vi "Surviv_io.vi"() -> ()   [LabVIEW 2021]
uses:
  <vilib>/Utility/miscctls.llb/LVPositionTypeDef.ctl
  b365312c-386e-413b-b974-73f95af02f70.vi
  <vilib>/Utility/miscctls.llb/LVComboBoxStrsAndValuesArrayTypeDef.ctl
  <vilib>/Utility/inputDevices.llb/closeMouse.vi
  <vilib>/Utility/inputDevices.llb/closeKeyboard.vi
  <vilib>/Utility/inputDevices.llb/mouseAcquire.vi
  <vilib>/Utility/inputDevices.llb/keyboardAcquire.vi
  <vilib>/Utility/file.llb/Read Delimited Spreadsheet (DBL).vi
  <vilib>/Utility/file.llb/Write Delimited Spreadsheet (DBL).vi
  <vilib>/sound2/lvsound2.llb/Sound Output Set Volume (Single).vi
panel:
  out "Data length":i32
  out "NetPlayer Commend":T1(array[cluster])
  out "My NetPlayer number":i32
  out "Connecting....":bool caption="Connecting..."
  out "NetPlayer":cluster{"Name":string, "IP Address":u32}[](array[cluster])
  in  "創建遊戲":bool
  in  "加入遊戲":bool
  out "Network Game":bool
  in  "選擇網路介面:":string(combo)="192.168.56.1"
  out "Background music":dbl
  out "Final Winner":string
  out "Enemy on 8 directions":T2
  out "Farther Bullets on 8 directions":T2
  out "Closer Bullets on 8 directions":T2
  out "Object on 8 directions":T2
  out "Closest valid target":T3
  out "Current Player HP":dbl
  out "Player HP Healing (And visibility)":i32[](array[numeric])
  out "Alive number":i32
  out "MP HP":dbl(slide) scale=0.0..290.0
  out "Input detect frequency (Hz)":dbl
  out "Sent command":T4(array[cluster])
  out "MainPlayer":T5
  out "Movement":dbl
  out "Theta":dbl
  out "Object number":i32
  out "Player Bullets Reload":i32[](array[numeric])
  out "Player Bullets":i32[](array[numeric])
  out "Frame Number":i32
  out "Player info":T6(array[cluster])
  out "Physic Engine frequency (Hz)":dbl
  out "Color 2":u32(colorbox)
  out "Color":u32(colorbox)
  out "MO ID":i32
  out "Moving Entity Position":T7(array[cluster])
  in  "進入遊戲":bool
  out "Map Entity Object Position":T8(array[cluster])
  in  "地圖:":string(combo) caption="Combo Box"
  in  "電腦代打模式:\n(Based on Machine Learning)\n(Behavior cloning)\n(Warning: High computing workload)":bool
  in  "初級電腦玩家人數:":i32 min=0 max=0 step=1
  in  "普通電腦玩家人數:":i32=1 min=0 max=19 step=1
  in  "Host IP: (Local Network)":string
  in  "玩家ID: (創建遊戲)":string
  in  "玩家ID: (加入遊戲)":string
  in  "Close (Main UI)":bool
  out "State":i32
  in  "Customized Game Button":bool
  in  "Join/Create Room Button":bool
  in  "Game Instruction Button":bool
  in  "Game Start Button":bool
  out "FPS":dbl
  in  "STOP (會卡住)":bool
  out "已加入的玩家:":string[](array[string])
  out "PlayingScene":picture
  # "若要遊玩網路遊戲，請至遊戲資料夾，目錄\\Game\\cmd\\Firewall.bat，點選\"以管理員身分執行\"，以打開防火牆設定，連線雙方均須打開請確保兩位玩家 在同一 Local Network 內 (如: 兩筆電連到同一個手機熱點)，並且在遊戲選單選擇對應的網卡介面，方可連上遊玩!"
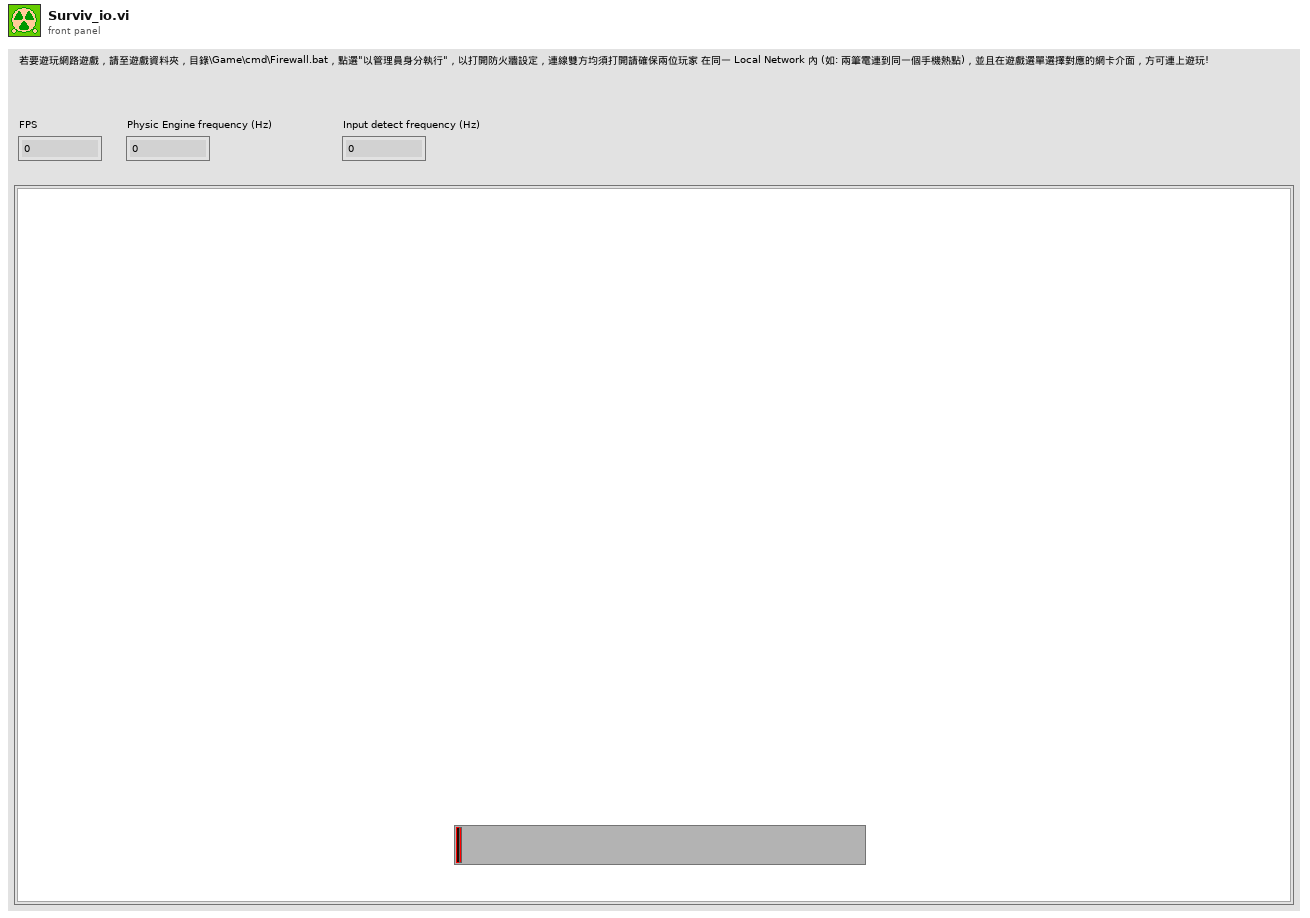
[diagram p1: front panel]
types:
  T1 = cluster{"Vector scalar":sgl, "Vector theta":sgl, "Mouse theta":sgl, "Mouse Shoot":sgl, "Reload R":sgl}[]
  T2 = cluster{"D1":dbl, "D2":dbl, "D3":dbl, "D4":dbl, "D5":dbl, "D6":dbl, "D7":dbl, "D8":dbl}
  T3 = cluster{"Theta (toward that target)":dbl, "Distance (toward that target)":dbl, "Reachable":bool}
  T4 = cluster{"X":dbl, "Y":dbl, "Object type":dbl, "Move info":dbl, "Vector scalar":dbl, "Theta":dbl}[]
  T5 = cluster{"X":dbl, "Y":dbl, "Object type":dbl, "Radius":dbl, "Width":dbl, "Height":dbl, "Theta":dbl, "HP":dbl, "R":dbl, "G":dbl, "B":dbl}
  T6 = cluster{"Kills":dbl, "Name":string, "Rank":dbl, "Who Kill Me":dbl, "After Kill":dbl}[]
  T7 = cluster{"X":dbl, "Y":dbl, "Object type":dbl, "Move info":dbl, "Vector scalar":dbl, "Vector theta":dbl}[]
  T8 = cluster{"X":dbl, "Y":dbl, "Object type":dbl, "Radius":dbl, "Width":dbl, "Height":dbl, "Theta":dbl, "HP":dbl, "R":dbl, "G":dbl, "B":dbl}[]
  T9 = typedef "LVComboBoxStrsAndValuesArrayTypeDef.ctl" = cluster{"String":string, "Value":string}[]
  T10 = enum8{"Enabled", "Disabled", "Disabled and Grayed Out"}
  T11 = cluster{"left":i16, "top":i16, "right":i16, "bottom":i16}
  T12 = typedef "LVPositionTypeDef.ctl" = cluster{"Left":i32, "Top":i32}
  T13 = enum16{"User-specified Font", "Application Font", "System Font", "Dialog Font"}
  T14 = cluster{"Font Name:":string, "Size":i16, "Strikeout?":bool, "Italic?":bool, "Underline?":bool, "Outline?":bool, "Shadow?":bool, "Bold?":bool}
  T15 = cluster{"horizontal":enum16{"left", "center", "right"}, "vertical":enum16{"top", "center", "bottom"}}
  T16 = enum16{"None", "Stacked", "Clockwise", "Counterclockwise"}
  T17 = cluster{"初級電腦玩家人數: ":i32, "普通電腦玩家人數: ":i32, "地圖:":string, "已加入的玩家:":string[]}
  T18 = typedef "Sound Output Task ID.ctl" = u32
  T19 = cluster{"Vector scalar":sgl, "Vector theta":sgl, "Mouse theta":sgl, "Mouse Shoot":sgl, "Reload R":sgl, "Reload R 2":sgl}
  T20 = cluster{dbl, "玩家ID: (加入遊戲)":string, dbl, dbl, dbl}
  T21 = cluster{"[0]":dbl, "[1]":dbl, "[2]":dbl, "[3]":dbl, "[4]":dbl, "[5]":dbl, "[6]":dbl, "[7]":dbl, "[8]":dbl, "[9]":dbl, "[10]":dbl}
  T22 = cluster{"[0]":dbl, "[1]":dbl, "[2]":dbl, "[3]":dbl, "[4]":dbl, "[5]":dbl, "[6]":dbl, "[7]":dbl, "[8]":dbl, "[9]":dbl, "[10]":dbl}[]
  T23 = cluster{"Kills":dbl, "玩家ID: (加入遊戲)":string, "Rank":dbl, "Who Kill Me":dbl, "After Kill":dbl}[]
  T24 = cluster{"X":dbl, "Y":dbl, "Object type":dbl, "Move info":dbl, "Vector scalar":dbl, "Vector theta":dbl}
  T25 = cluster{dbl, dbl, "Object type":dbl, "Move info":dbl, "Vector scalar":dbl, "Vector theta":dbl}
  T26 = cluster{"Kills":dbl, "Name":string, "Rank":dbl, "Who Kill Me":dbl, "After Kill":dbl}
  T27 = cluster{dbl, "Name":string, "Rank":dbl, "Who Kill Me":dbl, "After Kill":dbl}
  T28 = cluster{"Kills":dbl, "Name":string, "Alive number":i32, dbl, "y":dbl}
  T29 = cluster{"X":dbl, "Y":dbl, "Object type":dbl, "Radius":dbl, "Width":dbl, "Height":dbl, "Theta":dbl, dbl, "R":dbl, "G":dbl, "B":dbl}
  T30 = cluster{"New Vector Scalar":dbl, "New Vector Theta":dbl}
  T31 = cluster{dbl, dbl, "Object type":dbl, "Radius":dbl, "Width":dbl, "Height":dbl, "Move info":dbl, "HP":dbl, "R":dbl, "G":dbl, "B":dbl}
  T32 = cluster{"X":dbl, "Y":dbl, "Object type":dbl, "Radius":dbl, "y":dbl, "Height":dbl, "Theta":dbl, "HP":dbl, "R":dbl, "G":dbl, "B":dbl}
  T33 = cluster{"X":dbl, "Y":dbl, "Object type":dbl, "Radius":dbl, "y":dbl, "Height":dbl, "Theta":dbl, dbl, "R":dbl, "G":dbl, "B":dbl}
  T34 = cluster{"X":dbl, "Y":dbl, dbl, dbl, dbl, dbl, dbl, dbl, dbl, dbl, dbl}
  T35 = cluster{"X":dbl, "Y":dbl, "Object type":dbl, "Move info":dbl, "Vector scalar":dbl, "Theta":dbl}
  T36 = typedef "LVPointTypeDef.ctl" = cluster{"Horizontal":i16, "Vertical":i16}
  T37 = enum16{"0", "1", "2", "3", "4", "5", "6", "7", "8", "9", "A", "B", "C", "D", "E", "F", "G", "H", "I", "J", "K", "L", "M", "N", "O", "P", "Q", "R", "S", "T", "U", "V", "W", "X", "Y", "Z", "F1", "F2", "F3", "F4", "F5", "F6", "F7", "F8", "F9", "F10", "F11", "F12", "F13", "F14", "F15", "ADD", "BACK", "BACKSLASH", "CAPITAL", "COMMA", "DECIMAL", "DELETE", "DIVIDE", "DOWN", "END", "EQUALS", "ESCAPE", "GRAVE (`)", "HOME", "INSERT", "LBRACKET", "LCONTROL", "LEFT", "L ALT", "LSHIFT", "LWIN", "MINUS", "MULTIPLY", "NEXT", "NUMLOCK", "NUMPAD_0", "NUMPAD_1", "NUMPAD_2", "NUMPAD_3", "NUMPAD_4", "NUMPAD_5", "NUMPAD_6", "NUMPAD_7", "NUMPAD_8", "NUMPAD_9", "PAUSE", "PERIOD", "PRIOR (PG UP)", "RBRACKET", "RCONTROL", "RETURN", "RIGHT", "R ALT", "RSHIFT", "RWIN", "SCROLL", "SEMICOLON", "SLASH", "SPACE", "SUBTRACT", "TAB", "UP", "ENTER (num pad)", "' (quote)"}[]
  T38 = cluster{"Horizontal":i32, "Vertical":i32, "Scrolling":i32}
  T39 = cluster{"button 1":bool, "button 2":bool, "button 3":bool, "button 4":bool}
  T40 = typedef "LVRectTypeDef.ctl" = cluster{"Left":i16, "Top":i16, "Right":i16, "Bottom":i16}
  T41 = cluster{dbl, dbl, i32, "Mouse theta":sgl, "Vector scalar":sgl, "Vector theta":sgl}
  T42 = cluster{dbl, dbl, i32, dbl, dbl, "Mouse theta":sgl}
  T43 = cluster{"X":sgl, "Y":sgl, "Object type":sgl, "Radius":sgl, "Width":sgl, "Height":sgl, "Theta":sgl, "HP":sgl, "R":sgl, "G":sgl, "B":sgl}[]
  T44 = cluster{cluster{"X":sgl, "Y":sgl, "Object type":sgl, "Radius":sgl, "Width":sgl, "Height":sgl, "Theta":sgl, "HP":sgl, "R":sgl, "G":sgl, "B":sgl}[], "Final Winner":string, "Player info":cluster{"Kills":dbl, "Name":string, "Rank":dbl, "Who Kill Me":dbl, "After Kill":dbl}[], "Alive number":i32, i32, i32, i32}
  T45 = cluster{"Vector scalar":sgl, "Vector theta":sgl, "Mouse theta":sgl, "Mouse Shoot":sgl, "Reload R":sgl}
  T46 = cluster{dbl, "Theta":dbl, dbl, "f":dbl, "f":dbl, "My NetPlayer number":i32}
  T47 = cluster{sgl, "Theta":sgl, sgl, "f":sgl, "f":sgl, "My NetPlayer number":sgl}
  T48 = cluster{cluster{"X":sgl, "Y":sgl, "Object type":sgl, "Radius":sgl, "Width":sgl, "Height":sgl, "Theta":sgl, "HP":sgl, "R":sgl, "G":sgl, "B":sgl}[], "Final Winner":string, "Player info":cluster{"Kills":dbl, "Name":string, "Rank":dbl, "Who Kill Me":dbl, "After Kill":dbl}[], "Alive number":i32, "element":i32, "element":i32, "element":i32}
  T49 = cluster{"X":sgl, "Y":sgl, "Object type":sgl, "Radius":sgl, "Width":sgl, "Height":sgl, "Theta":sgl, "HP":sgl, "R":sgl, "G":sgl, "B":sgl}
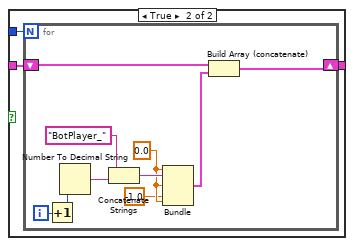
[diagram p4: hidden frame]
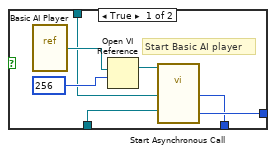
[diagram p6: hidden frame]
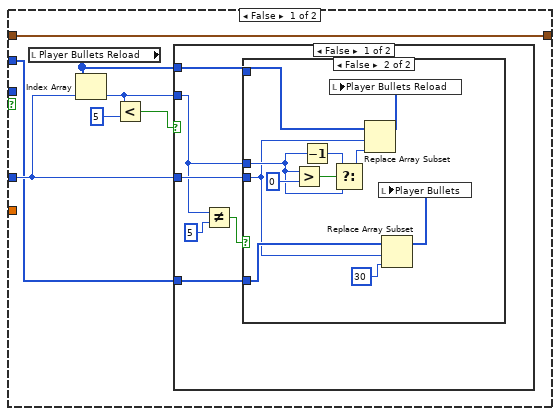
[diagram p11: hidden frame]
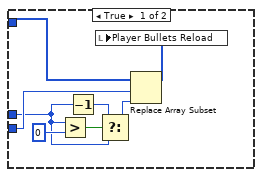
[diagram p12: hidden frame]
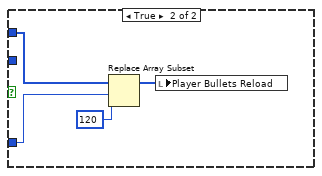
[diagram p13: hidden frame]
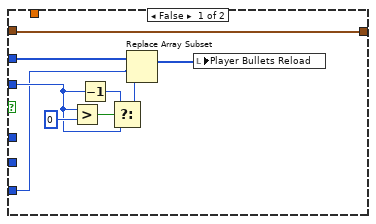
[diagram p14: hidden frame]
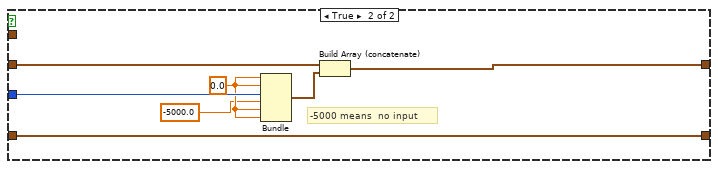
[diagram p15: hidden frame]
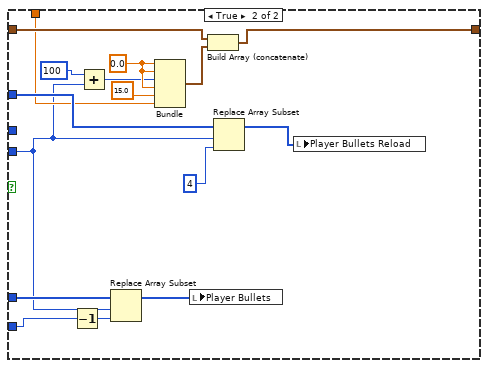
[diagram p18: hidden frame]
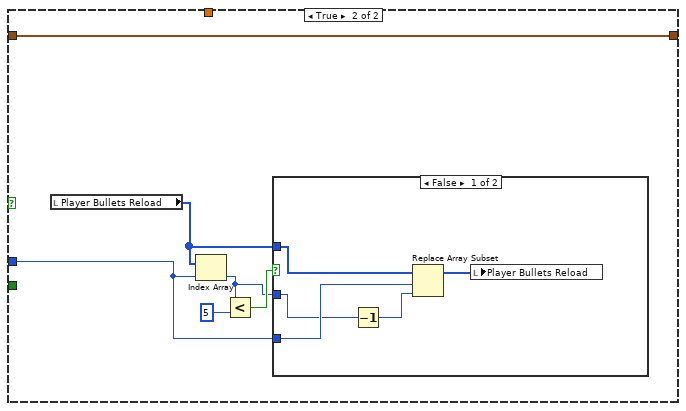
[diagram p19: hidden frame]
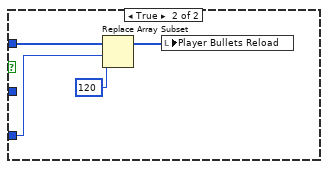
[diagram p20: hidden frame]
diagram:
  # "Stop still stuck as game started.\nUnsolved, but it doesn't matter.\nThis problem is from high workloads\nof Front Panel"
  # "Test color"
  n1 = flat-sequence {
    tunnel: [w13] -> w2
    tunnel: [w620] -> w1
    frame #0 {
      w47 = ""
      w13 = 1.0 ("Background music")
      # "Main UI and the whole game initialization."
      # "Initialization"
      n2 = String To IP() -> (0:w22:u32[])  [unwired: 1 in]
      n3 = for {
        tunnel: w22 -> [w65] mode=indexing
        shift-right: [w67] -> w21
        shift-left: T9 [] ("Strings And Values []") -> [w68]
        tunnel: [w63] -> w20
        n4 = IP To String(1:TRUE ("dot notation? (F)"), 2:w65) -> (0:w63:string)
        n5 = Bundle("name"=w63, "name"=w63) -> (w64:cluster{"name":string, "name":string})  [unwired: 1 in]
        n6 = Build Array (concatenate)(w68, w64) -> (w67:T9)
      }
      n7 = local write "NetPlayer Commend"(T1 [] ("NetPlayer Commend")) -> ()
      n8 = property on="電腦代打模式:\n(Based on Machine Learning)\n(Behavior cloning)\n(Warning: High computing workload)" class="Bool (strict)"("Visible"=FALSE) -> ()  [unwired: 2 in, 2 out]
      n9 = property on="普通電腦玩家人數:" class="DigNum (strict)"("Visible"=FALSE) -> ()  [unwired: 2 in, 2 out]
      n10 = property on="初級電腦玩家人數:" class="DigNum (strict)"("Visible"=FALSE) -> ()  [unwired: 2 in, 2 out]
      n11 = property on="地圖:" class="CmbBox"("Visible"=FALSE) -> ()  [unwired: 2 in, 2 out]
      n12 = local write "STOP (會卡住)"(FALSE ("Visible")) -> ()
      n13 = property on="選擇網路介面:" class="CmbBox"("Strings And Values[]"=w21) -> ()  [unwired: 2 in, 2 out]
      n14 = local write "選擇網路介面:"(w20) -> ()
      n15 = local write "Network Game"(FALSE ("Network Game")) -> ()
      n16 = local write "Connecting...."(FALSE ("Connecting....")) -> ()
      n17 = property on="已加入的玩家:" class="Arr (strict)"("Visible"=FALSE) -> ()  [unwired: 2 in, 2 out]
      n18 = property on="選擇網路介面:" class="CmbBox"("Visible"=FALSE) -> ()  [unwired: 2 in, 2 out]
      n19 = property on="加入遊戲" class="Bool"("Visible"=FALSE) -> ()  [unwired: 2 in, 2 out]
      n20 = local write "玩家ID: (加入遊戲)"(w47) -> ()
      n21 = property on="創建遊戲" class="Bool"("Visible"=FALSE) -> ()  [unwired: 2 in, 2 out]
      n22 = local write "玩家ID: (創建遊戲)"(w47) -> ()
      n23 = property on="Connecting...." class="Bool (strict)"("Visible"=FALSE) -> ()  [unwired: 2 in, 2 out]
      n24 = property on="Game Start Button" class="Bool"("Visible"=TRUE) -> ()  [unwired: 2 in, 2 out]
      n25 = property on="Join/Create Room Button" class="Bool"("Visible"=TRUE) -> ()  [unwired: 2 in, 2 out]
      n26 = property on="Customized Game Button" class="Bool"("Visible"=TRUE) -> ()  [unwired: 2 in, 2 out]
      n27 = property on="Game Instruction Button" class="Bool"("Visible"=TRUE) -> ()  [unwired: 2 in, 2 out]
      n28 = property on="MP HP" class="Slide (strict)"("Scale.Visible"=FALSE) -> ()  [unwired: 2 in, 2 out]
      n29 = property on="MP HP" class="Slide (strict)"("Visible"=FALSE) -> ()  [unwired: 2 in, 2 out]
      n30 = property on="進入遊戲" class="Bool"("Visible"=FALSE) -> ()  [unwired: 2 in, 2 out]
      n31 = property on="玩家ID: (創建遊戲)" class="Str"("Visible"=FALSE) -> ()  [unwired: 2 in, 2 out]
      n32 = property on="Host IP: (Local Network)" class="Str"("Visible"=FALSE) -> ()  [unwired: 2 in, 2 out]
      n33 = property on="玩家ID: (加入遊戲)" class="Str"("Visible"=FALSE) -> ()  [unwired: 2 in, 2 out]
      n34 = property on="Close (Main UI)" class="Bool (strict)"("Visible"=FALSE) -> ()  [unwired: 2 in, 2 out]
      n35 = local write "MP HP"(300.0 ("MP HP")) -> ()
      n36 = local write "初級電腦玩家人數:"(0 ("普通電腦玩家人數:")) -> ()
      n37 = local write "普通電腦玩家人數:"(10 ("普通電腦玩家人數:")) -> ()
      n38 = local write "地圖:"("Map 1" ("地圖:")) -> ()
      n39 = Current VI's Path() -> (path=w62:path)
      n40 = Strip Path(path=w62) -> (stripped path=w61:path)  [unwired: 1 out]
      n41 = Path To String(path=w61) -> (string=w60:string)
      n42 = property on="初級電腦玩家人數:" class="DigNum (strict)"("DisabledEnum"=T10."Enabled" ("Disabled")) -> ()  [unwired: 2 in, 2 out]
      n43 = property on="普通電腦玩家人數:" class="DigNum (strict)"("DisabledEnum"=T10."Enabled" ("Disabled")) -> ()  [unwired: 2 in, 2 out]
      n44 = property on="地圖:" class="CmbBox"("DisabledEnum"=T10."Enabled" ("Disabled")) -> ()  [unwired: 2 in, 2 out]
      n45 = property on="普通電腦玩家人數:" class="DigNum (strict)"("Maximum"=19 ("x")) -> ()  [unwired: 2 in, 2 out]
      n46 = Concatenate Strings("Start-Process cmd -ArgumentList \"/c `\"`\"" ("command line"), w60, "\\cmd\\Firewall.bat`\"`\"\" -Verb runAs" ("string")) -> ()  [unwired: 1 out]
      n47 = local write "Alive number"(100 ("Alive number")) -> ()
      n48 = property on="Map Entity Object Position" class="Arr (strict)"("Visible"=FALSE) -> ()  [unwired: 2 in, 2 out]
      n49 = local write "PlayingScene"(picture data[5B] ("picture")) -> ()
      n50 = property on="State" class="DigNum (strict)"("Visible"=FALSE) -> ()  [unwired: 2 in, 2 out]
      n51 = local write "State"(0 ("State")) -> ()
      n52 = Wait (ms)(milliseconds to wait=u32 5) -> ()  [unwired: 1 out]
      "MO ID" <- 0 ("MO ID")
      "Background music" <- w13
      "已加入的玩家:" <- string[] [] ("已加入的玩家:")
      "NetPlayer" <- cluster{"Name":string, "IP Address":u32}[] [] ("NetPlayer")
    }
    frame #1 {
      n53 = while {
        shift-right: [w70] -> _
        shift-left: _ -> [w69]
        stop <- w74 stop-if-true
        # "The Main Graphic User Interface"
        n54 = local read "State"() -> (w76:i32)
        n55 = call <vilib>:"Draw Rectangle.vi"("picture"=picture data[5B], "rect"=T11 {"left"=0, "top"=0, "right"=1280, "bottom"=720}, "fill?(F)"=TRUE, "color(black)"=u32 11861920) -> ("new picture"=w75:picture)  [unwired: 5 in]
        n56 = call <vilib>:"High Resolution Relative Seconds.vi"() -> ("relative seconds"=w82:dbl)
        n57 = feedback-in #1(w82) -> ()
        n58 = feedback #1(u32 0 ("millisecond timer value")) -> (w83:dbl)
        n59 = case shown="5" w76 {
          tunnel: w75 -> [w154 w180 w217 w354 w445 w496 w549]
          tunnel: [w153 w181 w218 w355 w446 w497 w550] -> w72
          tunnel: [_ _ _ w334 w427 w483 w540] -> w73
          tunnel: [_ _ w200 w335 w432 _ _] -> w70
          tunnel: w69 -> [_ _ _ w341 w433 _ _]
          frame 0, Default {
            n60 = call <vilib>:"Draw Text at Point.vi"("text orientation"=T16."None", "[user-specified font]"=T14 {"Font Name:"="Arial", "Size"=96, "Strikeout?"=FALSE, "Italic?"=FALSE, "Underline?"=FALSE, "Outline?"=FALSE, "Shadow?"=FALSE, "Bold?"=FALSE}, "text color(black)"=u32 0, "desired font(Application)"=T13."User-specified Font", "text"="Surviv.io", "alignment(left, top)"=T15 {"horizontal"=enum."center", "vertical"=enum."top"}, "origin"=cluster{"x":i16, "y":i16} {"x"=640, "y"=80}, "picture"=w154) -> ("new picture"=w158:picture)  [unwired: 2 in, 1 out]
            n61 = call <vilib>:"Draw Text at Point.vi"("text orientation"=T16."None", "[user-specified font]"=T14 {"Font Name:"="Arial", "Size"=36, "Strikeout?"=FALSE, "Italic?"=FALSE, "Underline?"=FALSE, "Outline?"=FALSE, "Shadow?"=FALSE, "Bold?"=FALSE}, "text color(black)"=u32 16716306, "desired font(Application)"=T13."User-specified Font", "text"="Unofficial Version", "alignment(left, top)"=T15 {"horizontal"=enum."center", "vertical"=enum."top"}, "origin"=cluster{"x":i16, "y":i16} {"x"=800, "y"=180}, "picture"=w158) -> ("new picture"=w157:picture)  [unwired: 2 in, 1 out]
            n62 = call <vilib>:"Draw Text at Point.vi"("text"="All rights reserved by 113550153, 113550099", "origin"=cluster{"x":i16, "y":i16} {"x"=1015, "y"=695}, "picture"=w157) -> ("new picture"=w153:picture)  [unwired: 7 in, 1 out]
          }
          frame 2 {
            n63 = call <vilib>:"Draw Rectangle.vi"("picture"=w180, "rect"=T11 {"left"=180, "top"=30, "right"=1100, "bottom"=690}, "fill?(F)"=TRUE, "color(black)"=u32 13816530) -> ("new picture"=w174:picture)  [unwired: 5 in]
            n64 = call <vilib>:"Draw Rectangle.vi"("picture"=w174, "rect"=T11 {"left"=180, "top"=30, "right"=1100, "bottom"=690}, "color(black)"=u32 0) -> ("new picture"=w173:picture)  [unwired: 6 in]
            n65 = call <vilib>:"Draw Text at Point.vi"("text orientation"=T16."None", "[user-specified font]"=T14 {"Font Name:"="Arial", "Size"=48, "Strikeout?"=FALSE, "Italic?"=FALSE, "Underline?"=FALSE, "Outline?"=FALSE, "Shadow?"=FALSE, "Bold?"=FALSE}, "text color(black)"=u32 0, "desired font(Application)"=T13."User-specified Font", "text"="遊戲說明", "alignment(left, top)"=T15 {"horizontal"=enum."center", "vertical"=enum."top"}, "origin"=cluster{"x":i16, "y":i16} {"x"=640, "y"=80}, "picture"=w173) -> ("new picture"=w185:picture)  [unwired: 2 in, 1 out]
            n66 = call <vilib>:"Draw Text at Point.vi"("text orientation"=T16."None", "[user-specified font]"=T14 {"Font Name:"="Arial", "Size"=36, "Strikeout?"=FALSE, "Italic?"=FALSE, "Underline?"=FALSE, "Outline?"=FALSE, "Shadow?"=FALSE, "Bold?"=FALSE}, "text color(black)"=u32 0, "desired font(Application)"=T13."User-specified Font", "text"="WASD                      |                 操作角色移動方向\n\n滑鼠                         |                 控制角色瞄準方向\n\n滑鼠右鍵點擊         |                 射擊\n\nR                               |                 換彈\n\n祝您體驗愉快!", "alignment(left, top)"=T15 {"horizontal"=enum."left", "vertical"=enum."top"}, "origin"=cluster{"x":i16, "y":i16} {"x"=240, "y"=210}, "picture"=w185) -> ("new picture"=w184:picture)  [unwired: 2 in, 1 out]
            n67 = call <vilib>:"Draw Text at Point.vi"("text"="All rights reserved by 113550153, 113550099", "origin"=cluster{"x":i16, "y":i16} {"x"=1015, "y"=695}, "picture"=w184) -> ("new picture"=w181:picture)  [unwired: 7 in, 1 out]
          }
          frame 3 {
            n68 = call <vilib>:"Draw Rectangle.vi"("picture"=w217, "rect"=T11 {"left"=180, "top"=30, "right"=1100, "bottom"=690}, "fill?(F)"=TRUE, "color(black)"=u32 13816530) -> ("new picture"=w211:picture)  [unwired: 5 in]
            n69 = call <vilib>:"Draw Rectangle.vi"("picture"=w211, "rect"=T11 {"left"=180, "top"=30, "right"=1100, "bottom"=690}, "color(black)"=u32 0) -> ("new picture"=w207:picture)  [unwired: 6 in]
            n70 = call <vilib>:"Draw Rectangle.vi"("picture"=w207, "rect"=T11 {"left"=180, "top"=30, "right"=640, "bottom"=580}, "color(black)"=u32 0) -> ("new picture"=w202:picture)  [unwired: 6 in]
            n71 = call <vilib>:"Draw Rectangle.vi"("picture"=w202, "rect"=T11 {"left"=180, "top"=30, "right"=1100, "bottom"=580}, "color(black)"=u32 0) -> ("new picture"=w203:picture)  [unwired: 6 in]
            n72 = call <vilib>:"Draw Text at Point.vi"("text orientation"=T16."None", "[user-specified font]"=T14 {"Font Name:"="Arial", "Size"=48, "Strikeout?"=FALSE, "Italic?"=FALSE, "Underline?"=FALSE, "Outline?"=FALSE, "Shadow?"=FALSE, "Bold?"=FALSE}, "text color(black)"=u32 0, "desired font(Application)"=T13."User-specified Font", "text"="加入遊戲", "alignment(left, top)"=T15 {"horizontal"=enum."center", "vertical"=enum."top"}, "origin"=cluster{"x":i16, "y":i16} {"x"=400, "y"=120}, "picture"=w203) -> ("new picture"=w221:picture)  [unwired: 2 in, 1 out]
            n73 = call <vilib>:"Draw Text at Point.vi"("text orientation"=T16."None", "[user-specified font]"=T14 {"Font Name:"="Arial", "Size"=48, "Strikeout?"=FALSE, "Italic?"=FALSE, "Underline?"=FALSE, "Outline?"=FALSE, "Shadow?"=FALSE, "Bold?"=FALSE}, "text color(black)"=u32 0, "desired font(Application)"=T13."User-specified Font", "text"="創建遊戲", "alignment(left, top)"=T15 {"horizontal"=enum."center", "vertical"=enum."top"}, "origin"=cluster{"x":i16, "y":i16} {"x"=880, "y"=120}, "picture"=w221) -> ("new picture"=w220:picture)  [unwired: 2 in, 1 out]
            n74 = event shown="[1] \"創建遊戲\": Value Change" {
              selector: _ -> [_ _ _]
              dyn-events: _ -> [_ _ _]
              timeout: 1 -> [_ _ _]
              tunnel: [_ w236 w283] -> w200
              event Timeout {
                n75 = event-data() -> ()  [unwired: 1 in, 3 out]
              }
              event "創建遊戲": Value Change {
                n76 = event-data() -> ()  [unwired: 1 in, 1 out]
                n77 = local write "電腦代打模式:\n(Based on Machine Learning)\n(Behavior cloning)\n(Warning: High computing workload)"(FALSE ("電腦代打模式:\n(Based on Machine Learning)\n(Behavior cloning)\n(Warning: High computing workload)")) -> ()
                n78 = property on="創建遊戲" class="Bool"("Visible"=FALSE) -> ()  [unwired: 2 in, 2 out]
                n79 = property on="加入遊戲" class="Bool"("Visible"=FALSE) -> ()  [unwired: 2 in, 2 out]
                n80 = property on="Close (Main UI)" class="Bool (strict)"("Visible"=FALSE) -> ()  [unwired: 2 in, 2 out]
                n81 = property on="進入遊戲" class="Bool"("Visible"=TRUE) -> ()  [unwired: 2 in, 2 out]
                n82 = property on="已加入的玩家:" class="Arr (strict)"("Visible"=TRUE) -> ()  [unwired: 2 in, 2 out]
                n83 = property on="Host IP: (Local Network)" class="Str"("Visible"=FALSE) -> ()  [unwired: 2 in, 2 out]
                n84 = property on="初級電腦玩家人數:" class="DigNum (strict)"("Position"=T12 {"Left"=36, "Top"=-154}) -> ()  [unwired: 2 in, 2 out]
                n85 = property on="普通電腦玩家人數:" class="DigNum (strict)"("Position"=T12 {"Left"=36, "Top"=-60}) -> ()  [unwired: 2 in, 2 out]
                n86 = property on="地圖:" class="CmbBox"("Position"=T12 {"Left"=54, "Top"=48}) -> ()  [unwired: 2 in, 2 out]
                n87 = property on="玩家ID: (加入遊戲)" class="Str"("Visible"=FALSE) -> ()  [unwired: 2 in, 2 out]
                n88 = property on="玩家ID: (創建遊戲)" class="Str"("Visible"=FALSE) -> ()  [unwired: 2 in, 2 out]
                n89 = property on="選擇網路介面:" class="CmbBox"("Visible"=FALSE) -> ()  [unwired: 2 in, 2 out]
                n90 = local read "已加入的玩家:"() -> (w253:string[])
                n91 = local write "玩家ID: (加入遊戲)"("玩家ID: (創建遊戲)") -> ()
                n92 = property on="初級電腦玩家人數:" class="DigNum (strict)"("Visible"=TRUE) -> ()  [unwired: 2 in, 2 out]
                n93 = property on="普通電腦玩家人數:" class="DigNum (strict)"("Visible"=TRUE) -> ()  [unwired: 2 in, 2 out]
                n94 = property on="地圖:" class="CmbBox"("Visible"=TRUE) -> ()  [unwired: 2 in, 2 out]
                n95 = Equal?(x="玩家ID: (創建遊戲)", y="") -> (x = y?=w255:bool)
                n96 = local read "選擇網路介面:"() -> (w239:string)
                n97 = case shown="True" w255 {
                  tunnel: "玩家ID: (創建遊戲)" -> [w264 _]
                  tunnel: [w264 w265] -> w250
                  frame False {
                  }
                  frame True {
                    n98 = Random Number (0-1)() -> (number: 0 to 1=w271:dbl)
                    n99 = Multiply(x=w271, y=9999.0) -> (x*y=w268:dbl)
                    n100 = To Long Integer(number=w268) -> (32bit integer=w266:i32)
                    n101 = Number To Decimal String(number=w266) -> (decimal integer string=w267:string)  [unwired: 1 in]
                    n102 = Concatenate Strings("無名氏_", w267) -> (w265:string)
                  }
                }
                n103 = Insert Into Array(array=w253, index=0, new element=w250) -> (w252:string[])
                n104 = local write "State"(5 ("State")) -> ()
                n105 = local write "已加入的玩家:"(w252) -> ()
                n106 = property on="進入遊戲" class="Bool"("Position"=T12 {"Left"=108, "Top"=192}) -> ()  [unwired: 2 in, 2 out]
                n107 = String To IP(1:w239) -> (0:w238:u32)
                n108 = UDP Open(7:w238, 11:u16 52023 ("port")) -> (port=w236:refnum<k16>)  [unwired: 3 in, 2 out]
              }
              event "加入遊戲": Value Change {
                n109 = event-data() -> ()  [unwired: 1 in, 1 out]
                n110 = local read "玩家ID: (加入遊戲)"() -> (w292:string)
                n111 = local read "Host IP: (Local Network)"() -> (w295:string)
                n112 = Equal?(x=w292, y="") -> (x = y?=w293:bool)
                n113 = property on="Connecting...." class="Bool (strict)"("Caption.Text"="Connecting...") -> ()  [unwired: 2 in, 2 out]
                n114 = case shown="True" w293 {
                  tunnel: w292 -> [w326 _]
                  tunnel: [w326 w327] -> w290
                  frame False {
                  }
                  frame True {
                    n115 = Random Number (0-1)() -> (number: 0 to 1=w333:dbl)
                    n116 = Multiply(x=w333, y=9999.0) -> (x*y=w330:dbl)
                    n117 = To Long Integer(number=w330) -> (32bit integer=w328:i32)
                    n118 = Number To Decimal String(number=w328) -> (decimal integer string=w329:string)  [unwired: 1 in]
                    n119 = Concatenate Strings("無名氏_", w329) -> (w327:string)
                  }
                }
                n120 = local write "Connecting...."(FALSE ("Connecting....")) -> ()
                n121 = String To IP(1:w295) -> (0:w278:u32)
                n122 = property on="Connecting...." class="Bool (strict)"("Visible"=TRUE) -> ()  [unwired: 2 in, 2 out]
                n123 = local read "選擇網路介面:"() -> (w298:string)
                n124 = String To IP(1:w298) -> (0:w279:u32)
                n125 = Equal?(x=w279, y=w278) -> (x = y?=w280:bool)
                n126 = Select(t=u32 0, s=w280, f=w278) -> (s? t:f=w277:u32)
                n127 = UDP Open(7:w279, 11:u16 52023 ("port")) -> (port=w296:refnum<k16>)  [unwired: 3 in, 2 out]
                n128 = UDP Write(address=w277, port or service name=u16 52023, connection ID=w296, data in=w290) -> (error out=w281:errorcluster, 3:w289:refnum<k16>)  [unwired: 2 in]
                n129 = UDP Read(connection ID=w289, timeout ms (25000)=5000, 8:w281) -> (data out=w275:string, error out=w288:errorcluster, 3:w284:refnum<k16>)  [unwired: 1 in, 2 out]
                n130 = case shown="No Error" w288 {
                  tunnel: w284 -> [w301 w321]
                  tunnel: [w301 _] -> w283
                  frame No Error {
                    n131 = local write "電腦代打模式:\n(Based on Machine Learning)\n(Behavior cloning)\n(Warning: High computing workload)"(FALSE ("電腦代打模式:\n(Based on Machine Learning)\n(Behavior cloning)\n(Warning: High computing workload)")) -> ()
                    n132 = property on="Connecting...." class="Bool (strict)"("Visible"=FALSE) -> ()  [unwired: 2 in, 2 out]
                    n133 = local write "State"(6 ("State")) -> ()
                    n134 = property on="玩家ID: (加入遊戲)" class="Str"("Visible"=FALSE) -> ()  [unwired: 2 in, 2 out]
                    n135 = property on="選擇網路介面:" class="CmbBox"("Visible"=FALSE) -> ()  [unwired: 2 in, 2 out]
                    n136 = property on="初級電腦玩家人數:" class="DigNum (strict)"("Visible"=TRUE) -> ()  [unwired: 2 in, 2 out]
                    n137 = property on="普通電腦玩家人數:" class="DigNum (strict)"("Visible"=TRUE) -> ()  [unwired: 2 in, 2 out]
                    n138 = property on="加入遊戲" class="Bool"("Visible"=FALSE) -> ()  [unwired: 2 in, 2 out]
                    n139 = property on="進入遊戲" class="Bool"("Position"=T12 {"Left"=108, "Top"=192}) -> ()  [unwired: 2 in, 2 out]
                    n140 = property on="初級電腦玩家人數:" class="DigNum (strict)"("Position"=T12 {"Left"=36, "Top"=-154}) -> ()  [unwired: 2 in, 2 out]
                    n141 = property on="普通電腦玩家人數:" class="DigNum (strict)"("Position"=T12 {"Left"=36, "Top"=-60}) -> ()  [unwired: 2 in, 2 out]
                    n142 = property on="地圖:" class="CmbBox"("Position"=T12 {"Left"=54, "Top"=48}) -> ()  [unwired: 2 in, 2 out]
                    n143 = property on="已加入的玩家:" class="Arr (strict)"("Visible"=TRUE) -> ()  [unwired: 2 in, 2 out]
                    n144 = property on="創建遊戲" class="Bool"("Visible"=FALSE) -> ()  [unwired: 2 in, 2 out]
                    n145 = property on="地圖:" class="CmbBox"("Visible"=TRUE) -> ()  [unwired: 2 in, 2 out]
                    n146 = property on="Close (Main UI)" class="Bool (strict)"("Visible"=FALSE) -> ()  [unwired: 2 in, 2 out]
                    n147 = property on="Host IP: (Local Network)" class="Str"("Visible"=FALSE) -> ()  [unwired: 2 in, 2 out]
                    n148 = property on="初級電腦玩家人數:" class="DigNum (strict)"("DisabledEnum"=T10."Disabled" ("Disabled")) -> ()  [unwired: 2 in, 2 out]
                    n149 = property on="普通電腦玩家人數:" class="DigNum (strict)"("DisabledEnum"=T10."Disabled" ("Disabled")) -> ()  [unwired: 2 in, 2 out]
                    n150 = property on="地圖:" class="CmbBox"("DisabledEnum"=T10."Disabled" ("Disabled")) -> ()  [unwired: 2 in, 2 out]
                    n151 = property on="玩家ID: (創建遊戲)" class="Str"("Visible"=FALSE) -> ()  [unwired: 2 in, 2 out]
                  }
                  frame Error {
                    n152 = flat-sequence {
                      frame #0 {
                        n153 = local write "Connecting...."(TRUE ("Connecting....")) -> ()
                        n154 = Wait (ms)(milliseconds to wait=u32 500) -> ()  [unwired: 1 out]
                        n155 = property on="Connecting...." class="Bool (strict)"("Caption.Text"="Connect Failed !") -> ()  [unwired: 2 in, 2 out]
                      }
                      frame #1 {
                        n156 = property on="Connecting...." class="Bool (strict)"("Visible"=FALSE) -> ()  [unwired: 2 in, 2 out]
                      }
                    }
                    n157 = UDP Close(connection ID=w321) -> ()  [unwired: 1 in, 2 out]
                  }
                }
                n158 = Unflatten From String(type=0, binary string=w275) -> (value=w274:i32, error out=w272:errorcluster)  [unwired: 3 in, 1 out]
                n159 = Unbundle(w272) -> ()  [unwired: 3 out]
                n160 = local write "My NetPlayer number"(w274) -> ()
              }
            }
            n161 = call <vilib>:"Draw Text at Point.vi"("text"="All rights reserved by 113550153, 113550099", "origin"=cluster{"x":i16, "y":i16} {"x"=1015, "y"=695}, "picture"=w220) -> ("new picture"=w218:picture)  [unwired: 7 in, 1 out]
          }
          frame 5 {
            n162 = local read "NetPlayer"() -> (w340:cluster{"Name":string, "IP Address":u32}[])
            n163 = call <vilib>:"Draw Rectangle.vi"("picture"=w354, "rect"=T11 {"left"=180, "top"=30, "right"=1100, "bottom"=690}, "fill?(F)"=TRUE, "color(black)"=u32 13816530) -> ("new picture"=w348:picture)  [unwired: 5 in]
            n164 = Array Size(array=w340) -> (size(s)=w339:i32)
            n165 = Less?(x=w339, y=9) -> (x < y?=w337:bool)
            n166 = case shown="True" w337 {
              tunnel: w341 -> [w375 w381]
              tunnel: [w375 w376] -> w335
              frame False {
              }
              frame True {
                n167 = UDP Read(connection ID=w381, timeout ms (25000)=16) -> (data out=w378:string, error out=w379:errorcluster, 3:w376:refnum<k16>, 6:w377:u32)  [unwired: 2 in, 1 out]
                n168 = case shown="No Error" w379 {
                  tunnel: w378 -> [w386 _]
                  tunnel: w377 -> [w388 _]
                  tunnel: w376 -> [w392 _]
                  frame No Error {
                    n169 = local read "已加入的玩家:"() -> (w382:string[])
                    n170 = Array Size(array=w382) -> (size(s)=w384:i32)
                    n171 = local read "NetPlayer"() -> (w390:cluster{"Name":string, "IP Address":u32}[])
                    n172 = Bundle("data out"=w386, "address"=w388) -> (w387:cluster{"data out":string, "address":u32})  [unwired: 1 in]
                    n173 = Flatten To String(anything=w384) -> (data string=w385:string)  [unwired: 3 in, 2 out]
                    n174 = Build Array (concatenate)(w382, w386) -> (w383:string[])
                    n175 = Build Array (concatenate)(w390, w387) -> (w389:cluster{"data out":string, "address":u32}[])
                    n176 = UDP Write(address=w388, port or service name=u16 52023, connection ID=w392, data in=w385) -> ()  [unwired: 2 in, 2 out]
                    n177 = local write "已加入的玩家:"(w383) -> ()
                    n178 = local write "NetPlayer"(w389) -> ()
                  }
                  frame Error {
                  }
                }
              }
            }
            n179 = call <vilib>:"Draw Rectangle.vi"("picture"=w348, "rect"=T11 {"left"=180, "top"=30, "right"=1100, "bottom"=690}, "color(black)"=u32 0) -> ("new picture"=w344:picture)  [unwired: 6 in]
            n180 = call <vilib>:"Draw Rectangle.vi"("picture"=w344, "rect"=T11 {"left"=180, "top"=30, "right"=1100, "bottom"=120}, "color(black)"=u32 0) -> ("new picture"=w345:picture)  [unwired: 6 in]
            n181 = event shown="[1] \"進入遊戲\": Value Change" {
              selector: _ -> [_ _]
              dyn-events: _ -> [_ _]
              timeout: 1 -> [_ _]
              tunnel: w335 -> [_ w402]
              tunnel: [_ TRUE ("Visible")] -> w334
              event Timeout {
                n182 = event-data() -> ()  [unwired: 1 in, 3 out]
                n183 = local read "普通電腦玩家人數:"() -> (w395:i32)
                n184 = Subtract(x=10, y=w395) -> (x-y=w396:i32)
                n185 = property on="普通電腦玩家人數:" class="DigNum (strict)"("Maximum"=10 ("x")) -> ()  [unwired: 2 in, 2 out]
                n186 = property on="初級電腦玩家人數:" class="DigNum (strict)"("Maximum"=w396) -> ()  [unwired: 2 in, 2 out]
              }
              event "進入遊戲": Value Change {
                n187 = event-data() -> ()  [unwired: 1 in, 1 out]
                n188 = local read "NetPlayer"() -> (w400:cluster{"Name":string, "IP Address":u32}[])
                n189 = Array Size(array=w400) -> (size(s)=w399:i32)
                n190 = property on="已加入的玩家:" class="Arr (strict)"("Visible"=FALSE) -> ()  [unwired: 2 in, 2 out]
                n191 = property on="普通電腦玩家人數:" class="DigNum (strict)"("Visible"=FALSE) -> ()  [unwired: 2 in, 2 out]
                n192 = Not Equal To 0?(x=w399) -> (x != 0?=w398:bool)
                n193 = property on="進入遊戲" class="Bool"("Visible"=FALSE) -> ()  [unwired: 2 in, 2 out]
                n194 = case shown="True" w398 {
                  tunnel: w400 -> [_ w411]
                  tunnel: w402 -> [w408 w410]
                  frame False {
                    n195 = UDP Close(connection ID=w408) -> ()  [unwired: 1 in, 2 out]
                  }
                  frame True {
                    n196 = for {
                      tunnel: w411 -> [w414] mode=indexing
                      tunnel: w410 -> [w413]
                      tunnel: [w412] -> w409
                      n197 = for {
                        N: 5 -> [_]
                        tunnel: w414 -> [w425]
                        tunnel: w413 -> [w426]
                        tunnel: [w421] -> w412
                        w416 = -1
                        n198 = Bundle(w416, w416, "", "已加入的玩家:"=string[] []) -> (w418:cluster{i32, i32, string, "已加入的玩家:":string[]})  [unwired: 1 in]
                        n199 = Unbundle(w425) -> ("IP Address"=w424:u32)  [unwired: 1 out]
                        n200 = Flatten To String(anything=w418) -> (data string=w422:string)  [unwired: 3 in, 2 out]
                        n201 = Wait (ms)(milliseconds to wait=u32 2) -> ()  [unwired: 1 out]
                        n202 = UDP Write(address=w424, port or service name=u16 52023, connection ID=w426, data in=w422) -> (3:w421:refnum<k16>)  [unwired: 2 in, 1 out]
                      }
                    }
                    n203 = UDP Close(connection ID=w409) -> ()  [unwired: 1 in, 2 out]
                  }
                }
                n204 = local write "Network Game"(FALSE ("Network Game")) -> ()
                n205 = property on="地圖:" class="CmbBox"("Visible"=FALSE) -> ()  [unwired: 2 in, 2 out]
                n206 = property on="初級電腦玩家人數:" class="DigNum (strict)"("Visible"=FALSE) -> ()  [unwired: 2 in, 2 out]
              }
            }
            n207 = call <vilib>:"Draw Text at Point.vi"("text orientation"=T16."None", "[user-specified font]"=T14 {"Font Name:"="Arial", "Size"=48, "Strikeout?"=FALSE, "Italic?"=FALSE, "Underline?"=FALSE, "Outline?"=FALSE, "Shadow?"=FALSE, "Bold?"=FALSE}, "text color(black)"=u32 0, "desired font(Application)"=T13."User-specified Font", "text"="等待遊戲開始...", "alignment(left, top)"=T15 {"horizontal"=enum."center", "vertical"=enum."top"}, "origin"=cluster{"x":i16, "y":i16} {"x"=640, "y"=50}, "picture"=w345) -> ("new picture"=w342:picture)  [unwired: 2 in, 1 out]
            n208 = call <vilib>:"Draw Text at Point.vi"("text"="All rights reserved by 113550153, 113550099", "origin"=cluster{"x":i16, "y":i16} {"x"=1015, "y"=695}, "picture"=w342) -> ("new picture"=w355:picture)  [unwired: 7 in, 1 out]
            n209 = local read "NetPlayer"() -> (w336:cluster{"Name":string, "IP Address":u32}[])
            n210 = for {
              tunnel: w336 -> [w374] mode=indexing
              tunnel: w335 -> [w372]
              n211 = local read "初級電腦玩家人數:"() -> (w368:i32)
              n212 = local read "普通電腦玩家人數:"() -> (w367:i32)
              n213 = local read "已加入的玩家:"() -> (w369:string[])
              n214 = Unbundle(w374) -> ("IP Address"=w371:u32)  [unwired: 1 out]
              n215 = local read "地圖:"() -> (w366:string)
              n216 = Bundle("初級電腦玩家人數:"=w368, "普通電腦玩家人數:"=w367, "地圖:"=w366, "已加入的玩家:"=w369) -> (w365:T17)  [unwired: 1 in]
              n217 = Flatten To String(anything=w365) -> (data string=w373:string)  [unwired: 3 in, 2 out]
              n218 = UDP Write(address=w371, port or service name=u16 52023, connection ID=w372, data in=w373) -> ()  [unwired: 2 in, 2 out]
            }
          }
          frame 6 {
            n219 = call <vilib>:"Draw Rectangle.vi"("picture"=w445, "rect"=T11 {"left"=180, "top"=30, "right"=1100, "bottom"=690}, "fill?(F)"=TRUE, "color(black)"=u32 13816530) -> ("new picture"=w439:picture)  [unwired: 5 in]
            n220 = UDP Read(connection ID=w433, timeout ms (25000)=16) -> (data out=w429:string, error out=w430:errorcluster, 3:w432:refnum<k16>, 6:w428:u32)  [unwired: 2 in, 1 out]
            n221 = call <vilib>:"Draw Rectangle.vi"("picture"=w439, "rect"=T11 {"left"=180, "top"=30, "right"=1100, "bottom"=690}, "color(black)"=u32 0) -> ("new picture"=w435:picture)  [unwired: 6 in]
            n222 = case shown="No Error" w430 {
              tunnel: w429 -> [w470 _]
              tunnel: w428 -> [_ _]
              tunnel: w432 -> [w461 _]
              tunnel: [w464 _] -> w427
              frame No Error {
                w467 = 0
                n223 = Bundle(w467, w467, "", "已加入的玩家:"=string[] []) -> (w466:cluster{i32, i32, string, "已加入的玩家:":string[]})  [unwired: 1 in]
                n224 = Unflatten From String(type=w466, binary string=w470) -> (value=w465:cluster{i32, i32, string, "已加入的玩家:":string[]}, error out=w460:errorcluster)  [unwired: 3 in, 1 out]
                n225 = Unbundle(w460) -> ()  [unwired: 3 out]
                n226 = Unbundle(w465) -> (w458:i32, w459:i32, w457:string, "已加入的玩家:"=w456:string[])
                n227 = Equal?(x=w458, y=-1) -> (x = y?=w463:bool)
                n228 = case shown="True" w463 {
                  tunnel: [_ TRUE ("Visible")] -> w464
                  tunnel: w461 -> [_ w475]
                  tunnel: w459 -> [w474 _]
                  tunnel: w458 -> [w473 _]
                  tunnel: w457 -> [w472 _]
                  tunnel: w456 -> [w471 _]
                  frame False {
                    n229 = local write "已加入的玩家:"(w471) -> ()
                    n230 = local write "地圖:"(w472) -> ()
                    n231 = local write "初級電腦玩家人數:"(w473) -> ()
                    n232 = local write "普通電腦玩家人數:"(w474) -> ()
                  }
                  frame True {
                    n233 = property on="普通電腦玩家人數:" class="DigNum (strict)"("Visible"=FALSE) -> ()  [unwired: 2 in, 2 out]
                    n234 = property on="已加入的玩家:" class="Arr (strict)"("Visible"=FALSE) -> ()  [unwired: 2 in, 2 out]
                    n235 = property on="地圖:" class="CmbBox"("Visible"=FALSE) -> ()  [unwired: 2 in, 2 out]
                    n236 = UDP Close(connection ID=w475) -> ()  [unwired: 1 in, 2 out]
                    n237 = local write "Network Game"(TRUE ("Network Game")) -> ()
                    n238 = local write "Network Game"(TRUE ("Network Game")) -> ()
                    n239 = property on="初級電腦玩家人數:" class="DigNum (strict)"("Visible"=FALSE) -> ()  [unwired: 2 in, 2 out]
                  }
                }
              }
              frame Error {
              }
            }
            n240 = call <vilib>:"Draw Rectangle.vi"("picture"=w435, "rect"=T11 {"left"=180, "top"=30, "right"=1100, "bottom"=120}, "color(black)"=u32 0) -> ("new picture"=w436:picture)  [unwired: 6 in]
            n241 = call <vilib>:"Draw Text at Point.vi"("text orientation"=T16."None", "[user-specified font]"=T14 {"Font Name:"="Arial", "Size"=48, "Strikeout?"=FALSE, "Italic?"=FALSE, "Underline?"=FALSE, "Outline?"=FALSE, "Shadow?"=FALSE, "Bold?"=FALSE}, "text color(black)"=u32 0, "desired font(Application)"=T13."User-specified Font", "text"="等待遊戲開始...", "alignment(left, top)"=T15 {"horizontal"=enum."center", "vertical"=enum."top"}, "origin"=cluster{"x":i16, "y":i16} {"x"=640, "y"=50}, "picture"=w436) -> ("new picture"=w434:picture)  [unwired: 2 in, 1 out]
            n242 = call <vilib>:"Draw Text at Point.vi"("text"="All rights reserved by 113550153, 113550099", "origin"=cluster{"x":i16, "y":i16} {"x"=1015, "y"=695}, "picture"=w434) -> ("new picture"=w446:picture)  [unwired: 7 in, 1 out]
          }
          frame 4 {
            n243 = call <vilib>:"Draw Rectangle.vi"("picture"=w496, "rect"=T11 {"left"=180, "top"=30, "right"=1100, "bottom"=690}, "fill?(F)"=TRUE, "color(black)"=u32 13816530) -> ("new picture"=w490:picture)  [unwired: 5 in]
            n244 = call <vilib>:"Draw Rectangle.vi"("picture"=w490, "rect"=T11 {"left"=180, "top"=30, "right"=1100, "bottom"=690}, "color(black)"=u32 0) -> ("new picture"=w485:picture)  [unwired: 6 in]
            n245 = call <vilib>:"Draw Rectangle.vi"("picture"=w485, "rect"=T11 {"left"=180, "top"=30, "right"=640, "bottom"=690}, "color(black)"=u32 0) -> ("new picture"=w486:picture)  [unwired: 6 in]
            n246 = event shown="[1] \"進入遊戲\": Value Change" {
              selector: _ -> [_ _]
              dyn-events: _ -> [_ _]
              timeout: 1 -> [_ _]
              tunnel: [_ TRUE ("Visible")] -> w483
              event Timeout {
                n247 = event-data() -> ()  [unwired: 1 in, 3 out]
                n248 = local read "普通電腦玩家人數:"() -> (w516:i32)
                n249 = Subtract(x=19, y=w516) -> (x-y=w517:i32)
                n250 = property on="初級電腦玩家人數:" class="DigNum (strict)"("Maximum"=w517) -> ()  [unwired: 2 in, 2 out]
              }
              event "進入遊戲": Value Change {
                n251 = event-data() -> ()  [unwired: 1 in, 1 out]
                n252 = property on="Close (Main UI)" class="Bool (strict)"("Visible"=FALSE) -> ()  [unwired: 2 in, 2 out]
                n253 = property on="進入遊戲" class="Bool"("Visible"=FALSE) -> ()  [unwired: 2 in, 2 out]
                n254 = property on="玩家ID: (加入遊戲)" class="Str"("Visible"=FALSE) -> ()  [unwired: 2 in, 2 out]
                n255 = property on="地圖:" class="CmbBox"("Visible"=FALSE) -> ()  [unwired: 2 in, 2 out]
                n256 = property on="初級電腦玩家人數:" class="DigNum (strict)"("Visible"=FALSE) -> ()  [unwired: 2 in, 2 out]
                n257 = property on="普通電腦玩家人數:" class="DigNum (strict)"("Visible"=FALSE) -> ()  [unwired: 2 in, 2 out]
                n258 = property on="電腦代打模式:\n(Based on Machine Learning)\n(Behavior cloning)\n(Warning: High computing workload)" class="Bool (strict)"("Visible"=FALSE) -> ()  [unwired: 2 in, 2 out]
                n259 = local write "Network Game"(FALSE ("Network Game")) -> ()
                n260 = local read "玩家ID: (加入遊戲)"() -> (w519:string)
                n261 = Equal?(x=w519, y="") -> (x = y?=w521:bool)
                n262 = case shown="True" w521 {
                  tunnel: w519 -> [w531 _]
                  tunnel: [w531 w532] -> w520
                  frame False {
                  }
                  frame True {
                    n263 = Random Number (0-1)() -> (number: 0 to 1=w538:dbl)
                    n264 = Multiply(x=w538, y=9999.0) -> (x*y=w535:dbl)
                    n265 = To Long Integer(number=w535) -> (32bit integer=w533:i32)
                    n266 = Number To Decimal String(number=w533) -> (decimal integer string=w534:string)  [unwired: 1 in]
                    n267 = Concatenate Strings("無名氏_", w534) -> (w532:string)
                  }
                }
                n268 = local write "玩家ID: (加入遊戲)"(w520) -> ()
              }
            }
            n269 = call <vilib>:"Draw Text at Point.vi"("text orientation"=T16."None", "[user-specified font]"=T14 {"Font Name:"="Arial", "Size"=48, "Strikeout?"=FALSE, "Italic?"=FALSE, "Underline?"=FALSE, "Outline?"=FALSE, "Shadow?"=FALSE, "Bold?"=FALSE}, "text color(black)"=u32 0, "desired font(Application)"=T13."User-specified Font", "text"="遊戲玩家", "alignment(left, top)"=T15 {"horizontal"=enum."center", "vertical"=enum."top"}, "origin"=cluster{"x":i16, "y":i16} {"x"=400, "y"=150}, "picture"=w486) -> ("new picture"=w501:picture)  [unwired: 2 in, 1 out]
            n270 = call <vilib>:"Draw Text at Point.vi"("text orientation"=T16."None", "[user-specified font]"=T14 {"Font Name:"="Arial", "Size"=48, "Strikeout?"=FALSE, "Italic?"=FALSE, "Underline?"=FALSE, "Outline?"=FALSE, "Shadow?"=FALSE, "Bold?"=FALSE}, "text color(black)"=u32 0, "desired font(Application)"=T13."User-specified Font", "text"="地圖選項", "alignment(left, top)"=T15 {"horizontal"=enum."center", "vertical"=enum."top"}, "origin"=cluster{"x":i16, "y":i16} {"x"=880, "y"=150}, "picture"=w501) -> ("new picture"=w500:picture)  [unwired: 2 in, 1 out]
            n271 = call <vilib>:"Draw Text at Point.vi"("text"="All rights reserved by 113550153, 113550099", "origin"=cluster{"x":i16, "y":i16} {"x"=1015, "y"=695}, "picture"=w500) -> ("new picture"=w497:picture)  [unwired: 7 in, 1 out]
          }
          frame 1 {
            n272 = call <vilib>:"Draw Rectangle.vi"("picture"=w549, "rect"=T11 {"left"=180, "top"=30, "right"=1100, "bottom"=690}, "fill?(F)"=TRUE, "color(black)"=u32 13816530) -> ("new picture"=w543:picture)  [unwired: 5 in]
            n273 = call <vilib>:"Draw Rectangle.vi"("picture"=w543, "rect"=T11 {"left"=180, "top"=30, "right"=1100, "bottom"=690}, "color(black)"=u32 0) -> ("new picture"=w542:picture)  [unwired: 6 in]
            n274 = event shown="[1] \"進入遊戲\": Value Change" {
              selector: _ -> [_ _]
              dyn-events: _ -> [_ _]
              timeout: 1 -> [_ _]
              tunnel: [_ TRUE] -> w540
              event Timeout {
                n275 = event-data() -> ()  [unwired: 1 in, 3 out]
              }
              event "進入遊戲": Value Change {
                n276 = event-data() -> ()  [unwired: 1 in, 3 out]
                n277 = local write "電腦代打模式:\n(Based on Machine Learning)\n(Behavior cloning)\n(Warning: High computing workload)"(FALSE) -> ()
                n278 = Random Number (0-1)() -> (number: 0 to 1=w584:dbl)
                n279 = Multiply(x=w584, y=3.0) -> (x*y=w577:dbl)
                n280 = Greater Or Equal?(x=w577, y=1.0) -> (x >= y?=w576:bool)
                n281 = Greater Or Equal?(x=w577, y=2.0) -> (x >= y?=w581:bool)
                n282 = Select(t="Map 2" ("地圖:"), s=w576, f="Map 1" ("地圖:")) -> (s? t:f=w575:string)
                n283 = Select(t="Map 3" ("地圖:"), s=w581, f=w575) -> (s? t:f=w579:string)
                n284 = Random Number (0-1)() -> (number: 0 to 1=w588:dbl)
                n285 = Multiply(x=w588, y=9.0) -> (x*y=w568:dbl)
                n286 = Add(x=w568, y=10.0) -> (x+y=w569:dbl)
                n287 = property on="玩家ID: (加入遊戲)" class="Str"("Visible"=FALSE) -> ()  [unwired: 2 in, 2 out]
                n288 = property on="進入遊戲" class="Bool"("Visible"=FALSE) -> ()  [unwired: 2 in, 2 out]
                n289 = To Long Integer(number=w569) -> (32bit integer=w585:i32)
                n290 = local write "普通電腦玩家人數:"(w585) -> ()
                n291 = local write "初級電腦玩家人數:"(0 ("強力電腦玩家人數:")) -> ()
                n292 = local write "地圖:"(w579) -> ()
                n293 = property on="Close (Main UI)" class="Bool (strict)"("Visible"=FALSE) -> ()  [unwired: 2 in, 2 out]
                n294 = local write "Network Game"(FALSE ("Network Game")) -> ()
                n295 = local read "玩家ID: (加入遊戲)"() -> (w560:string)
                n296 = Equal?(x=w560, y="") -> (x = y?=w563:bool)
                n297 = case shown="True" w563 {
                  tunnel: w560 -> [w589 _]
                  tunnel: [w589 w590] -> w561
                  frame False {
                  }
                  frame True {
                    n298 = Random Number (0-1)() -> (number: 0 to 1=w596:dbl)
                    n299 = Multiply(x=w596, y=9999.0) -> (x*y=w593:dbl)
                    n300 = To Long Integer(number=w593) -> (32bit integer=w591:i32)
                    n301 = Number To Decimal String(number=w591) -> (decimal integer string=w592:string)  [unwired: 1 in]
                    n302 = Concatenate Strings("無名氏_", w592) -> (w590:string)
                  }
                }
                n303 = local write "玩家ID: (加入遊戲)"(w561) -> ()
              }
            }
            n304 = call <vilib>:"Draw Text at Point.vi"("text orientation"=T16."None", "[user-specified font]"=T14 {"Font Name:"="Arial", "Size"=48, "Strikeout?"=FALSE, "Italic?"=FALSE, "Underline?"=FALSE, "Outline?"=FALSE, "Shadow?"=FALSE, "Bold?"=FALSE}, "text color(black)"=u32 0, "desired font(Application)"=T13."User-specified Font", "text"="準備開始遊戲", "alignment(left, top)"=T15 {"horizontal"=enum."center", "vertical"=enum."top"}, "origin"=cluster{"x":i16, "y":i16} {"x"=640, "y"=150}, "picture"=w542) -> ("new picture"=w541:picture)  [unwired: 2 in, 1 out]
            n305 = call <vilib>:"Draw Text at Point.vi"("text"="All rights reserved by 113550153, 113550099", "origin"=cluster{"x":i16, "y":i16} {"x"=1015, "y"=695}, "picture"=w541) -> ("new picture"=w550:picture)  [unwired: 7 in, 1 out]
          }
        }
        n306 = Subtract(x=w82, y=w83) -> (x-y=w87:dbl)
        n307 = Divide(x=1.0, y=w87) -> (x/y=→"FPS":dbl)
        n308 = local read "STOP (會卡住)"() -> (w71:bool)
        n309 = Or(x=w73, y=w71) -> (x .or. y?=w74:bool)
        n310 = event shown="[4] \"Customized Game Button\": Value Change" {
          selector: _ -> [_ _ _ _ _ _]
          dyn-events: _ -> [_ _ _ _ _ _]
          timeout: 16 -> [_ _ _ _ _ _]
          event Timeout {
            n311 = event-data() -> ()  [unwired: 1 in, 3 out]
          }
          event "Game Start Button": Value Change {
            n312 = event-data() -> ()  [unwired: 1 in, 6 out]
            n313 = property on="Game Instruction Button" class="Bool"("Visible"=FALSE) -> ()  [unwired: 2 in, 2 out]
            n314 = property on="Game Start Button" class="Bool"("Visible"=FALSE) -> ()  [unwired: 2 in, 2 out]
            n315 = property on="Customized Game Button" class="Bool"("Visible"=FALSE) -> ()  [unwired: 2 in, 2 out]
            n316 = property on="Join/Create Room Button" class="Bool"("Visible"=FALSE) -> ()  [unwired: 2 in, 2 out]
            n317 = property on="Close (Main UI)" class="Bool (strict)"("Visible"=TRUE) -> ()  [unwired: 2 in, 2 out]
            n318 = property on="玩家ID: (加入遊戲)" class="Str"("Visible"=TRUE) -> ()  [unwired: 2 in, 2 out]
            n319 = property on="進入遊戲" class="Bool"("Visible"=TRUE) -> ()  [unwired: 2 in, 2 out]
            n320 = local write "State"(1 ("State")) -> ()
            n321 = property on="玩家ID: (加入遊戲)" class="Str"("Position"=T12 {"Left"=-162, "Top"=0}) -> ()  [unwired: 2 in, 2 out]
            n322 = property on="進入遊戲" class="Bool"("Left"=-100 ("Position:Left"), "Top"=120 ("Position:Top")) -> ()  [unwired: 2 in, 2 out]
          }
          event "Game Instruction Button": Value Change {
            n323 = event-data() -> ()  [unwired: 1 in, 6 out]
            n324 = property on="Game Instruction Button" class="Bool"("Visible"=FALSE) -> ()  [unwired: 2 in, 2 out]
            n325 = property on="Game Start Button" class="Bool"("Visible"=FALSE) -> ()  [unwired: 2 in, 2 out]
            n326 = property on="Customized Game Button" class="Bool"("Visible"=FALSE) -> ()  [unwired: 2 in, 2 out]
            n327 = property on="Join/Create Room Button" class="Bool"("Visible"=FALSE) -> ()  [unwired: 2 in, 2 out]
            n328 = local write "State"(2 ("State")) -> ()
            n329 = property on="Close (Main UI)" class="Bool (strict)"("Visible"=TRUE) -> ()  [unwired: 2 in, 2 out]
          }
          event "Join/Create Room Button": Value Change {
            n330 = event-data() -> ()  [unwired: 1 in, 6 out]
            n331 = property on="Game Instruction Button" class="Bool"("Visible"=FALSE) -> ()  [unwired: 2 in, 2 out]
            n332 = property on="Game Start Button" class="Bool"("Visible"=FALSE) -> ()  [unwired: 2 in, 2 out]
            n333 = property on="Customized Game Button" class="Bool"("Visible"=FALSE) -> ()  [unwired: 2 in, 2 out]
            n334 = property on="Join/Create Room Button" class="Bool"("Visible"=FALSE) -> ()  [unwired: 2 in, 2 out]
            n335 = property on="玩家ID: (加入遊戲)" class="Str"("Position"=T12 {"Left"=-384, "Top"=-136}) -> ()  [unwired: 2 in, 2 out]
            n336 = property on="Close (Main UI)" class="Bool (strict)"("Visible"=TRUE) -> ()  [unwired: 2 in, 2 out]
            n337 = property on="玩家ID: (創建遊戲)" class="Str"("Visible"=TRUE) -> ()  [unwired: 2 in, 2 out]
            n338 = property on="玩家ID: (加入遊戲)" class="Str"("Visible"=TRUE) -> ()  [unwired: 2 in, 2 out]
            n339 = property on="Host IP: (Local Network)" class="Str"("Visible"=TRUE) -> ()  [unwired: 2 in, 2 out]
            n340 = local write "State"(3 ("State")) -> ()
            n341 = property on="選擇網路介面:" class="CmbBox"("Visible"=TRUE) -> ()  [unwired: 2 in, 2 out]
            n342 = property on="加入遊戲" class="Bool"("Visible"=TRUE) -> ()  [unwired: 2 in, 2 out]
            n343 = property on="創建遊戲" class="Bool"("Visible"=TRUE) -> ()  [unwired: 2 in, 2 out]
          }
          event "Customized Game Button": Value Change {
            n344 = event-data() -> ()  [unwired: 1 in, 1 out]
            n345 = property on="初級電腦玩家人數:" class="DigNum (strict)"("Position"=T12 {"Left"=-400, "Top"=-90}) -> ()  [unwired: 2 in, 2 out]
            n346 = property on="普通電腦玩家人數:" class="DigNum (strict)"("Position"=T12 {"Left"=-400, "Top"=20}) -> ()  [unwired: 2 in, 2 out]
            n347 = property on="地圖:" class="CmbBox"("Position"=T12 {"Left"=90, "Top"=-72}) -> ()  [unwired: 2 in, 2 out]
            n348 = property on="玩家ID: (加入遊戲)" class="Str"("Position"=T12 {"Left"=72, "Top"=32}) -> ()  [unwired: 2 in, 2 out]
            n349 = property on="Game Instruction Button" class="Bool"("Visible"=FALSE) -> ()  [unwired: 2 in, 2 out]
            n350 = property on="Game Start Button" class="Bool"("Visible"=FALSE) -> ()  [unwired: 2 in, 2 out]
            n351 = property on="Customized Game Button" class="Bool"("Visible"=FALSE) -> ()  [unwired: 2 in, 2 out]
            n352 = property on="Join/Create Room Button" class="Bool"("Visible"=FALSE) -> ()  [unwired: 2 in, 2 out]
            n353 = property on="電腦代打模式:\n(Based on Machine Learning)\n(Behavior cloning)\n(Warning: High computing workload)" class="Bool (strict)"("Visible"=TRUE) -> ()  [unwired: 2 in, 2 out]
            n354 = local write "State"(4 ("State")) -> ()
            n355 = property on="Close (Main UI)" class="Bool (strict)"("Visible"=TRUE) -> ()  [unwired: 2 in, 2 out]
            n356 = property on="普通電腦玩家人數:" class="DigNum (strict)"("Visible"=TRUE) -> ()  [unwired: 2 in, 2 out]
            n357 = property on="初級電腦玩家人數:" class="DigNum (strict)"("Visible"=TRUE) -> ()  [unwired: 2 in, 2 out]
            n358 = property on="地圖:" class="CmbBox"("Visible"=TRUE) -> ()  [unwired: 2 in, 2 out]
            n359 = property on="玩家ID: (加入遊戲)" class="Str"("Visible"=TRUE) -> ()  [unwired: 2 in, 2 out]
            n360 = property on="進入遊戲" class="Bool"("Visible"=TRUE) -> ()  [unwired: 2 in, 2 out]
            n361 = property on="進入遊戲" class="Bool"("Left"=136 ("Position:Left"), "Top"=180 ("Position:Top")) -> ()  [unwired: 2 in, 2 out]
          }
          event "Close (Main UI)": Value Change {
            n362 = event-data() -> ()  [unwired: 1 in, 6 out]
            n363 = property on="普通電腦玩家人數:" class="DigNum (strict)"("Visible"=FALSE) -> ()  [unwired: 2 in, 2 out]
            n364 = property on="Game Instruction Button" class="Bool"("Visible"=TRUE) -> ()  [unwired: 2 in, 2 out]
            n365 = property on="初級電腦玩家人數:" class="DigNum (strict)"("Visible"=FALSE) -> ()  [unwired: 2 in, 2 out]
            n366 = property on="Game Start Button" class="Bool"("Visible"=TRUE) -> ()  [unwired: 2 in, 2 out]
            n367 = property on="Customized Game Button" class="Bool"("Visible"=TRUE) -> ()  [unwired: 2 in, 2 out]
            n368 = property on="Join/Create Room Button" class="Bool"("Visible"=TRUE) -> ()  [unwired: 2 in, 2 out]
            n369 = property on="電腦代打模式:\n(Based on Machine Learning)\n(Behavior cloning)\n(Warning: High computing workload)" class="Bool (strict)"("Visible"=FALSE) -> ()  [unwired: 2 in, 2 out]
            n370 = property on="創建遊戲" class="Bool"("Visible"=FALSE) -> ()  [unwired: 2 in, 2 out]
            n371 = property on="選擇網路介面:" class="CmbBox"("Visible"=FALSE) -> ()  [unwired: 2 in, 2 out]
            n372 = property on="進入遊戲" class="Bool"("Visible"=FALSE) -> ()  [unwired: 2 in, 2 out]
            n373 = local write "State"(0 ("State")) -> ()
            n374 = property on="Close (Main UI)" class="Bool (strict)"("Visible"=FALSE) -> ()  [unwired: 2 in, 2 out]
            n375 = property on="玩家ID: (加入遊戲)" class="Str"("Visible"=FALSE) -> ()  [unwired: 2 in, 2 out]
            n376 = property on="Host IP: (Local Network)" class="Str"("Visible"=FALSE) -> ()  [unwired: 2 in, 2 out]
            n377 = property on="玩家ID: (創建遊戲)" class="Str"("Visible"=FALSE) -> ()  [unwired: 2 in, 2 out]
            n378 = property on="加入遊戲" class="Bool"("Visible"=FALSE) -> ()  [unwired: 2 in, 2 out]
            n379 = property on="地圖:" class="CmbBox"("Visible"=FALSE) -> ()  [unwired: 2 in, 2 out]
          }
        }
        n380 = local write "PlayingScene"(w72) -> ()
      }
    }
    frame #2 {
      w604 = 0.0
      # "Data initialization"
      # "Initialize Entity Position Array"
      # "Game start general initialization"
      # "Player 0 is MP"
      n381 = local read "初級電腦玩家人數:"() -> (w612:i32)
      n382 = local read "普通電腦玩家人數:"() -> (w611:i32)
      n383 = local read "初級電腦玩家人數:"() -> (w617:i32)
      n384 = local read "普通電腦玩家人數:"() -> (w616:i32)
      n385 = local read "已加入的玩家:"() -> (w610:string[])
      n386 = local read "My NetPlayer number"() -> (w618:i32)
      n387 = local write "Background music"(0.0 ("Background music")) -> ()
      n388 = Bundle(w604, w604, w604, w604, w604, w604) -> (w605:cluster{dbl, dbl, dbl, dbl, dbl, dbl})  [unwired: 1 in]
      n389 = local write "Final Winner"("") -> ()
      n390 = Array Size(array=w610) -> (size(s)=w609:i32)
      n391 = property on="MP HP" class="Slide (strict)"("Visible"=TRUE) -> ()  [unwired: 2 in, 2 out]
      n392 = Compound Arithmetic op=ADD(w618, w617, w616) -> (w619:i32)
      n393 = local write "My NetPlayer number"(w619) -> ()
      n394 = Compound Arithmetic op=ADD(w609, w612, w611) -> (w599:i32)
      n395 = Increment(x=w599) -> (x+1=→"Alive number":i32)
      n396 = Initialize Array(0, w599) -> (→"Player HP Healing (And visibility)":i32[])
      n397 = Initialize Array(30, w599) -> (→"Player Bullets":i32[])
      n398 = Initialize Array(0, w599) -> (→"Player Bullets Reload":i32[])
      n399 = Initialize Array(w605, w599) -> (→"Moving Entity Position":cluster{dbl, dbl, dbl, dbl, dbl, dbl}[])
      n400 = Decrement(x=w599) -> (x-1=w598:i32)
      n401 = local read "Network Game"() -> (w620:bool)
      n402 = local write "MO ID"(w598) -> ()
    }
  }
  n403 = call <vilib>:"RGB to Color.vi"("B"=u8 160, "G"=u8 215, "R"=u8 255) -> ("Color"=→"Color":u32)
  n404 = call <vilib>:"RGB to Color.vi"("B"=u8 85, "G"=u8 140, "R"=u8 180) -> ("Color"=→"Color 2":u32)
  n405 = while {
    tunnel: w2 -> [_]
    stop <- "STOP (會卡住)" stop-if-true
    n406 = Wait (ms)(milliseconds to wait=u32 16) -> ()  [unwired: 1 out]
  }
  n407 = while {
    tunnel: w2 -> [_]
    stop <- w624 stop-if-true
    # "Music playing loop"
    n408 = local read "Background music"() -> (w625:dbl)
    n409 = Wait (ms)(milliseconds to wait=u32 16) -> ()  [unwired: 1 out]
    n410 = case shown="1" w625 {
      tunnel: [w626 w632 w663] -> w624
      frame 0, Default {
        n411 = local read "STOP (會卡住)"() -> (w626:bool)
      }
      frame 1 {
        n412 = Current VI's Path() -> (path=w634:path)
        n413 = Strip Path(path=w634) -> (stripped path=w631:path)  [unwired: 1 out]
        n414 = Build Path(base path=w631, name or relative path="Musics\\Surviv.io Saloon Music on Piano.wav") -> (appended path=w628:path)
        n415 = call <vilib>:"Play Sound File.vi"("path"=w628, "device ID"=u32 0) -> ("error out"=w629:errorcluster, "task ID"=w630:T18)  [unwired: 8 in]
        n416 = while {
          tunnel: [w636] -> w632
          tunnel: w630 -> [w645]
          tunnel: w629 -> [w646]
          stop <- w637 stop-if-true
          n417 = local read "Background music"() -> (w644:dbl)
          n418 = local read "STOP (會卡住)"() -> (w636:bool)
          n419 = Equal?(x=1.0, y=w644) -> (x = y?=w640:bool)
          n420 = Not(x=w636) -> (.not. x?=w641:bool)
          n421 = And(x=w640, y=w641) -> (x .and. y?=w639:bool)
          n422 = case shown="False" w639 {
            tunnel: w646 -> [w650 w654]
            tunnel: w645 -> [w651 w653]
            tunnel: [FALSE ("is playing?") w652] -> w642
            frame False {
              n423 = call <vilib>:"Sound Output Stop.vi"("error in (no error)"=w650, "task ID"=w651) -> ("error out"=w648:errorcluster, "task ID out"=w649:T18)  [unwired: 8 in]
              n424 = call <vilib>:"Sound Output Clear.vi"("error in (no error)"=w648, "task ID"=w649) -> ()  [unwired: 9 in, 1 out]
            }
            frame True {
              n425 = call <vilib>:"Sound Output Info.vi"("error in (no error)"=w654, "task ID"=w653) -> ("is playing?"=w652:bool)  [unwired: 6 in, 3 out]
            }
          }
          n426 = Not(x=w642) -> (.not. x?=w638:bool)
          n427 = Or(x=w638, y=w636) -> (x .or. y?=w637:bool)
          n428 = Wait (ms)(milliseconds to wait=u32 16) -> ()  [unwired: 1 out]
        }
      }
      frame 2 {
        n429 = Current VI's Path() -> (path=w665:path)
        n430 = Strip Path(path=w665) -> (stripped path=w662:path)  [unwired: 1 out]
        n431 = Build Path(base path=w662, name or relative path="Musics\\First_Built_Last_Found.wav") -> (appended path=w661:path)
        n432 = call <vilib>:"Play Sound File.vi"("path"=w661, "device ID"=u32 0) -> ("error out"=w658:errorcluster, "task ID"=w657:T18)  [unwired: 8 in]
        n433 = call-poly <vilib>:"Sound Output Set Volume.vi"("error in (no error)"=w658, "volume"=75.0, "task ID"=w657) -> ("error out"=w655:errorcluster, "task ID out"=w656:T18)  [unwired: 7 in]
        n434 = while {
          tunnel: [w667] -> w663
          tunnel: w656 -> [w676]
          tunnel: w655 -> [w677]
          stop <- w668 stop-if-true
          n435 = local read "Background music"() -> (w675:dbl)
          n436 = local read "STOP (會卡住)"() -> (w667:bool)
          n437 = Equal?(x=2.0, y=w675) -> (x = y?=w671:bool)
          n438 = Not(x=w667) -> (.not. x?=w672:bool)
          n439 = And(x=w671, y=w672) -> (x .and. y?=w670:bool)
          n440 = case shown="True" w670 {
            tunnel: w677 -> [w681 w685]
            tunnel: w676 -> [w682 w684]
            tunnel: [FALSE ("is playing?") w683] -> w673
            frame False {
              n441 = call <vilib>:"Sound Output Stop.vi"("error in (no error)"=w681, "task ID"=w682) -> ("error out"=w679:errorcluster, "task ID out"=w680:T18)  [unwired: 8 in]
              n442 = call <vilib>:"Sound Output Clear.vi"("error in (no error)"=w679, "task ID"=w680) -> ()  [unwired: 9 in, 1 out]
            }
            frame True {
              n443 = call <vilib>:"Sound Output Info.vi"("error in (no error)"=w685, "task ID"=w684) -> ("is playing?"=w683:bool)  [unwired: 6 in, 3 out]
            }
          }
          n444 = Not(x=w673) -> (.not. x?=w669:bool)
          n445 = Or(x=w669, y=w667) -> (x .or. y?=w668:bool)
          n446 = Wait (ms)(milliseconds to wait=u32 16) -> ()  [unwired: 1 out]
        }
      }
    }
  }
  n447 = case shown="True" w1 {
    frame False {
      # "If current user the the host of a game"
      n448 = flat-sequence {
        tunnel: [w726] -> w692
        tunnel: [w708] -> w691
        tunnel: [w730] -> w690
        tunnel: [w729] -> w689
        tunnel: [w728] -> w688
        tunnel: [w718] -> w687
        tunnel: [w717] -> w686
        tunnel: w692 -> [w873]
        tunnel: w691 -> [w878]
        tunnel: w690 -> [w882]
        tunnel: w689 -> [w854]
        tunnel: w688 -> [w872]
        tunnel: w687 -> [w865]
        tunnel: w686 -> [w864]
        frame #0 {
          w723 = 0.0
          # "Build Player info array"
          # "Shuffle initial player positions"
          # "Read map from csv file"
          n449 = local read "初級電腦玩家人數:"() -> (w703:i32)
          n450 = local read "普通電腦玩家人數:"() -> (w702:i32)
          n451 = local read "地圖:"() -> (w735:string)
          n452 = Current VI's Path() -> (path=w741:path)
          n453 = local read "電腦代打模式:\n(Based on Machine Learning)\n(Behavior cloning)\n(Warning: High computing workload)"() -> (w706:bool)
          n454 = local read "NetPlayer"() -> (w705:cluster{"Name":string, "IP Address":u32}[])
          n455 = Array Size(array=w705) -> (size(s)=w704:i32)
          n456 = Strip Path(path=w741) -> (stripped path=w742:path)  [unwired: 1 out]
          n457 = Concatenate Strings("Tables\\" ("string"), w735, ".csv" ("string")) -> (w732:string)
          n458 = Add(x=w703, y=w702) -> (x+y=w695:i32)
          n459 = Build Path(base path=w742, name or relative path=w732) -> (appended path=w740:path)
          n460 = Compound Arithmetic op=ADD(w703, w702, w704) -> (w726:i32)
          n461 = call-poly <vilib>:"Read Delimited Spreadsheet.vi"("file path (dialog if empty)"=w740, "number of rows (all:-1)"=-1, "start of read offset (chars.:0)"=1, "delimiter (\\t)"="," ("delimiter (\\t)")) -> ("all rows"=w746:dbl[][])  [unwired: 6 in, 5 out]
          n462 = Array Size(array=w746) -> (size(s)=w743:i32[])
          n463 = local read "NetPlayer Commend"() -> (w694:T1)
          n464 = Increment(x=w726) -> (x+1=w719:i32)
          n465 = for {
            N: w695 -> [_]
            shift-right: [w812] -> w728
            shift-left: refnum<queue>[] [] -> [w813]
            shift-right: [w807] -> w730
            shift-left: refnum<queue>[] [] -> [w806]
            tunnel: w719 -> [w804]
            tunnel: w702 -> [w805]
            i -> [w793]
            w814 = 0.0
            # "Build queue array\nMain.vi <- AI Player.vi"
            # "Build queue array\nMain.vi -> AI Player.vi"
            n466 = Increment(x=w793) -> (x+1=w794:i32)
            n467 = Number To Decimal String(number=w794) -> (decimal integer string=w809:string)  [unwired: 1 in]
            n468 = Less?(x=w793, y=w805) -> (x < y?=w803:bool)
            n469 = Number To Decimal String(number=w794) -> (decimal integer string=w811:string)  [unwired: 1 in]
            n470 = Concatenate Strings("ToAI_" ("string"), w809) -> (w802:string)
            n471 = Bundle(w814, w814, w814, w814) -> (w797:cluster{dbl, dbl, dbl, dbl})  [unwired: 1 in]
            n472 = Concatenate Strings("ToMain_" ("string"), w811) -> (w796:string)
            n473 = Obtain Queue(max queue size (-1, unlimited)=2, name (unnamed)=w802, element data type=T8 [] ("Map Entity Object Position")) -> (queue out=w800:refnum<queue>)  [unwired: 2 in, 2 out]
            n474 = Obtain Queue(max queue size (-1, unlimited)=2, name (unnamed)=w796, element data type=w797) -> (queue out=w798:refnum<queue>)  [unwired: 2 in, 2 out]
            n475 = case shown="False" w803 {
              tunnel: w804 -> [w818 w825]
              tunnel: w794 -> [w817 w824]
              tunnel: w798 -> [w816 w823]
              tunnel: w800 -> [w815 w822]
              frame True {
                # "Start Basic AI player"
                n476 = vi-ref "Basic AI Player.vi"() -> (w821:refnum<vi>)
                n477 = Open VI Reference(vi path=w821, options=256) -> (vi reference=w819:refnum<vi>)  [unwired: 4 in, 1 out]
                n478 = call-by-ref "Start Asynchronous Call"(reference=w819, "Total Player number"=w818, "Current Player ID number"=w817, "queue output"=w816, "queue input"=w815) -> ()  [unwired: 1 in, 2 out]
              }
              frame False {
                # "Start Weak AI player"
                n479 = vi-ref "Weak AI Player.vi"() -> (w828:refnum<vi>)
                n480 = Open VI Reference(vi path=w828, options=256) -> (vi reference=w826:refnum<vi>)  [unwired: 4 in, 1 out]
                n481 = call-by-ref "Start Asynchronous Call"(reference=w826, "Total Player number"=w825, "Current Player ID number"=w824, "queue output"=w823, "queue input"=w822) -> ()  [unwired: 1 in, 2 out]
              }
            }
            n482 = Build Array (concatenate)(w806, w800) -> (w807:refnum<queue>[])
            n483 = Build Array (concatenate)(w813, w798) -> (w812:refnum<queue>[])
          }
          n484 = Index Array(array=w743, index=0) -> (element=w744:i32)
          n485 = local read "NetPlayer"() -> (w696:cluster{"Name":string, "IP Address":u32}[])
          n486 = Bundle(w723, "玩家ID: (加入遊戲)"="玩家ID: (加入遊戲)", w723, -1.0, w723) -> (w727:T20)  [unwired: 1 in]
          n487 = Decrement(x=w744) -> (x-1=w745:i32)
          n488 = case shown="True" w706 {
            tunnel: w719 -> [_ w782]
            tunnel: [_ w780] -> w718
            tunnel: [_ w779] -> w717
            frame False {
            }
            frame True {
              w787 = 0.0
              # "Calling ML Player (based on Random Forest method)\n(It is on my presentation, but it is not in this version)\nSince it require python kits, we provide you a state-action\nbased ML AI Player."
              n489 = Bundle(w787, w787, w787, w787) -> (w786:cluster{dbl, dbl, dbl, dbl})  [unwired: 1 in]
              n490 = Obtain Queue(max queue size (-1, unlimited)=2, name (unnamed)="MP", element data type=T8 [] ("Map Entity Object Position")) -> (queue out=w780:refnum<queue>)  [unwired: 2 in, 2 out]
              n491 = Obtain Queue(max queue size (-1, unlimited)=2, name (unnamed)="MP receive", element data type=w786) -> (queue out=w779:refnum<queue>)  [unwired: 2 in, 2 out]
              n492 = vi-ref "ML AI Player.vi"() -> (w792:refnum<vi>)
              n493 = Open VI Reference(vi path=w792, options=256) -> (vi reference=w790:refnum<vi>)  [unwired: 4 in, 1 out]
              n494 = call-by-ref "Start Asynchronous Call"(reference=w790, "Total Player number"=w782, "Current Player ID number"=0, "queue output"=w779, "queue input"=w780) -> ()  [unwired: 1 in, 2 out]
            }
          }
          n495 = Array Size(array=w696) -> (size(s)=w697:i32)
          n496 = for {
            N: w745 -> [_]
            tunnel: w746 -> [w838]
            shift-right: [w831] -> w713
            shift-left: T8 [] ("Map Entity Object Position") -> [w832]
            i -> [w834]
            n497 = Increment(x=w834) -> (x+1=w833:i32)
            n498 = Array Subset(array=w838, index (row)=w833, length (row)=1 ("length"), index (col)=0 ("index"), length (col)=11 ("length")) -> (w840:dbl[][])
            n499 = Reshape Array(w840, 11 ("dimension size")) -> (w830:dbl[])
            n500 = Array To Cluster(array=w830) -> (cluster=w829:T21)
            n501 = Build Array (concatenate)(w832, w829) -> (w831:T22)
          }
          n502 = Greater Than 0?(x=w697) -> (x > 0?=w698:bool)
          n503 = Build Array (concatenate)(T6 [] ("Player info"), w727) -> (w725:T23)
          n504 = Greater Than 0?(x=w695) -> (x > 0?=w699:bool)
          n505 = case shown="False" w699 {
            tunnel: w725 -> [w765 w768]
            tunnel: w695 -> [_ w767]
            tunnel: [w765 w766] -> w701
            frame False {
            }
            frame True {
              n506 = for {
                N: w767 -> [_]
                shift-right: [w777] -> w766
                shift-left: w768 -> [w778]
                i -> [w776]
                w770 = 0.0
                n507 = Increment(x=w776) -> (x+1=w775:i32)
                n508 = Number To Decimal String(number=w775) -> (decimal integer string=w774:string)  [unwired: 1 in]
                n509 = Concatenate Strings("BotPlayer_" ("string"), w774) -> (w771:string)
                n510 = Bundle(w770, w771, w770, -1.0, w770) -> (w773:cluster{dbl, string, dbl, dbl, dbl})  [unwired: 1 in]
                n511 = Build Array (concatenate)(w778, w773) -> (w777:T23)
              }
            }
          }
          n512 = case shown="True" w698 {
            tunnel: w696 -> [_ w753]
            tunnel: w701 -> [w748 w752]
            tunnel: [w748 w751] -> w700
            tunnel: w694 -> [w747 w750]
            tunnel: [w747 w749] -> w693
            frame False {
            }
            frame True {
              n513 = for {
                tunnel: w753 -> [w762] mode=indexing
                shift-right: [w764] -> w751
                shift-left: w752 -> [w763]
                shift-right: [w757] -> w749
                shift-left: w750 -> [w756]
                w754 = sgl 0.0
                w761 = 0.0
                n514 = Unbundle(w762) -> ("Name"=w759:string)  [unwired: 1 out]
                n515 = Bundle(w761, "Name"=w759, w761, -1.0, w761) -> (w758:cluster{dbl, "Name":string, dbl, dbl, dbl})  [unwired: 1 in]
                n516 = Build Array (concatenate)(w763, w758) -> (w764:T6)
                n517 = Bundle(w754, w754, w754, w754, w754) -> (w755:cluster{sgl, sgl, sgl, sgl, sgl})  [unwired: 1 in]
                n518 = Build Array (concatenate)(w756, w755) -> (w757:T1)
              }
            }
          }
          "Player info" <- w700
          n519 = Array Subset(array=w713, index=0, length=20) -> (w714:T8)
          n520 = call "Shuffle 1D Array.vim"("array"=w714) -> ("shuffled array"=w709:T8)  [unwired: 4 in]
          n521 = Delete From Array(array=w713, length=20, index=0) -> (array with subset deleted=w710:T8)  [unwired: 1 out]
          n522 = Build Array (concatenate)(w709, w710) -> (w708:T8)
          "Map Entity Object Position" <- w708
          n523 = local write "NetPlayer Commend"(w693) -> ()
          n524 = Array Size(array=w708) -> (size(s)=w729:i32)
        }
        frame #1 {
          # "Network model"
          # "Shading Model"
          # "Physic Engine  (Position Processing Model)"
          # "Input Detection Model"
          # "Initial scene input"
          n525 = Obtain Queue(max queue size (-1, unlimited)=3, name (unnamed)="Shading Model", element data type=T8 [] ("Map Entity Object Position")) -> (queue out=w881:refnum<queue>)  [unwired: 2 in, 2 out]
          n526 = Lossy Enqueue Element(queue=w881, element=w878) -> (queue out=w880:refnum<queue>)  [unwired: 1 in, 3 out]
          n527 = Lossy Enqueue Element(queue=w880, element=w878) -> (queue out=w879:refnum<queue>)  [unwired: 1 in, 3 out]
          n528 = Lossy Enqueue Element(queue=w879, element=w878) -> ()  [unwired: 1 in, 4 out]
          n529 = Obtain Queue(max queue size (-1, unlimited)=3, name (unnamed)="Network Model", element data type=T8 [] ("Map Entity Object Position")) -> (queue out=w855:refnum<queue>)  [unwired: 2 in, 2 out]
          n530 = Obtain Queue(max queue size (-1, unlimited)=3, name (unnamed)=" Position Processing Model (Shoot)", element data type=T7 [] ("Moving Entity Position")) -> (queue out=w871:refnum<queue>)  [unwired: 2 in, 2 out]
          n531 = Obtain Queue(max queue size (-1, unlimited)=3, name (unnamed)=" Position Processing Model (Move)", element data type=T7 [] ("Moving Entity Position")) -> (queue out=w870:refnum<queue>)  [unwired: 2 in, 2 out]
          n532 = local read "地圖:"() -> (w843:string)
          n533 = while {
            shift-right: [w1357] -> _
            shift-left: w878 -> [w1364]
            tunnel: w870 -> [w1382]
            tunnel: w881 -> [w1381]
            tunnel: w871 -> [w1374]
            shift-right: [w1355] -> _
            shift-left: T7 [] ("Moving Entity Position") -> [w1372]
            tunnel: w873 -> [w1354]
            tunnel: w855 -> [w1352]
            stop <- w1384 stop-if-true
            # "Write processed data to PlayingScene and NetPlayer"
            # "Move command process"
            n534 = Dequeue Element(queue=w1382, timeout in ms (-1)=300) -> (element=w1365:T7)  [unwired: 1 in, 3 out]
            n535 = Dequeue Element(queue=w1374, timeout in ms (-1)=0) -> (element=w1363:T7, timed out?=w1360:bool)  [unwired: 1 in, 2 out]
            n536 = Not(x=w1360) -> (.not. x?=w1361:bool)
            n537 = case shown="True" w1361 {
              tunnel: [T7 [] ("Moving Entity Position") w1473] -> w1367
              tunnel: w1364 -> [_ w1471]
              tunnel: w1363 -> [_ w1470]
              frame False {
              }
              frame True {
                n538 = Array Size(array=w1470) -> (size(s)=w1472:i32)
                n539 = for {
                  N: w1472 -> [_]
                  shift-right: [w1503] -> w1473
                  shift-left: w1470 -> [w1502]
                  tunnel: w1471 -> [w1498]
                  shift-right: [w1478] -> _
                  shift-left: 0 ("timeout in ms (-1)") -> [w1479]
                  i -> [w1481]
                  # "Generate bullet based on bullet request.\nMeanwhile, check if it is a valid request."
                  # "Bullet info aggregation"
                  n540 = local read "Player HP Healing (And visibility)"() -> (w1476:i32[])
                  n541 = Add(x=w1481, y=w1479) -> (x+y=w1480:i32)
                  n542 = Index Array(array=w1502, index=w1480) -> (element=w1501:T24)
                  n543 = Unbundle(w1501) -> ("Object type"=w1497:dbl, "Move info"=w1500:dbl, "Vector scalar"=w1499:dbl, "Vector theta"=w1491:dbl)  [unwired: 2 out]
                  n544 = Subtract(x=w1497, y=100.0) -> (x-y=w1474:dbl)
                  n545 = Index Array(array=w1498, index=w1474) -> (element=w1495:T5)
                  n546 = Unbundle By Name(w1495) -> ("X"=w1490:dbl, "Y"=w1489:dbl, "HP"=w1484:dbl)
                  n547 = Greater?(x=w1484, y=0.0) -> (0:w1482:bool)
                  n548 = Replace Array Subset(array=w1476, new element=600 ("new element/subarray"), index=w1474) -> (w1477:i32[])
                  n549 = local write "Player HP Healing (And visibility)"(w1477) -> ()
                  n550 = call "rotation matrix.vi"("angle"=w1491, "y"=0.0 ("angle"), "x"=-40.0) -> ("new y"=w1487:dbl, "new x"=w1488:dbl)
                  n551 = Add(x=w1490, y=w1488) -> (x+y=w1494:dbl)
                  n552 = Add(x=w1489, y=w1487) -> (x+y=w1492:dbl)
                  n553 = Bundle(w1494, w1492, "Object type"=w1497, "Move info"=w1500, "Vector scalar"=w1499, "Vector theta"=w1491) -> (w1493:T25)  [unwired: 1 in]
                  n554 = case shown="True" w1482 {
                    tunnel: [w1506 w1514] -> w1503
                    tunnel: w1502 -> [w1507 w1513]
                    tunnel: w1480 -> [w1509 w1512]
                    tunnel: w1493 -> [_ w1511]
                    tunnel: w1479 -> [w1505 w1510]
                    tunnel: [w1504 w1510] -> w1478
                    frame False {
                      n555 = Decrement(x=w1505) -> (x-1=w1504:i32)
                      n556 = Delete From Array(array=w1507, length=1, index=w1509) -> (array with subset deleted=w1506:T7)  [unwired: 1 out]
                    }
                    frame True {
                      n557 = Replace Array Subset(array=w1513, new element=w1511, index=w1512) -> (w1514:T7)
                    }
                  }
                }
              }
            }
            n558 = Array Size(array=w1365) -> (size(s)=w1366:i32)
            n559 = for {
              N: w1366 -> [_]
              shift-right: [w1531] -> w1350
              shift-left: w1365 -> [w1530]
              tunnel: w1364 -> [w1526]
              i -> [w1529]
              # "-5000 means  no input"
              n560 = Index Array(array=w1530, index=w1529) -> (element=w1528:T24)
              n561 = Unbundle(w1528) -> ("Object type"=w1523:dbl, "Move info"=w1515:dbl, "Vector scalar"=w1524:dbl, "Vector theta"=w1525:dbl)  [unwired: 2 out]
              n562 = Index Array(array=w1526, index=w1523) -> (element=w1527:T5)
              n563 = Unbundle By Name(w1527) -> ("X"=w1522:dbl, "Y"=w1521:dbl, "Theta"=w1517:dbl)
              n564 = Equal?(x=w1515, y=-5000.0) -> (x = y?=w1519:bool)
              n565 = Select(t=w1517, s=w1519, f=w1515) -> (s? t:f=w1516:dbl)
              n566 = Bundle("X"=w1522, "Y"=w1521, "Object type"=w1523, "Move info"=w1516, "Vector scalar"=w1524, "Vector theta"=w1525) -> (w1520:T24)  [unwired: 1 in]
              n567 = Replace Array Subset(array=w1530, new element=w1520, index=w1529) -> (w1531:T7)
            }
            n568 = Build Array (concatenate)(w1372, w1367, w1350) -> (w1373:T7)
            n569 = Array Size(array=w1373) -> (size(s)=w1383:i32)
            n570 = for {
              N: w1383 -> [_]
              shift-right: [w1549] -> w1358
              shift-left: w1364 -> [w1550]
              tunnel: w1373 -> [w1551]
              shift-right: [w1548] -> w1355
              shift-left: T7 [] ("Moving Entity Position") -> [w1547]
              tunnel: w1354 -> [w1544]
              i -> [w1546]
              n571 = case shown="True" TRUE {
                tunnel: w1551 -> [_ w1565]
                tunnel: w1546 -> [_ w1564]
                tunnel: w1550 -> [w1553 w1561]
                tunnel: [w1553 w1559] -> w1549
                tunnel: [w1552 w1556] -> w1548
                tunnel: w1547 -> [w1552 w1555]
                tunnel: w1544 -> [_ w1554]
                frame False {
                }
                frame True {
                  # "Check moving object is\nplayer or bullet"
                  n572 = Index Array(array=w1565, index=w1564) -> (element=w1558:T24)
                  n573 = Unbundle By Name(w1558) -> ("Object type"=w1560:dbl, "Move info"=w1557:dbl)  [unwired: 4 out]
                  n574 = Less?(x=w1560, y=20.0) -> (x < y?=w1562:bool)
                  n575 = case shown="True" w1562 {
                    tunnel: w1561 -> [w1568 w1647]
                    tunnel: w1558 -> [w1567 w1648]
                    tunnel: w1560 -> [w1570 w1645]
                    tunnel: [w1573 w1646] -> w1559
                    tunnel: w1557 -> [_ w1643]
                    tunnel: [w1572 w1642] -> w1556
                    tunnel: w1555 -> [w1571 w1642]
                    tunnel: w1554 -> [w1566 w1641]
                    frame False {
                      # "100 represent bullet doesn't hit anything\n200 represent bullet hit objects but not player"
                      n576 = call "Collision Detection.vi"("Map Entity Objects Positions"=w1568, "Max Player ID number"=w1566, "Moving Object"=w1567) -> ("Bullet hit Player No."=w1569:i32)  [unwired: 1 out]
                      n577 = case shown="0, Default" w1569 {
                        tunnel: [w1597 w1636 w1640] -> w1573
                        tunnel: w1568 -> [w1596 w1636 w1640]
                        tunnel: [w1598 w1638 w1639] -> w1572
                        tunnel: w1571 -> [w1598 w1637 w1639]
                        tunnel: w1567 -> [_ w1635 _]
                        tunnel: w1569 -> [w1574 _ _]
                        tunnel: w1570 -> [w1579 _ _]
                        frame 0, Default {
                          # "Change the player visibility also"
                          # "Change HP points of the hit player"
                          n578 = local read "Player HP Healing (And visibility)"() -> (w1577:i32[])
                          n579 = Index Array(array=w1596, index=w1574) -> (element=w1595:T5)
                          n580 = Unbundle(w1595) -> ("X"=w1593:dbl, "Y"=w1592:dbl, "Object type"=w1591:dbl, "Radius"=w1590:dbl, "Width"=w1589:dbl, "Height"=w1588:dbl, "Theta"=w1587:dbl, "HP"=w1581:dbl, "R"=w1586:dbl, "G"=w1585:dbl, "B"=w1584:dbl)
                          n581 = Less Or Equal?(x=w1581, y=10.5) -> (x <= y?=w1578:bool)
                          n582 = case shown="True" w1578 {
                            tunnel: w1579 -> [_ w1620]
                            tunnel: w1574 -> [_ w1607]
                            frame False {
                            }
                            frame True {
                              n583 = Subtract(x=w1620, y=100.0) -> (x-y=w1601:dbl)
                              n584 = local read "Alive number"() -> (w1602:i32)
                              n585 = local read "Player info"() -> (w1618:T6)
                              n586 = Index Array(array=w1618, index=w1601) -> (element=w1617:T26)
                              n587 = Unbundle(w1617) -> ("Kills"=w1613:dbl, "Name"=w1615:string, "Rank"=w1611:dbl, "Who Kill Me"=w1610:dbl, "After Kill"=w1609:dbl)
                              n588 = Decrement(x=w1602) -> (x-1=w1612:i32)
                              n589 = Increment(x=w1613) -> (x+1=w1614:dbl)
                              n590 = local write "Alive number"(w1612) -> ()
                              n591 = Bundle(w1614, "Name"=w1615, "Rank"=w1611, "Who Kill Me"=w1610, "After Kill"=w1609) -> (w1616:T27)  [unwired: 1 in]
                              n592 = Replace Array Subset(array=w1618, new element=w1616, index=w1601) -> (w1608:T6)
                              n593 = Index Array(array=w1608, index=w1607) -> (element=w1606:T26)
                              n594 = Unbundle(w1606) -> ("Kills"=w1600:dbl, "Name"=w1599:string)  [unwired: 3 out]
                              n595 = Bundle("Kills"=w1600, "Name"=w1599, "Alive number"=w1602, w1601, "y"=600.0) -> (w1605:T28)  [unwired: 1 in]
                              n596 = Replace Array Subset(array=w1608, new element=w1605, index=w1607) -> (w1604:T6)
                              n597 = local write "Player info"(w1604) -> ()
                            }
                          }
                          n598 = Replace Array Subset(array=w1577, new element=600 ("new element/subarray"), index=w1574) -> (w1576:i32[])
                          n599 = local write "Player HP Healing (And visibility)"(w1576) -> ()
                          n600 = Subtract(x=w1581, y=10.5) -> (x-y=w1582:dbl)
                          n601 = Bundle("X"=w1593, "Y"=w1592, "Object type"=w1591, "Radius"=w1590, "Width"=w1589, "Height"=w1588, "Theta"=w1587, w1582, "R"=w1586, "G"=w1585, "B"=w1584) -> (w1594:T29)  [unwired: 1 in]
                          n602 = Replace Array Subset(array=w1596, new element=w1594, index=w1574) -> (w1597:T8)
                        }
                        frame 100 {
                          n603 = Unbundle(w1635) -> ("X"=w1624:dbl, "Y"=w1627:dbl, "Object type"=w1634:dbl, "Move info"=w1633:dbl, "Vector scalar"=w1630:dbl, "Vector theta"=w1632:dbl)
                          n604 = Sine & Cosine(0:w1632) -> (1:w1629:dbl, 2:w1628:dbl)
                          n605 = Multiply(x=w1630, y=w1629) -> (x*y=w1626:dbl)
                          n606 = Multiply(x=w1630, y=w1628) -> (x*y=w1621:dbl)
                          n607 = Add(x=w1627, y=w1626) -> (x+y=w1625:dbl)
                          n608 = Negate(x=w1621) -> (-x=w1622:dbl)
                          n609 = Add(x=w1624, y=w1622) -> (x+y=w1623:dbl)
                          n610 = Bundle(w1623, w1625, "Object type"=w1634, "Move info"=w1633, "Vector scalar"=w1630, "Vector theta"=w1632) -> (w1631:T25)  [unwired: 1 in]
                          n611 = Build Array (concatenate)(w1637, w1631) -> (w1638:T7)
                        }
                        frame 200 {
                        }
                      }
                    }
                    frame True {
                      # "If it is player, then let bullet fly."
                      # "Check if player alive"
                      n612 = Index Array(array=w1647, index=w1645) -> (element=w1644:T5)
                      n613 = Unbundle By Name(w1644) -> ("HP"=w1649:dbl)
                      n614 = Greater?(x=w1649, y=0.0) -> (0:w1650:bool)
                      n615 = case shown="True" w1650 {
                        tunnel: w1648 -> [_ w1655]
                        tunnel: w1647 -> [w1652 w1654]
                        tunnel: [w1652 w1680] -> w1646
                        tunnel: w1645 -> [_ w1679]
                        tunnel: w1644 -> [_ w1678]
                        tunnel: w1643 -> [_ w1659]
                        tunnel: w1641 -> [_ w1653]
                        frame False {
                        }
                        frame True {
                          # "Move based on the info from Collision Detection.vi"
                          n616 = Unbundle By Name(w1678) -> ("X"=w1673:dbl, "Y"=w1661:dbl, "Object type"=w1670:dbl, "Radius"=w1669:dbl, "Width"=w1668:dbl, "Height"=w1667:dbl, "HP"=w1666:dbl, "R"=w1665:dbl, "G"=w1664:dbl, "B"=w1663:dbl)  [unwired: 1 out]
                          n617 = call "Collision Detection.vi"("Map Entity Objects Positions"=w1654, "Max Player ID number"=w1653, "Moving Object"=w1655) -> ("New Vector"=w1656:T30)  [unwired: 1 out]
                          n618 = Unbundle By Name(w1656) -> ("New Vector Scalar"=w1676:dbl, "New Vector Theta"=w1677:dbl)
                          n619 = Sine & Cosine(0:w1677) -> (1:w1675:dbl, 2:w1674:dbl)
                          n620 = Multiply(x=w1676, y=w1674) -> (x*y=w1658:dbl)
                          n621 = Negate(x=w1658) -> (-x=w1657:dbl)
                          n622 = Add(x=w1657, y=w1673) -> (x+y=w1672:dbl)
                          n623 = Multiply(x=w1676, y=w1675) -> (x*y=w1660:dbl)
                          n624 = Add(x=w1660, y=w1661) -> (x+y=w1671:dbl)
                          n625 = Bundle(w1672, w1671, "Object type"=w1670, "Radius"=w1669, "Width"=w1668, "Height"=w1667, "Move info"=w1659, "HP"=w1666, "R"=w1665, "G"=w1664, "B"=w1663) -> (w1662:T31)  [unwired: 1 in]
                          n626 = Replace Array Subset(array=w1654, new element=w1662, index=w1679) -> (w1680:T8)
                        }
                      }
                    }
                  }
                }
              }
            }
            n627 = local read "Player HP Healing (And visibility)"() -> (w1359:i32[])
            n628 = Array Size(array=w1355) -> (size(s)=w1370:i32)
            n629 = Increment(x=w1354) -> (x+1=w1353:i32)
            n630 = Greater Or Equal?(x=w1370, y=1) -> (x >= y?=w1371:bool)
            n631 = for {
              tunnel: w1359 -> [w1398] mode=indexing
              shift-right: [w1401] -> w1357
              shift-left: w1358 -> [w1400]
              i -> [w1399]
              n632 = Equal?(x=w1398, y=0) -> (x = y?=w1402:bool)
              n633 = case shown="True" w1402 {
                tunnel: [w1416 w1433] -> w1401
                tunnel: w1400 -> [w1419 w1432]
                tunnel: w1399 -> [w1418 w1430]
                tunnel: w1398 -> [w1421 _]
                frame False {
                  n634 = local read "Player HP Healing (And visibility)"() -> (w1422:i32[])
                  n635 = Index Array(array=w1419, index=w1418) -> (element=w1415:T5)
                  n636 = Decrement(x=w1421) -> (x-1=w1420:i32)
                  n637 = Unbundle(w1415) -> ("X"=w1417:dbl, "Y"=w1413:dbl, "Object type"=w1412:dbl, "Radius"=w1411:dbl, "Height"=w1410:dbl, "Theta"=w1409:dbl, "HP"=w1408:dbl, "R"=w1405:dbl, "G"=w1407:dbl, "B"=w1406:dbl)  [unwired: 1 out]
                  n638 = Replace Array Subset(array=w1422, new element=w1420, index=w1418) -> (w1423:i32[])
                  n639 = local write "Player HP Healing (And visibility)"(w1423) -> ()
                  n640 = Bundle("X"=w1417, "Y"=w1413, "Object type"=w1412, "Radius"=w1411, "y"=1.0, "Height"=w1410, "Theta"=w1409, "HP"=w1408, "R"=w1405, "G"=w1407, "B"=w1406) -> (w1414:T32)  [unwired: 1 in]
                  n641 = Replace Array Subset(array=w1419, new element=w1414, index=w1418) -> (w1416:T8)
                }
                frame True {
                  # "Width of Player Object represent one visibility factor"
                  n642 = Index Array(array=w1432, index=w1430) -> (element=w1429:T5)
                  n643 = Unbundle By Name(w1429) -> ("HP"=w1428:dbl)
                  n644 = Less?(x=w1428, y=300.0) -> (x < y?=w1425:bool)
                  n645 = Greater?(x=w1428, y=0.0) -> (0:w1424:bool)
                  n646 = And(x=w1425, y=w1424) -> (x .and. y?=w1426:bool)
                  n647 = case shown="True" w1426 {
                    tunnel: [w1437 w1466] -> w1433
                    tunnel: w1432 -> [w1438 w1467]
                    tunnel: w1430 -> [w1435 w1465]
                    tunnel: w1429 -> [w1436 w1464]
                    frame False {
                      n648 = Unbundle(w1436) -> ("X"=w1441:dbl, "Y"=w1442:dbl, "Object type"=w1444:dbl, "Radius"=w1443:dbl, "Height"=w1445:dbl, "Theta"=w1446:dbl, "HP"=w1434:dbl, "R"=w1447:dbl, "G"=w1448:dbl, "B"=w1449:dbl)  [unwired: 1 out]
                      n649 = Bundle("X"=w1441, "Y"=w1442, "Object type"=w1444, "Radius"=w1443, "y"=0.0, "Height"=w1445, "Theta"=w1446, "HP"=w1434, "R"=w1447, "G"=w1448, "B"=w1449) -> (w1440:T32)  [unwired: 1 in]
                      n650 = Replace Array Subset(array=w1438, new element=w1440, index=w1435) -> (w1437:T8)
                    }
                    frame True {
                      # "Healing HP"
                      n651 = Unbundle(w1464) -> ("X"=w1455:dbl, "Y"=w1456:dbl, "Object type"=w1458:dbl, "Radius"=w1457:dbl, "Height"=w1459:dbl, "Theta"=w1460:dbl, "HP"=w1452:dbl, "R"=w1461:dbl, "G"=w1462:dbl, "B"=w1463:dbl)  [unwired: 1 out]
                      n652 = Add(x=w1452, y=0.5) -> (x+y=w1453:dbl)
                      n653 = Bundle("X"=w1455, "Y"=w1456, "Object type"=w1458, "Radius"=w1457, "y"=0.0, "Height"=w1459, "Theta"=w1460, w1453, "R"=w1461, "G"=w1462, "B"=w1463) -> (w1454:T33)  [unwired: 1 in]
                      n654 = Replace Array Subset(array=w1467, new element=w1454, index=w1465) -> (w1466:T8)
                    }
                  }
                }
              }
            }
            n655 = for {
              N: w1353 -> [_]
              tunnel: w1355 -> [_]
              i -> [w1386]
              n656 = local read "Player info"() -> (w1387:T6)
              n657 = Index Array(array=w1387, index=w1386) -> (element=w1397:T26)
              n658 = Unbundle(w1397) -> ("Kills"=w1393:dbl, "Name"=w1392:string, "Rank"=w1391:dbl, "Who Kill Me"=w1390:dbl, "After Kill"=w1395:dbl)
              n659 = Greater Than 0?(x=w1395) -> (x > 0?=w1396:bool)
              n660 = Decrement(x=w1395) -> (x-1=w1394:dbl)
              n661 = Select(t=w1394, s=w1396, f=w1395) -> (s? t:f=w1389:dbl)
              n662 = Bundle("Kills"=w1393, "Name"=w1392, "Rank"=w1391, "Who Kill Me"=w1390, "After Kill"=w1389) -> (w1388:T26)  [unwired: 1 in]
              n663 = Replace Array Subset(array=w1387, new element=w1388, index=w1386) -> (w1385:T6)
              n664 = local write "Player info"(w1385) -> ()
            }
            n665 = case shown="True" w1371 {
              tunnel: w1357 -> [w1532 w1535]
              tunnel: w1355 -> [_ w1534]
              tunnel: [w1532 w1533] -> w1351
              frame False {
              }
              frame True {
                n666 = for {
                  shift-right: [w1537] -> w1533
                  shift-left: w1535 -> [w1543]
                  tunnel: w1534 -> [w1542] mode=indexing
                  w1538 = 0.0
                  n667 = Unbundle(w1542) -> ("X"=w1540:dbl, "Y"=w1539:dbl)  [unwired: 4 out]
                  n668 = Bundle("X"=w1540, "Y"=w1539, 5.0, w1538, w1538, w1538, w1538, w1538, w1538, w1538, w1538) -> (w1541:T34)  [unwired: 1 in]
                  n669 = Build Array (concatenate)(w1543, w1541) -> (w1537:T8)
                }
              }
            }
            n670 = call <vilib>:"High Resolution Relative Seconds.vi"() -> ("relative seconds"=w1378:dbl)
            n671 = call <vilib>:"High Resolution Relative Seconds.vi"() -> ("relative seconds"=w1375:dbl)
            n672 = feedback #2(w1375) -> (w1379:dbl)
            n673 = feedback-in #2(w1378) -> ()
            n674 = Lossy Enqueue Element(queue=w1381, element=w1351) -> ()  [unwired: 1 in, 4 out]
            n675 = Lossy Enqueue Element(queue=w1352, element=w1351) -> ()  [unwired: 1 in, 4 out]
            n676 = Subtract(x=w1378, y=w1379) -> (x-y=w1380:dbl)
            n677 = Divide(x=1.0, y=w1380) -> (x/y=→"Physic Engine frequency (Hz)":dbl)
            n678 = local read "STOP (會卡住)"() -> (w1384:bool)
          }
          n679 = Equal?(x=w843, y="Map 2") -> (x = y?=w841:bool)
          n680 = call <vilib>:"RGB to Color.vi"("B"=u8 17, "G"=u8 149, "R"=u8 227) -> ("Color"=w844:u32)
          n681 = Select(t=w844, s=w841, f=u32 13828024 ("color(black)")) -> (s? t:f=w848:u32)
          n682 = while {
            tunnel: w881 -> [w1767]
            tunnel: w873 -> [w1714]
            tunnel: w882 -> [w1755]
            tunnel: w854 -> [w1747]
            tunnel: w865 -> [w1682]
            tunnel: w848 -> [w1681]
            i -> [w1746]
            stop <- w1766 stop-if-true
            # "States shading (rank, bulllets, kills...etc)"
            # "If it is ML player mode, send info to ML player.vi"
            # "Analize the scene info of main player"
            # "Play data collection"
            # "Shade Other Objects"
            # "Shade bullet first!"
            # "Refresh Speed limit"
            n683 = local read "電腦代打模式:\n(Based on Machine Learning)\n(Behavior cloning)\n(Warning: High computing workload)"() -> (w1684:bool)
            n684 = call <vilib>:"Draw Rectangle.vi"("picture"=picture data[5B], "rect"=T11 {"left"=0, "top"=0, "right"=1280, "bottom"=720}, "fill?(F)"=TRUE, "color(black)"=w1681) -> ("new picture"=w1751:picture)  [unwired: 5 in]
            n685 = Dequeue Element(queue=w1767) -> (element=w1683:T8)  [unwired: 2 in, 3 out]
            n686 = for {
              tunnel: w1755 -> [w1956] mode=indexing
              tunnel: w1683 -> [w1955]
              # "Send processed data to AI Player"
              n687 = Lossy Enqueue Element(queue=w1956, element=w1955) -> ()  [unwired: 1 in, 4 out]
            }
            n688 = Array Size(array=w1683) -> (size(s)=w1754:i32)
            n689 = case shown="True" w1684 {
              tunnel: w1683 -> [_ w1769]
              tunnel: w1682 -> [_ w1768]
              frame False {
              }
              frame True {
                n690 = Lossy Enqueue Element(queue=w1768, element=w1769) -> ()  [unwired: 1 in, 4 out]
              }
            }
            n691 = Index Array(array=w1683, index=0) -> (element=w1750:T5)
            "MainPlayer" <- w1750
            n692 = call "Scene info analyzer.vi"("Map Entity Object Position"=w1683, "Current Player ID"=0, "Max Player ID"=w1714) -> ("Enemy on 8 directions"=w1699:T2, "Closest valid target"=→"Closest valid target":T3, "Farther Bullets on 8 directions"=w1700:T2, "Closer Bullets on 8 directions"=w1701:T2, "Current Player HP"=w1694:dbl, "Object on 8 directions"=w1702:T2)
            "Current Player HP" <- w1694
            "Object on 8 directions" <- w1702
            "Closer Bullets on 8 directions" <- w1701
            "Farther Bullets on 8 directions" <- w1700
            "Enemy on 8 directions" <- w1699
            n693 = Wait (ms)(milliseconds to wait=u32 16) -> ()  [unwired: 1 out]
            n694 = Subtract(x=w1754, y=w1747) -> (x-y=w1748:i32)
            n695 = Greater Or Equal?(x=w1748, y=1) -> (x >= y?=w1753:bool)
            n696 = local read "Sent command"() -> (w1693:T4)
            n697 = case shown="True" w1753 {
              tunnel: w1751 -> [w1914 w1920]
              tunnel: w1750 -> [_ w1919]
              tunnel: [w1914 w1918] -> w1749
              tunnel: w1748 -> [_ w1917]
              tunnel: w1683 -> [_ w1916]
              tunnel: w1747 -> [_ w1915]
              frame False {
              }
              frame True {
                n698 = for {
                  N: w1917 -> [_]
                  shift-right: [w1925] -> w1918
                  shift-left: w1920 -> [w1924]
                  tunnel: w1919 -> [w1941]
                  tunnel: w1916 -> [w1930]
                  tunnel: w1915 -> [w1928]
                  i -> [w1921]
                  n699 = Add(x=w1928, y=w1921) -> (x+y=w1929:i32)
                  n700 = Index Array(array=w1930, index=w1929) -> (element=w1931:T5)
                  n701 = Unbundle By Name(w1941) -> ("X"=w1934:dbl, "Y"=w1935:dbl)
                  n702 = Unbundle By Name(w1931) -> ("X"=w1927:dbl, "Y"=w1926:dbl)
                  n703 = Subtract(x=w1926, y=w1935) -> (x-y=w1922:dbl)
                  n704 = Subtract(x=w1927, y=w1934) -> (x-y=w1923:dbl)
                  n705 = Absolute Value(x=w1922) -> (abs(x)=w1937:dbl)
                  n706 = Absolute Value(x=w1923) -> (abs(x)=w1936:dbl)
                  n707 = Less?(x=w1936, y=660.0) -> (x < y?=w1932:bool)
                  n708 = Less?(x=w1937, y=380.0) -> (x < y?=w1933:bool)
                  n709 = And(x=w1932, y=w1933) -> (x .and. y?=w1939:bool)
                  n710 = case shown="True" w1939 {
                    tunnel: [w1942 w1945] -> w1925
                    tunnel: w1924 -> [w1942 w1946]
                    tunnel: w1923 -> [_ w1952]
                    tunnel: w1922 -> [_ w1951]
                    frame False {
                    }
                    frame True {
                      n711 = Add(x=w1952, y=640.0) -> (x+y=w1949:dbl)
                      n712 = Add(x=w1951, y=360.0) -> (x+y=w1950:dbl)
                      n713 = Bundle(w1949, w1950) -> (w1948:cluster{dbl, dbl})  [unwired: 1 in]
                      n714 = call <vilib>:"Draw Circle by Radius.vi"("color(black)"=u32 2492672, "fill?(F)"=TRUE, "pixel center"=w1948, "radius"=i16 5, "picture"=w1946) -> ("new picture"=w1945:picture)  [unwired: 6 in]
                    }
                  }
                }
              }
            }
            n715 = Cluster To Array(cluster=w1699) -> (array=w1695:dbl[])
            n716 = Cluster To Array(cluster=w1700) -> (array=w1696:dbl[])
            n717 = Cluster To Array(cluster=w1702) -> (array=w1698:dbl[])
            n718 = Cluster To Array(cluster=w1701) -> (array=w1697:dbl[])
            n719 = Index Array(array=w1693, index=0) -> (element=w1691:T35)
            n720 = Unbundle(w1691) -> ("Vector scalar"=w1690:dbl, "Theta"=w1688:dbl)  [unwired: 4 out]
            n721 = Build Array (concatenate)(w1694, w1698, w1697, w1696, w1695) -> (w1687:dbl[])
            n722 = Equal To 0?(x=w1690) -> (x = 0?=w1689:bool)
            n723 = case shown="True" w1689 {
              tunnel: w1688 -> [w1777 _]
              tunnel: w1687 -> [w1778 w1783]
              tunnel: [w1775 w1781] -> w1686
              frame False {
                n724 = Divide(x=w1777, y=0.785) -> (x/y=w1779:dbl)
                n725 = Round To Nearest(number=w1779) -> (nearest integer value=w1776:dbl)
                n726 = Build Array (concatenate)(w1778, w1776) -> (w1775:dbl[])
              }
              frame True {
                n727 = Build Array (concatenate)(w1783, 8.0) -> (w1781:dbl[])
              }
            }
            n728 = case shown="True" FALSE {
              tunnel: w1686 -> [_ w1772]
              frame False {
              }
              frame True {
                # "Write data into a csv file"
                n729 = call-poly <vilib>:"Write Delimited Spreadsheet.vi"("file path (dialog if empty)"=path "C:/Users/eason/OneDrive/NYCU file/LabVIEW Programming/Final Project/Game/Play Data/Test03.csv", "format (%.3f)"="%d", "1D data"=w1772, "append to file? (new file:F)"=TRUE, "delimiter (\\t)"="," ("delimiter (\\t)")) -> ()  [unwired: 9 in, 2 out]
              }
            }
            n730 = for {
              N: w1747 -> [_]
              tunnel: w1714 -> [w1989]
              tunnel: w1683 -> [w1986]
              tunnel: w1750 -> [w1983]
              shift-right: [w1970] -> w1745
              shift-left: w1749 -> [w1971]
              i -> [w1985]
              n731 = Index Array(array=w1986, index=w1985) -> (element=w1984:T5)
              n732 = Greater Or Equal?(x=w1985, y=20) -> (x >= y?=w1992:bool)
              n733 = Unbundle(w1983) -> ("X"=w1981:dbl, "Y"=w1979:dbl, "HP"=→"MP HP":dbl)  [unwired: 8 out]
              n734 = Less Or Equal?(x=w1985, y=w1989) -> (x <= y?=w1991:bool)
              n735 = Unbundle(w1984) -> ("X"=w1982:dbl, "Y"=w1980:dbl, "Object type"=w1969:dbl, "Radius"=w1963:dbl, "Width"=w1959:dbl, "Height"=w1958:dbl, "Theta"=w1964:dbl, "HP"=w1965:dbl, "R"=w1962:dbl, "G"=w1961:dbl, "B"=w1960:dbl)
              n736 = Or(x=w1991, y=w1992) -> (x .or. y?=w1987:bool)
              n737 = Subtract(x=w1982, y=w1981) -> (x-y=w1966:dbl)
              n738 = Subtract(x=w1980, y=w1979) -> (x-y=w1967:dbl)
              n739 = Absolute Value(x=w1967) -> (abs(x)=w1975:dbl)
              n740 = Absolute Value(x=w1966) -> (abs(x)=w1978:dbl)
              n741 = To Long Integer(number=w1969) -> (32bit integer=w1968:i32)
              n742 = Less?(x=w1975, y=560.0) -> (x < y?=w1973:bool)
              n743 = Less?(x=w1978, y=840.0) -> (x < y?=w1972:bool)
              n744 = And(x=w1972, y=w1973) -> (x .and. y?=w1974:bool)
              n745 = And(x=w1974, y=w1987) -> (x .and. y?=w1988:bool)
              n746 = case shown="True" w1988 {
                tunnel: [w1993 w2000] -> w1970
                tunnel: w1971 -> [w1993 w2003]
                tunnel: w1968 -> [_ w2006]
                tunnel: w1967 -> [_ w2005]
                tunnel: w1966 -> [_ w2004]
                tunnel: w1965 -> [_ w2002]
                tunnel: w1964 -> [_ w2001]
                tunnel: w1963 -> [_ w1999]
                tunnel: w1962 -> [_ w1998]
                tunnel: w1961 -> [_ w1997]
                tunnel: w1960 -> [_ w1996]
                tunnel: w1959 -> [_ w1995]
                tunnel: w1958 -> [_ w1994]
                frame False {
                }
                frame True {
                  n747 = case shown="0, Default" w2006 {
                    tunnel: w2005 -> [w2014 w2187 w2202 w2221 w2237]
                    tunnel: w2004 -> [w2013 w2186 w2201 w2220 w2236]
                    tunnel: w2003 -> [w2011 w2184 w2199 w2215 w2231]
                    tunnel: w2002 -> [w2009 _ _ _ _]
                    tunnel: w2001 -> [w2012 _ _ w2212 w2229]
                    tunnel: [w2007 w2178 w2190 w2209 w2224] -> w2000
                    tunnel: w1999 -> [_ w2177 w2194 _ _]
                    tunnel: w1998 -> [_ w2176 w2193 w2219 w2235]
                    tunnel: w1997 -> [_ w2175 w2192 w2218 w2234]
                    tunnel: w1996 -> [_ w2174 w2191 w2217 w2233]
                    tunnel: w1995 -> [_ _ _ w2206 w2226]
                    tunnel: w1994 -> [_ _ _ w2205 w2225]
                    frame 0, Default {
                      n748 = Greater?(x=w2009, y=0.0) -> (0:w2010:bool)
                      n749 = case shown="False" w2010 {
                        tunnel: w2014 -> [w2071 w2171]
                        tunnel: w2013 -> [w2070 w2170]
                        tunnel: w2009 -> [w2068 w2168]
                        tunnel: [w2037 w2137] -> w2007
                        tunnel: w2012 -> [w2025 w2074]
                        tunnel: w2011 -> [w2017 w2114]
                        frame True {
                          w2028 = 10.0 ("height")
                          w2029 = 55.0 ("width")
                          w2039 = i16 9 ("radius")
                          w2049 = i16 9 ("radius")
                          w2058 = i16 30 ("radius")
                          # "Draw two hand on player"
                          # "Draw the weapon on hand"
                          # "The color of player base on the HP points"
                          n750 = Add(x=w2070, y=640.0) -> (x+y=w2023:dbl)
                          n751 = Add(x=w2071, y=360.0) -> (x+y=w2020:dbl)
                          n752 = Divide(x=w2068, y=4.0) -> (x/y=w2062:dbl)
                          n753 = call "rotation matrix.vi"("angle"=w2025, "y"=0.0, "x"=-55.0) -> ("new y"=w2021:dbl, "new x"=w2024:dbl)
                          n754 = Add(x=w2021, y=w2020) -> (x+y=w2019:dbl)
                          n755 = Add(x=w2024, y=w2023) -> (x+y=w2022:dbl)
                          n756 = Bundle(w2023, w2020) -> (w2057:cluster{dbl, dbl})  [unwired: 1 in]
                          n757 = Add(x=w2062, y=180.0) -> (x+y=w2066:dbl)
                          n758 = Add(x=w2062, y=140.0) -> (x+y=w2065:dbl)
                          n759 = Add(x=w2062, y=85.0) -> (x+y=w2064:dbl)
                          n760 = call "draw rotated rectangle.vi"("fill"=TRUE, "Color Box"=u32 3684408, "angle"=w2025, "2D Picture"=w2017, "height"=w2028, "width"=w2029, "y"=w2019, "x"=w2022) -> ("new picture"=w2030:picture)  [unwired: 3 in]
                          n761 = call <vilib>:"RGB to Color.vi"("B"=w2064, "G"=w2065, "R"=w2066) -> ("Color"=w2034:u32)
                          n762 = call "draw rotated rectangle.vi"("fill"=FALSE, "Color Box"=u32 0, "angle"=w2025, "2D Picture"=w2030, "height"=w2028, "width"=w2029, "y"=w2019, "x"=w2022) -> ("new picture"=w2015:picture)  [unwired: 3 in]
                          n763 = call <vilib>:"Draw Circle by Radius.vi"("color(black)"=w2034, "fill?(F)"=TRUE, "pixel center"=w2057, "radius"=w2058, "picture"=w2015) -> ("new picture"=w2059:picture)  [unwired: 6 in]
                          n764 = call <vilib>:"Draw Circle by Radius.vi"("pixel center"=w2057, "radius"=w2058, "picture"=w2059) -> ("new picture"=w2016:picture)  [unwired: 8 in]
                          n765 = call "rotation matrix.vi"("angle"=w2025, "y"=-8.0, "x"=-35.0) -> ("new y"=w2050:dbl, "new x"=w2051:dbl)
                          n766 = Add(x=w2020, y=w2050) -> (x+y=w2053:dbl)
                          n767 = Add(x=w2023, y=w2051) -> (x+y=w2054:dbl)
                          n768 = Bundle(w2054, w2053) -> (w2047:cluster{dbl, dbl})  [unwired: 1 in]
                          n769 = call <vilib>:"Draw Circle by Radius.vi"("color(black)"=w2034, "fill?(F)"=TRUE, "pixel center"=w2047, "radius"=w2049, "picture"=w2016) -> ("new picture"=w2048:picture)  [unwired: 6 in]
                          n770 = call "rotation matrix.vi"("angle"=w2025, "y"=8.0, "x"=-40.0) -> ("new y"=w2035:dbl, "new x"=w2036:dbl)
                          n771 = call <vilib>:"Draw Circle by Radius.vi"("pixel center"=w2047, "radius"=w2049, "picture"=w2048) -> ("new picture"=w2038:picture)  [unwired: 8 in]
                          n772 = Add(x=w2023, y=w2036) -> (x+y=w2041:dbl)
                          n773 = Add(x=w2020, y=w2035) -> (x+y=w2042:dbl)
                          n774 = Bundle(w2041, w2042) -> (w2040:cluster{dbl, dbl})  [unwired: 1 in]
                          n775 = call <vilib>:"Draw Circle by Radius.vi"("color(black)"=w2034, "fill?(F)"=TRUE, "pixel center"=w2040, "radius"=w2039, "picture"=w2038) -> ("new picture"=w2046:picture)  [unwired: 6 in]
                          n776 = call <vilib>:"Draw Circle by Radius.vi"("pixel center"=w2040, "radius"=w2039, "picture"=w2046) -> ("new picture"=w2037:picture)  [unwired: 8 in]
                        }
                        frame False {
                          w2128 = 10.0 ("height")
                          w2129 = 55.0 ("width")
                          w2139 = i16 9 ("radius")
                          w2149 = i16 9 ("radius")
                          w2158 = i16 30 ("radius")
                          # "Draw two hand on player"
                          # "Draw the weapon on hand"
                          # "The color of player base on the HP points"
                          n777 = Add(x=w2170, y=640.0) -> (x+y=w2077:dbl)
                          n778 = Add(x=w2171, y=360.0) -> (x+y=w2078:dbl)
                          n779 = call "rotation matrix.vi"("angle"=w2074, "y"=-5.0, "x"=-22.0 ("y")) -> ("new y"=w2105:dbl, "new x"=w2106:dbl)
                          n780 = Add(x=w2077, y=w2106) -> (x+y=w2112:dbl)
                          n781 = Add(x=w2078, y=w2105) -> (x+y=w2111:dbl)
                          n782 = Divide(x=w2168, y=4.0) -> (x/y=w2162:dbl)
                          n783 = Bundle(w2112, w2111) -> (w2104:cluster{dbl, dbl})  [unwired: 1 in]
                          n784 = call <vilib>:"Draw Circle by Radius.vi"("color(black)"=u32 16711680, "fill?(F)"=TRUE, "pixel center"=w2104, "radius"=i16 24, "picture"=w2114) -> ("new picture"=w2097:picture)  [unwired: 6 in]
                          n785 = Bundle(w2077, w2078) -> (w2157:cluster{dbl, dbl})  [unwired: 1 in]
                          n786 = Add(x=w2074, y=0.5) -> (x+y=w2094:dbl)
                          n787 = Add(x=w2162, y=180.0) -> (x+y=w2166:dbl)
                          n788 = call "rotation matrix.vi"("angle"=w2094, "y"=5.0, "x"=-24.0) -> ("new y"=w2091:dbl, "new x"=w2092:dbl)
                          n789 = Add(x=w2162, y=140.0) -> (x+y=w2165:dbl)
                          n790 = Add(x=w2162, y=85.0) -> (x+y=w2164:dbl)
                          n791 = Add(x=w2077, y=w2092) -> (x+y=w2102:dbl)
                          n792 = Add(x=w2078, y=w2091) -> (x+y=w2101:dbl)
                          n793 = Add(x=w2074, y=-0.1) -> (x+y=w2117:dbl)
                          n794 = call <vilib>:"RGB to Color.vi"("B"=w2164, "G"=w2165, "R"=w2166) -> ("Color"=w2134:u32)
                          n795 = Add(x=w2074, y=-1.75) -> (x+y=w2075:dbl)
                          n796 = Bundle(w2102, w2101) -> (w2098:cluster{dbl, dbl})  [unwired: 1 in]
                          n797 = call <vilib>:"Draw Circle by Radius.vi"("color(black)"=u32 16711680, "fill?(F)"=TRUE, "pixel center"=w2098, "radius"=i16 20, "picture"=w2097) -> ("new picture"=w2084:picture)  [unwired: 6 in]
                          n798 = call "rotation matrix.vi"("angle"=w2075, "y"=5.0, "x"=-27.0) -> ("new y"=w2079:dbl, "new x"=w2080:dbl)
                          n799 = call "rotation matrix.vi"("angle"=w2117, "y"=-8.0, "x"=-40.0) -> ("new y"=w2150:dbl, "new x"=w2151:dbl)
                          n800 = Add(x=w2077, y=w2080) -> (x+y=w2089:dbl)
                          n801 = Add(x=w2078, y=w2079) -> (x+y=w2088:dbl)
                          n802 = Bundle(w2089, w2088) -> (w2085:cluster{dbl, dbl})  [unwired: 1 in]
                          n803 = call <vilib>:"Draw Circle by Radius.vi"("color(black)"=u32 16711680, "fill?(F)"=TRUE, "pixel center"=w2085, "radius"=i16 7, "picture"=w2084) -> ("new picture"=w2083:picture)  [unwired: 6 in]
                          n804 = Add(x=w2078, y=w2150) -> (x+y=w2153:dbl)
                          n805 = Add(x=w2077, y=w2151) -> (x+y=w2154:dbl)
                          n806 = Bundle(w2154, w2153) -> (w2147:cluster{dbl, dbl})  [unwired: 1 in]
                          n807 = Add(x=w2074, y=0.5) -> (x+y=w2118:dbl)
                          n808 = call "rotation matrix.vi"("angle"=w2074, "y"=10.0, "x"=-50.0) -> ("new y"=w2135:dbl, "new x"=w2136:dbl)
                          n809 = call "rotation matrix.vi"("angle"=w2074, "y"=0.0, "x"=-55.0) -> ("new y"=w2123:dbl, "new x"=w2125:dbl)
                          n810 = Add(x=w2123, y=w2078) -> (x+y=w2122:dbl)
                          n811 = Add(x=w2125, y=w2077) -> (x+y=w2124:dbl)
                          n812 = Add(x=w2077, y=w2136) -> (x+y=w2141:dbl)
                          n813 = Add(x=w2078, y=w2135) -> (x+y=w2142:dbl)
                          n814 = call "draw rotated rectangle.vi"("fill"=TRUE, "Color Box"=u32 3684408, "angle"=w2118, "2D Picture"=w2083, "height"=w2128, "width"=w2129, "y"=w2122, "x"=w2124) -> ("new picture"=w2130:picture)  [unwired: 3 in]
                          n815 = Bundle(w2141, w2142) -> (w2140:cluster{dbl, dbl})  [unwired: 1 in]
                          n816 = call "draw rotated rectangle.vi"("fill"=FALSE, "Color Box"=u32 0, "angle"=w2118, "2D Picture"=w2130, "height"=w2128, "width"=w2129, "y"=w2122, "x"=w2124) -> ("new picture"=w2119:picture)  [unwired: 3 in]
                          n817 = call <vilib>:"Draw Circle by Radius.vi"("color(black)"=w2134, "fill?(F)"=TRUE, "pixel center"=w2157, "radius"=w2158, "picture"=w2119) -> ("new picture"=w2159:picture)  [unwired: 6 in]
                          n818 = call <vilib>:"Draw Circle by Radius.vi"("pixel center"=w2157, "radius"=w2158, "picture"=w2159) -> ("new picture"=w2120:picture)  [unwired: 8 in]
                          n819 = call <vilib>:"Draw Circle by Radius.vi"("color(black)"=w2134, "fill?(F)"=TRUE, "pixel center"=w2147, "radius"=w2149, "picture"=w2120) -> ("new picture"=w2148:picture)  [unwired: 6 in]
                          n820 = call <vilib>:"Draw Circle by Radius.vi"("pixel center"=w2147, "radius"=w2149, "picture"=w2148) -> ("new picture"=w2138:picture)  [unwired: 8 in]
                          n821 = call <vilib>:"Draw Circle by Radius.vi"("color(black)"=w2134, "fill?(F)"=TRUE, "pixel center"=w2140, "radius"=w2139, "picture"=w2138) -> ("new picture"=w2146:picture)  [unwired: 6 in]
                          n822 = call <vilib>:"Draw Circle by Radius.vi"("pixel center"=w2140, "radius"=w2139, "picture"=w2146) -> ("new picture"=w2137:picture)  [unwired: 8 in]
                        }
                      }
                    }
                    frame 1 {
                      n823 = Add(x=w2186, y=640.0) -> (x+y=w2180:dbl)
                      n824 = Add(x=w2187, y=360.0) -> (x+y=w2179:dbl)
                      n825 = Bundle(w2180, w2179) -> (w2182:cluster{dbl, dbl})  [unwired: 1 in]
                      n826 = call <vilib>:"RGB to Color.vi"("B"=w2174, "G"=w2175, "R"=w2176) -> ("Color"=w2181:u32)
                      n827 = call <vilib>:"Draw Circle by Radius.vi"("color(black)"=w2181, "fill?(F)"=TRUE, "pixel center"=w2182, "radius"=w2177, "picture"=w2184) -> ("new picture"=w2183:picture)  [unwired: 6 in]
                      n828 = call <vilib>:"Draw Circle by Radius.vi"("pixel center"=w2182, "radius"=w2177, "picture"=w2183) -> ("new picture"=w2178:picture)  [unwired: 8 in]
                    }
                    frame 3 {
                      n829 = Add(x=w2201, y=640.0) -> (x+y=w2196:dbl)
                      n830 = Add(x=w2202, y=360.0) -> (x+y=w2195:dbl)
                      n831 = Bundle(w2196, w2195) -> (w2198:cluster{dbl, dbl})  [unwired: 1 in]
                      n832 = call <vilib>:"RGB to Color.vi"("B"=w2191, "G"=w2192, "R"=w2193) -> ("Color"=w2197:u32)
                      n833 = call <vilib>:"Draw Circle by Radius.vi"("color(black)"=w2197, "fill?(F)"=TRUE, "pixel center"=w2198, "radius"=w2194, "picture"=w2199) -> ("new picture"=w2190:picture)  [unwired: 6 in]
                    }
                    frame 2 {
                      n834 = Add(x=w2220, y=640.0) -> (x+y=w2208:dbl)
                      n835 = Add(x=w2221, y=360.0) -> (x+y=w2207:dbl)
                      n836 = call <vilib>:"RGB to Color.vi"("B"=w2217, "G"=w2218, "R"=w2219) -> ("Color"=w2214:u32)
                      n837 = call "draw rotated rectangle.vi"("fill"=TRUE, "Color Box"=w2214, "angle"=w2212, "2D Picture"=w2215, "height"=w2205, "width"=w2206, "y"=w2207, "x"=w2208) -> ("new picture"=w2210:picture)  [unwired: 3 in]
                      n838 = call "draw rotated rectangle.vi"("fill"=FALSE, "Color Box"=u32 0, "angle"=w2212, "2D Picture"=w2210, "height"=w2205, "width"=w2206, "y"=w2207, "x"=w2208) -> ("new picture"=w2209:picture)  [unwired: 3 in]
                    }
                    frame 4 {
                      n839 = Add(x=w2236, y=640.0) -> (x+y=w2228:dbl)
                      n840 = Add(x=w2237, y=360.0) -> (x+y=w2227:dbl)
                      n841 = call <vilib>:"RGB to Color.vi"("B"=w2233, "G"=w2234, "R"=w2235) -> ("Color"=w2230:u32)
                      n842 = call "draw rotated rectangle.vi"("fill"=TRUE, "Color Box"=w2230, "angle"=w2229, "2D Picture"=w2231, "height"=w2225, "width"=w2226, "y"=w2227, "x"=w2228) -> ("new picture"=w2224:picture)  [unwired: 3 in]
                    }
                  }
                }
              }
            }
            n843 = local read "Player Bullets"() -> (w1738:i32[])
            n844 = local read "Player Bullets Reload"() -> (w1734:i32[])
            n845 = Index Array(array=w1738, index=0) -> (element=w1737:i32)
            n846 = call <vilib>:"High Resolution Relative Seconds.vi"() -> ("relative seconds"=w1762:dbl)
            n847 = Number To Decimal String(number=w1737) -> (decimal integer string=w1736:string)  [unwired: 1 in]
            n848 = feedback #3(u32 0 ("millisecond timer value")) -> (w1763:dbl)
            n849 = feedback-in #3(w1762) -> ()
            n850 = Index Array(array=w1734, index=0) -> (element=w1730:i32)
            n851 = Subtract(x=w1762, y=w1763) -> (x-y=w1764:dbl)
            n852 = call <vilib>:"Draw Text at Point.vi"("[user-specified font]"=T14 {"Font Name:"="Arial", "Size"=36, "Strikeout?"=FALSE, "Italic?"=FALSE, "Underline?"=FALSE, "Outline?"=FALSE, "Shadow?"=TRUE, "Bold?"=TRUE}, "text color(black)"=u32 0, "desired font(Application)"=T13."User-specified Font", "text"=w1736, "alignment(left, top)"=T15 {"horizontal"=enum."left", "vertical"=enum."top"}, "origin"=cluster{"x":i16, "y":i16} {"x"=860, "y"=635}, "picture"=w1745) -> ("new picture"=w1731:picture)  [unwired: 3 in, 1 out]
            n853 = Divide(x=1.0, y=w1764) -> (x/y=w1759:dbl)
            n854 = local write "FPS"(w1759) -> ()
            n855 = Greater?(x=w1730, y=4) -> (0:w1732:bool)
            n856 = case shown="True" w1732 {
              tunnel: [w1891 w1908] -> w1728
              tunnel: w1731 -> [w1891 w1913]
              tunnel: w1730 -> [_ w1906]
              frame False {
              }
              frame True {
                w1903 = cluster{"x":i16, "y":i16} {"x"=640, "y"=580} ("origin")
                n857 = Divide(x=w1906, y=120) -> (x/y=w1893:dbl)
                n858 = Multiply(x=w1893, y=360.0) -> (x*y=w1900:dbl)
                n859 = call <vilib>:"Draw Circle by Radius.vi"("arc size(360)"=w1900, "color(black)"=u32 13816530, "fill?(F)"=TRUE, "pixel center"=w1903, "radius"=i16 50, "picture"=w1913) -> ("new picture"=w1907:picture)  [unwired: 5 in]
                n860 = Multiply(x=w1893, y=2.0) -> (x*y=w1894:dbl)
                n861 = Number To Fractional String(number=w1894, precision (6)=i16 1) -> (F-format string=w1896:string)  [unwired: 2 in]
                n862 = Concatenate Strings("Reloading...\n      ", w1896) -> (w1898:string)
                n863 = call <vilib>:"Draw Text at Point.vi"("[user-specified font]"=T14 {"Font Name:"="Arial", "Size"=24, "Strikeout?"=FALSE, "Italic?"=FALSE, "Underline?"=FALSE, "Outline?"=FALSE, "Shadow?"=TRUE, "Bold?"=TRUE}, "text color(black)"=u32 0, "desired font(Application)"=T13."User-specified Font", "text"=w1898, "alignment(left, top)"=T15 {"horizontal"=enum."center", "vertical"=enum."center"}, "origin"=w1903, "picture"=w1907) -> ("new picture"=w1908:picture)  [unwired: 3 in, 1 out]
              }
            }
            n864 = local read "STOP (會卡住)"() -> (w1766:bool)
            n865 = local read "Player info"() -> (w1729:T6)
            n866 = Sort 1D Array(array=w1729) -> (sorted array=w1727:T6)
            n867 = Reverse 1D Array(array=w1727) -> (reversed array=w1726:T6)
            n868 = for {
              tunnel: w1726 -> [w1883] mode=indexing
              shift-right: [w1878] -> w1721
              shift-left: w1728 -> [w1884]
              i -> [w1869]
              stop <- w1890 stop-if-true
              n869 = Unbundle(w1883) -> ("Kills"=w1875:dbl, "Name"=w1876:string)  [unwired: 3 out]
              n870 = Multiply(x=32, y=w1869) -> (x*y=w1867:i32)
              n871 = Add(x=24, y=w1867) -> (x+y=w1865:i32)
              n872 = Bundle(24, w1865) -> (w1873:cluster{i32, i32})  [unwired: 1 in]
              n873 = call <vilib>:"Draw Text at Point.vi"("[user-specified font]"=T14 {"Font Name:"="Arial", "Size"=24, "Strikeout?"=FALSE, "Italic?"=FALSE, "Underline?"=FALSE, "Outline?"=FALSE, "Shadow?"=TRUE, "Bold?"=TRUE}, "text color(black)"=u32 0, "desired font(Application)"=T13."User-specified Font", "text"=w1876, "alignment(left, top)"=T15 {"horizontal"=enum."left", "vertical"=enum."center"}, "origin"=w1873, "picture"=w1884) -> ("new picture"=w1877:picture)  [unwired: 3 in, 1 out]
              n874 = Number To Decimal String(number=w1875) -> (decimal integer string=w1874:string)  [unwired: 1 in]
              n875 = Bundle(210, w1865) -> (w1872:cluster{i32, i32})  [unwired: 1 in]
              n876 = Greater?(x=w1869, y=3) -> (0:w1890:bool)
              n877 = call <vilib>:"Draw Text at Point.vi"("[user-specified font]"=T14 {"Font Name:"="Arial", "Size"=24, "Strikeout?"=FALSE, "Italic?"=FALSE, "Underline?"=FALSE, "Outline?"=FALSE, "Shadow?"=TRUE, "Bold?"=TRUE}, "text color(black)"=u32 0, "desired font(Application)"=T13."User-specified Font", "text"=w1874, "alignment(left, top)"=T15 {"horizontal"=enum."left", "vertical"=enum."center"}, "origin"=w1872, "picture"=w1877) -> ("new picture"=w1878:picture)  [unwired: 3 in, 1 out]
            }
            n878 = local read "Alive number"() -> (w1720:i32)
            n879 = Number To Decimal String(number=w1720) -> (decimal integer string=w1718:string)  [unwired: 1 in]
            n880 = Concatenate Strings("Alive: " ("string"), w1718) -> (w1719:string)
            n881 = call <vilib>:"Draw Text at Point.vi"("[user-specified font]"=T14 {"Font Name:"="Arial", "Size"=42, "Strikeout?"=FALSE, "Italic?"=FALSE, "Underline?"=FALSE, "Outline?"=FALSE, "Shadow?"=TRUE, "Bold?"=TRUE}, "text color(black)"=u32 0, "desired font(Application)"=T13."User-specified Font", "text"=w1719, "alignment(left, top)"=T15 {"horizontal"=enum."left", "vertical"=enum."center"}, "origin"=cluster{"x":i16, "y":i16} {"x"=1080, "y"=40}, "picture"=w1721) -> ("new picture"=w1712:picture)  [unwired: 3 in, 1 out]
            n882 = local read "MP HP"() -> (w1710:dbl)
            n883 = Less Or Equal?(x=w1710, y=0.0) -> (x <= y?=w1711:bool)
            n884 = case shown="True" w1711 {
              tunnel: w1712 -> [w1808 w1835]
              tunnel: [w1808 w1814] -> w1705
              frame False {
              }
              frame True {
                # "If main player have been killed, shade player info thereupon."
                n885 = local read "Player info"() -> (w1831:T6)
                n886 = Index Array(array=w1831, index=0) -> (element=w1833:T26)
                n887 = Unbundle(w1833) -> ("Kills"=w1810:dbl, "Rank"=w1816:dbl, "Who Kill Me"=w1832:dbl, "After Kill"=w1811:dbl)  [unwired: 1 out]
                n888 = call <vilib>:"Draw Text at Point.vi"("[user-specified font]"=T14 {"Font Name:"="Arial", "Size"=56, "Strikeout?"=FALSE, "Italic?"=FALSE, "Underline?"=TRUE, "Outline?"=FALSE, "Shadow?"=TRUE, "Bold?"=TRUE}, "text color(black)"=u32 16711699, "desired font(Application)"=T13."User-specified Font", "text"="你已陣亡!", "alignment(left, top)"=T15 {"horizontal"=enum."center", "vertical"=enum."center"}, "origin"=cluster{"x":i16, "y":i16} {"x"=640, "y"=150}, "picture"=w1835) -> ("new picture"=w1820:picture)  [unwired: 3 in, 1 out]
                n889 = Index Array(array=w1831, index=w1832) -> (element=w1830:T26)
                n890 = local write "Background music"(2.0 ("Background music")) -> ()
                n891 = Unbundle(w1830) -> ("Name"=w1828:string)  [unwired: 4 out]
                n892 = Concatenate Strings(w1828, " 選擇對你痛下殺手" ("string")) -> (w1821:string)
                n893 = call <vilib>:"Draw Text at Point.vi"("[user-specified font]"=T14 {"Font Name:"="Arial", "Size"=42, "Strikeout?"=FALSE, "Italic?"=FALSE, "Underline?"=FALSE, "Outline?"=FALSE, "Shadow?"=TRUE, "Bold?"=TRUE}, "text color(black)"=u32 5064, "desired font(Application)"=T13."User-specified Font", "text"=w1821, "alignment(left, top)"=T15 {"horizontal"=enum."center", "vertical"=enum."center"}, "origin"=cluster{"x":i16, "y":i16} {"x"=640, "y"=210}, "picture"=w1820) -> ("new picture"=w1817:picture)  [unwired: 3 in, 1 out]
                n894 = Less?(x=w1811, y=400.0) -> (x < y?=w1818:bool)
                n895 = case shown="True" w1818 {
                  tunnel: w1817 -> [w1853 w1856]
                  tunnel: [w1853 w1855] -> w1815
                  tunnel: w1816 -> [_ w1854]
                  frame False {
                  }
                  frame True {
                    n896 = Number To Decimal String(number=w1854) -> (decimal integer string=w1857:string)  [unwired: 1 in]
                    n897 = Concatenate Strings("Rank: " ("text"), w1857) -> (w1858:string)
                    n898 = call <vilib>:"Draw Text at Point.vi"("[user-specified font]"=T14 {"Font Name:"="Arial", "Size"=42, "Strikeout?"=FALSE, "Italic?"=FALSE, "Underline?"=FALSE, "Outline?"=FALSE, "Shadow?"=TRUE, "Bold?"=TRUE}, "text color(black)"=u32 16764482, "desired font(Application)"=T13."User-specified Font", "text"=w1858, "alignment(left, top)"=T15 {"horizontal"=enum."center", "vertical"=enum."center"}, "origin"=cluster{"x":i16, "y":i16} {"x"=450, "y"=270}, "picture"=w1856) -> ("new picture"=w1855:picture)  [unwired: 3 in, 1 out]
                  }
                }
                n899 = Less?(x=w1811, y=200.0) -> (x < y?=w1812:bool)
                n900 = case shown="True" w1812 {
                  tunnel: w1815 -> [w1841 w1844]
                  tunnel: [w1841 w1843] -> w1814
                  tunnel: w1810 -> [_ w1842]
                  frame False {
                  }
                  frame True {
                    n901 = Number To Decimal String(number=w1842) -> (decimal integer string=w1845:string)  [unwired: 1 in]
                    n902 = Concatenate Strings("Kills: " ("text"), w1845) -> (w1846:string)
                    n903 = call <vilib>:"Draw Text at Point.vi"("[user-specified font]"=T14 {"Font Name:"="Arial", "Size"=42, "Strikeout?"=FALSE, "Italic?"=FALSE, "Underline?"=FALSE, "Outline?"=FALSE, "Shadow?"=TRUE, "Bold?"=TRUE}, "text color(black)"=u32 16735530, "desired font(Application)"=T13."User-specified Font", "text"=w1846, "alignment(left, top)"=T15 {"horizontal"=enum."center", "vertical"=enum."center"}, "origin"=cluster{"x":i16, "y":i16} {"x"=810, "y"=270}, "picture"=w1844) -> ("new picture"=w1843:picture)  [unwired: 3 in, 1 out]
                  }
                }
              }
            }
            n904 = local read "Alive number"() -> (w1708:i32)
            n905 = Less Or Equal?(x=w1708, y=1) -> (x <= y?=w1706:bool)
            n906 = case shown="True" w1706 {
              tunnel: [w1784 w1792] -> w1704
              tunnel: w1705 -> [w1784 w1788]
              frame False {
              }
              frame True {
                # "Shade final winner"
                n907 = local read "MO ID"() -> (w1791:i32)
                n908 = local read "Player info"() -> (w1802:T6)
                n909 = Increment(x=w1791) -> (x+1=w1790:i32)
                n910 = for {
                  N: w1790 -> [_]
                  tunnel: w1802 -> [w1807] mode=indexing
                  tunnel: [w1803] -> w1801
                  stop <- w1804 stop-if-true
                  n911 = Unbundle(w1807) -> ("Name"=w1803:string, "Who Kill Me"=w1806:dbl)  [unwired: 3 out]
                  n912 = Equal?(x=w1806, y=-1.0) -> (x = y?=w1804:bool)
                }
                "Final Winner" <- w1801
                n913 = call <vilib>:"Draw Rectangle.vi"("picture"=w1788, "rect"=T11 {"left"=280, "top"=20, "right"=1000, "bottom"=100}, "fill?(F)"=TRUE, "color(black)"=u32 15395562) -> ("new picture"=w1789:picture)  [unwired: 5 in]
                n914 = local read "Final Winner"() -> (w1794:string)
                n915 = Concatenate Strings(w1794, " 取得最終勝利!" ("string")) -> (w1795:string)
                n916 = call <vilib>:"Draw Text at Point.vi"("[user-specified font]"=T14 {"Font Name:"="Arial", "Size"=56, "Strikeout?"=FALSE, "Italic?"=FALSE, "Underline?"=FALSE, "Outline?"=FALSE, "Shadow?"=TRUE, "Bold?"=TRUE}, "text color(black)"=u32 15715328, "desired font(Application)"=T13."User-specified Font", "text"=w1795, "alignment(left, top)"=T15 {"horizontal"=enum."center", "vertical"=enum."center"}, "origin"=cluster{"x":i16, "y":i16} {"x"=640, "y"=60}, "picture"=w1789) -> ("new picture"=w1792:picture)  [unwired: 3 in, 1 out]
              }
            }
            "PlayingScene" <- w1704
            "Frame Number" <- w1746
            "Object number" <- w1747
          }
          n917 = call <vilib>:"Intialize Keyboard.vi"() -> ("device ID"=w869:refnum<k1>)  [unwired: 10 in, 1 out]
          n918 = call <vilib>:"Initialize Mouse.vi"() -> ("device ID"=w868:refnum<k1>)  [unwired: 10 in, 1 out]
          n919 = while {
            tunnel: w872 -> [w960]
            tunnel: w871 -> [w970]
            tunnel: w870 -> [w971]
            tunnel: w869 -> [w976]
            tunnel: w868 -> [w975]
            tunnel: [w973] -> w867
            tunnel: [w972] -> w866
            tunnel: w864 -> [w959]
            stop <- w977 stop-if-true
            # "Shoot command"
            # "Move command"
            n920 = local read "電腦代打模式:\n(Based on Machine Learning)\n(Behavior cloning)\n(Warning: High computing workload)"() -> (w961:bool)
            n921 = case shown="False" w961 {
              tunnel: w976 -> [w1248 w1348]
              tunnel: w975 -> [w1247 w1349]
              tunnel: [w1246 w1349] -> w973
              tunnel: [w1245 w1348] -> w972
              tunnel: [w1205 w1347] -> w969
              tunnel: [w1204 w1347] -> w968
              tunnel: w960 -> [w1187 w1346]
              tunnel: [w1187 w1344] -> w950
              tunnel: w959 -> [_ w1345]
              frame False {
                w1206 = T7 [] ("Moving Entity Position")
                w1212 = 0 ("y")
                w1219 = 0.0
                # "Bullets, shooting, reloading processing"
                # "Host player input detect"
                # "A/D"
                # "W/S"
                n922 = control-ref of="Pane"() -> (w1199:refnum<vi>)
                n923 = control-ref of="This VI"() -> (w1243:refnum<vi>)
                n924 = property class="Pane"(reference=w1199) -> ("Origin"=w1244:T36)  [unwired: 1 in, 2 out]
                n925 = call-poly <vilib>:"Acquire Input Data.vi"("device ID"=w1248) -> ("device ID"=w1245:refnum<k1>, "keys pressed"=w1218:T37)  [unwired: 16 in, 1 out]
                n926 = call-poly <vilib>:"Acquire Input Data.vi"("device ID"=w1247, "key mode"=enum16{"RELATIVE", "ABSOLUTE"}."ABSOLUTE") -> ("device ID"=w1246:refnum<k1>, "axis info"=w1220:T38, "button info"=w1210:T39)  [unwired: 14 in, 1 out]
                n927 = property class="VI"(reference=w1243) -> ("Front Panel.PanelBounds"=w1242:T40)  [unwired: 1 in, 2 out]
                n928 = Unbundle By Name(w1220) -> ("Horizontal"=w1235:i32, "Vertical"=w1233:i32)
                n929 = Unbundle By Name(w1244) -> ("Horizontal"=w1239:i16, "Vertical"=w1238:i16)
                n930 = for {
                  tunnel: w1218 -> [w1321] mode=indexing
                  shift-right: [w1320] -> w1197
                  shift-left: 0 ("y") -> [w1319]
                  shift-right: [w1318] -> w1195
                  shift-left: 0 ("y") -> [w1317]
                  shift-right: [w1316] -> w1209
                  shift-left: FALSE -> [w1315]
                  n931 = case shown="\"0\", Default" w1321 {
                    tunnel: [w1324 w1326 w1330 w1336 w1340 w1343] -> w1320
                    tunnel: w1319 -> [w1324 w1327 w1331 w1336 w1340 w1343]
                    tunnel: [w1323 w1328 w1332 w1334 w1338 w1342] -> w1318
                    tunnel: w1317 -> [w1323 w1328 w1332 w1335 w1339 w1342]
                    tunnel: [w1322 w1325 w1329 w1333 w1337 TRUE] -> w1316
                    tunnel: w1315 -> [w1322 w1325 w1329 w1333 w1337 _]
                    frame "0", Default {
                    }
                    frame "W" {
                      n932 = Decrement(x=w1327) -> (x-1=w1326:i32)
                    }
                    frame "S" {
                      n933 = Increment(x=w1331) -> (x+1=w1330:i32)
                    }
                    frame "A" {
                      n934 = Decrement(x=w1335) -> (x-1=w1334:i32)
                    }
                    frame "D" {
                      n935 = Increment(x=w1339) -> (x+1=w1338:i32)
                    }
                    frame "R" {
                    }
                  }
                }
                n936 = Unbundle By Name(w1242) -> ("Left"=w1237:i16, "Top"=w1236:i16)
                n937 = Subtract(x=w1239, y=w1237) -> (x-y=w1240:i16)
                n938 = Subtract(x=w1238, y=w1236) -> (x-y=w1241:i16)
                n939 = To Long Integer(number=w1241) -> (32bit integer=w1232:i32)
                n940 = To Long Integer(number=w1240) -> (32bit integer=w1234:i32)
                n941 = Add(x=w1233, y=w1232) -> (x+y=w1224:i32)
                n942 = Add(x=w1235, y=w1234) -> (x+y=w1225:i32)
                n943 = Less?(x=w1224, y=0) -> (x < y?=w1229:bool)
                n944 = Divide(x=w1225, y=w1224) -> (x/y=w1231:dbl)
                n945 = Inverse Tangent(1:w1231) -> (0:w1226:dbl)
                n946 = Not Equal?(x=w1197, y=0) -> (x != y?=w1190:bool)
                n947 = Not Equal?(x=w1195, y=0) -> (x != y?=w1191:bool)
                n948 = Add(x=w1226, y=3.141592653589793) -> (x+y=w1227:dbl)
                n949 = Or(x=w1190, y=w1191) -> (x .or. y?=w1192:bool)
                n950 = Equal?(x=w1197, y=w1212) -> (x = y?=w1214:bool)
                n951 = Equal?(x=w1195, y=w1212) -> (x = y?=w1215:bool)
                n952 = Select(t=1.0, s=w1192, f=0.0) -> (s? t:f=w1193:dbl)
                n953 = Select(t=w1227, s=w1229, f=w1226) -> (s? t:f=w1223:dbl)
                n954 = And(x=w1214, y=w1215) -> (x .and. y?=w1213:bool)
                n955 = Unbundle(w1210) -> ("button 1"=w1208:bool)  [unwired: 3 out]
                n956 = Square Root(x=w1193) -> (sqrt(x)=w1202:dbl)
                n957 = Add(x=w1223, y=1.5707963267948966) -> (x+y=w1200:dbl)
                n958 = case shown="False" w1209 {
                  tunnel: w1208 -> [w1265 _]
                  tunnel: [w1267 w1301] -> w1204
                  tunnel: w1206 -> [w1266 w1301]
                  tunnel: w1200 -> [w1255 _]
                  frame False {
                    w1264 = 0 ("index")
                    n959 = local read "Player Bullets"() -> (w1253:i32[])
                    n960 = local read "Player Bullets Reload"() -> (w1257:i32[])
                    n961 = Index Array(array=w1253, index=w1264) -> (element=w1254:i32)
                    n962 = Index Array(array=w1257, index=0) -> (element=w1256:i32)
                    n963 = Greater?(x=w1254, y=w1264) -> (0:w1262:bool)
                    n964 = Equal?(x=w1256, y=0) -> (x = y?=w1259:bool)
                    n965 = And(x=w1265, y=w1262) -> (x .and. y?=w1261:bool)
                    n966 = And(x=w1259, y=w1261) -> (x .and. y?=w1260:bool)
                    n967 = case shown="True" w1260 {
                      tunnel: [w1279 w1299] -> w1267
                      tunnel: w1266 -> [w1279 w1298]
                      tunnel: w1257 -> [w1276 w1291]
                      tunnel: w1256 -> [w1272 _]
                      tunnel: w1255 -> [_ w1294]
                      tunnel: w1254 -> [_ w1292]
                      tunnel: w1253 -> [w1268 w1285]
                      frame False {
                        n968 = Greater?(x=w1272, y=0 ("index")) -> (0:w1275:bool)
                        n969 = Decrement(x=w1272) -> (x-1=w1273:i32)
                        n970 = Select(t=w1273, s=w1275, f=w1272) -> (s? t:f=w1270:i32)
                        n971 = Replace Array Subset(array=w1276, new element=w1270, index=0) -> (w1277:i32[])
                        n972 = Equal?(x=w1270, y=5) -> (x = y?=w1271:bool)
                        n973 = local write "Player Bullets Reload"(w1277) -> ()
                        n974 = case shown="True" w1271 {
                          tunnel: w1268 -> [_ w1280]
                          frame False {
                          }
                          frame True {
                            n975 = Replace Array Subset(array=w1280, new element=30 ("index"), index=0) -> (w1283:i32[])
                            n976 = local write "Player Bullets"(w1283) -> ()
                          }
                        }
                      }
                      frame True {
                        w1296 = 0.0
                        n977 = Decrement(x=w1292) -> (x-1=w1287:i32)
                        n978 = Replace Array Subset(array=w1285, new element=w1287, index=0) -> (w1286:i32[])
                        n979 = Bundle(w1296, w1296, 100.0, w1296, 15.0, w1294) -> (w1297:cluster{dbl, dbl, dbl, dbl, dbl, dbl})  [unwired: 1 in]
                        n980 = local write "Player Bullets"(w1286) -> ()
                        n981 = Build Array (concatenate)(w1298, w1297) -> (w1299:T7)
                        n982 = Replace Array Subset(array=w1291, new element=4 ("new element/subarray"), index=0) -> (w1290:i32[])
                        n983 = local write "Player Bullets Reload"(w1290) -> ()
                      }
                    }
                  }
                  frame True {
                    n984 = local read "Player Bullets Reload"() -> (w1302:i32[])
                    n985 = Index Array(array=w1302, index=0) -> (element=w1300:i32)
                    n986 = Less?(x=w1300, y=5) -> (x < y?=w1303:bool)
                    n987 = case shown="True" w1303 {
                      tunnel: w1302 -> [w1308 w1314]
                      tunnel: w1300 -> [w1307 _]
                      frame False {
                        n988 = Decrement(x=w1307) -> (x-1=w1306:i32)
                        n989 = Replace Array Subset(array=w1308, new element=w1306, index=0 ("new element/subarray")) -> (w1309:i32[])
                        n990 = local write "Player Bullets Reload"(w1309) -> ()
                      }
                      frame True {
                        n991 = Replace Array Subset(array=w1314, new element=120 ("new element/subarray"), index=0 ("new element/subarray")) -> (w1311:i32[])
                        n992 = local write "Player Bullets Reload"(w1311) -> ()
                      }
                    }
                  }
                }
                n993 = case shown="True" w1213 {
                  tunnel: [w1251 0.0 ("Theta")] -> w1211
                  tunnel: w1197 -> [w1250 _]
                  tunnel: w1195 -> [w1249 _]
                  frame False {
                    n994 = call "XY to Theta (2D picture).vi"("y"=w1250, "x"=w1249) -> ("Theta"=w1251:dbl)
                  }
                  frame True {
                  }
                }
                "Theta" <- w1211
                n995 = Multiply(x=w1202, y=4.0) -> (x*y=w1203:dbl)
                "Movement" <- w1203
                n996 = Bundle(w1219, w1219, w1219, w1200, w1203, "Theta"=w1211) -> (w1207:cluster{dbl, dbl, dbl, dbl, dbl, "Theta":dbl})  [unwired: 1 in]
                n997 = Build Array (concatenate)(w1206, w1207) -> (w1205:T4)
              }
              frame True {
                w1347 = T7 [] ("Moving Entity Position")
                n998 = Build Array (concatenate)(w1345, w1346) -> (w1344:refnum<queue>[])
              }
            }
            n999 = Array Size(array=w950) -> (size(s)=w951:i32)
            n1000 = Not Equal To 0?(x=w951) -> (x != 0?=w949:bool)
            n1001 = case shown="True" w949 {
              tunnel: w969 -> [w979 w984]
              tunnel: w968 -> [w978 w983]
              tunnel: [w979 w982] -> w956
              tunnel: [w978 w981] -> w955
              tunnel: w950 -> [_ w980]
              frame False {
              }
              frame True {
                n1002 = for {
                  tunnel: w980 -> [w991] mode=indexing
                  shift-right: [w993] -> w982
                  shift-left: w984 -> [w996]
                  shift-right: [w994] -> w981
                  shift-left: w983 -> [w995]
                  i -> [w986]
                  n1003 = local read "電腦代打模式:\n(Based on Machine Learning)\n(Behavior cloning)\n(Warning: High computing workload)"() -> (w988:bool)
                  n1004 = Increment(x=w986) -> (x+1=w985:i32)
                  n1005 = Select(t=w986, s=w988, f=w985) -> (s? t:f=w987:i32)
                  n1006 = Dequeue Element(queue=w991, timeout in ms (-1)=0) -> (element=w990:cluster{dbl, dbl, dbl, dbl}, timed out?=w989:bool)  [unwired: 1 in, 2 out]
                  n1007 = case shown="False" w989 {
                    tunnel: w996 -> [w1009 w1097]
                    tunnel: w995 -> [w1004 w1095]
                    tunnel: [w1005 w1095] -> w994
                    tunnel: [w1008 w1096] -> w993
                    tunnel: w987 -> [w1001 w1093]
                    tunnel: w990 -> [w1012 _]
                    frame False {
                      w1011 = 0.0
                      # "Input transformation"
                      # "Bullets, shooting, reloading processing"
                      n1008 = local read "Player Bullets"() -> (w1000:i32[])
                      n1009 = Index Array(array=w1000, index=w1001) -> (element=w999:i32)
                      n1010 = Not Equal?(x=w999, y=0) -> (x != y?=w998:bool)
                      n1011 = Unbundle(w1012) -> (w1006:dbl, w1007:dbl, w1003:dbl, w997:dbl)
                      n1012 = case shown="True" w998 {
                        tunnel: [w1019 w1061] -> w1005
                        tunnel: w1004 -> [w1019 w1060]
                        tunnel: w1001 -> [w1016 w1049]
                        tunnel: w1003 -> [_ w1059]
                        tunnel: w1000 -> [w1013 w1055]
                        tunnel: w999 -> [_ _]
                        tunnel: w997 -> [_ w1050]
                        frame False {
                          n1013 = local read "Player Bullets Reload"() -> (w1017:i32[])
                          n1014 = Index Array(array=w1017, index=w1016) -> (element=w1015:i32)
                          n1015 = Less?(x=w1015, y=5) -> (x < y?=w1014:bool)
                          n1016 = case shown="False" w1014 {
                            tunnel: w1017 -> [w1025 w1046]
                            tunnel: w1016 -> [w1024 w1045]
                            tunnel: w1015 -> [w1023 _]
                            tunnel: w1013 -> [w1020 _]
                            frame False {
                              n1017 = Not Equal?(x=w1023, y=5) -> (x != y?=w1021:bool)
                              n1018 = case shown="False" w1021 {
                                tunnel: w1025 -> [w1033 w1044]
                                tunnel: w1024 -> [w1032 w1034]
                                tunnel: w1023 -> [w1026 w1038]
                                tunnel: w1020 -> [_ w1035]
                                frame True {
                                n1019 = Greater?(x=w1026, y=0 ("index")) -> (0:w1030:bool)
                                n1020 = Decrement(x=w1026) -> (x-1=w1028:i32)
                                n1021 = Select(t=w1028, s=w1030, f=w1026) -> (s? t:f=w1027:i32)
                                n1022 = Replace Array Subset(array=w1033, new element=w1027, index=w1032) -> (w1031:i32[])
                                n1023 = local write "Player Bullets Reload"(w1031) -> ()
                                }
                                frame False {
                                n1024 = Greater?(x=w1038, y=0 ("index")) -> (0:w1042:bool)
                                n1025 = Decrement(x=w1038) -> (x-1=w1040:i32)
                                n1026 = Select(t=w1040, s=w1042, f=w1038) -> (s? t:f=w1039:i32)
                                n1027 = Replace Array Subset(array=w1044, new element=w1039, index=w1034) -> (w1043:i32[])
                                n1028 = local write "Player Bullets Reload"(w1043) -> ()
                                n1029 = Replace Array Subset(array=w1035, new element=30 ("index"), index=w1034) -> (w1036:i32[])
                                n1030 = local write "Player Bullets"(w1036) -> ()
                                }
                              }
                            }
                            frame True {
                              n1031 = Replace Array Subset(array=w1046, new element=120 ("new element/subarray"), index=w1045) -> (w1047:i32[])
                              n1032 = local write "Player Bullets Reload"(w1047) -> ()
                            }
                          }
                        }
                        frame True {
                          n1033 = local read "Player Bullets Reload"() -> (w1058:i32[])
                          n1034 = Index Array(array=w1055, index=w1049) -> (element=w1057:i32)
                          n1035 = Index Array(array=w1058, index=w1049) -> (element=w1056:i32)
                          n1036 = Equal?(x=w1050, y=1.0) -> (x = y?=w1052:bool)
                          n1037 = Equal?(x=w1056, y=0) -> (x = y?=w1062:bool)
                          n1038 = Greater?(x=w1057, y=0 ("index")) -> (0:w1064:bool)
                          n1039 = And(x=w1062, y=w1064) -> (x .and. y?=w1054:bool)
                          n1040 = And(x=w1054, y=w1052) -> (x .and. y?=w1053:bool)
                          n1041 = case shown="True" w1053 {
                            tunnel: [w1074 w1087] -> w1061
                            tunnel: w1060 -> [w1074 w1088]
                            tunnel: w1059 -> [_ w1083]
                            tunnel: w1049 -> [w1066 w1075]
                            tunnel: w1058 -> [w1068 w1080]
                            tunnel: w1055 -> [_ w1077]
                            tunnel: w1057 -> [_ w1076]
                            tunnel: w1056 -> [w1069 _]
                            frame False {
                              n1042 = Greater?(x=w1069, y=0 ("index")) -> (0:w1073:bool)
                              n1043 = Decrement(x=w1069) -> (x-1=w1071:i32)
                              n1044 = Select(t=w1071, s=w1073, f=w1069) -> (s? t:f=w1070:i32)
                              n1045 = Replace Array Subset(array=w1068, new element=w1070, index=w1066) -> (w1067:i32[])
                              n1046 = local write "Player Bullets Reload"(w1067) -> ()
                            }
                            frame True {
                              w1090 = 0.0
                              n1047 = Decrement(x=w1076) -> (x-1=w1079:i32)
                              n1048 = Add(x=w1075, y=100.0) -> (x+y=w1085:dbl)
                              n1049 = Replace Array Subset(array=w1077, new element=w1079, index=w1075) -> (w1078:i32[])
                              n1050 = Replace Array Subset(array=w1080, new element=4 ("new element/subarray"), index=w1075) -> (w1081:i32[])
                              n1051 = Bundle(w1090, w1090, w1085, w1090, 15.0, w1083) -> (w1086:cluster{dbl, dbl, dbl, dbl, dbl, dbl})  [unwired: 1 in]
                              n1052 = local write "Player Bullets"(w1078) -> ()
                              n1053 = Build Array (concatenate)(w1088, w1086) -> (w1087:T7)
                              n1054 = local write "Player Bullets Reload"(w1081) -> ()
                            }
                          }
                        }
                      }
                      n1055 = Bundle(w1011, w1011, w1001, w1003, w1006, w1007) -> (w1010:cluster{dbl, dbl, i32, dbl, dbl, dbl})  [unwired: 1 in]
                      n1056 = Build Array (concatenate)(w1009, w1010) -> (w1008:T7)
                    }
                    frame True {
                      w1092 = 0.0
                      # "-5000 means  no input"
                      n1057 = Bundle(w1092, w1092, w1093, -5000.0, w1092, w1092) -> (w1094:cluster{dbl, dbl, i32, dbl, dbl, dbl})  [unwired: 1 in]
                      n1058 = Build Array (concatenate)(w1097, w1094) -> (w1096:T7)
                    }
                  }
                }
              }
            }
            n1059 = Wait (ms)(milliseconds to wait=u32 16) -> ()  [unwired: 1 out]
            n1060 = call <vilib>:"High Resolution Relative Seconds.vi"() -> ("relative seconds"=w964:dbl)
            n1061 = feedback #4(u32 0 ("millisecond timer value")) -> (w965:dbl)
            n1062 = feedback-in #4(w964) -> ()
            n1063 = Subtract(x=w964, y=w965) -> (x-y=w967:dbl)
            n1064 = Divide(x=1.0, y=w967) -> (x/y=→"Input detect frequency (Hz)":dbl)
            n1065 = local read "STOP (會卡住)"() -> (w977:bool)
            n1066 = local read "NetPlayer Commend"() -> (w952:T1)
            n1067 = Array Size(array=w952) -> (size(s)=w958:i32)
            n1068 = Not Equal To 0?(x=w958) -> (x != 0?=w957:bool)
            n1069 = case shown="True" w957 {
              tunnel: w956 -> [w1099 w1104]
              tunnel: w955 -> [w1098 w1102]
              tunnel: [w1099 w1103] -> w954
              tunnel: [w1098 w1101] -> w953
              tunnel: w952 -> [_ w1100]
              frame False {
              }
              frame True {
                n1070 = for {
                  shift-right: [w1115] -> w1103
                  shift-left: w1104 -> [w1125]
                  shift-right: [w1108] -> w1101
                  shift-left: w1102 -> [w1109]
                  tunnel: w1100 -> [w1123] mode=indexing
                  i -> [w1119]
                  w1124 = 0.0
                  # "Read command from NetPlayers"
                  n1071 = local read "初級電腦玩家人數:"() -> (w1117:i32)
                  n1072 = local read "普通電腦玩家人數:"() -> (w1116:i32)
                  n1073 = Unbundle(w1123) -> ("Vector scalar"=w1122:sgl, "Vector theta"=w1121:sgl, "Mouse theta"=w1105:sgl, "Mouse Shoot"=w1110:sgl, "Reload R"=w1114:sgl)
                  n1074 = Increment(x=w1119) -> (x+1=w1118:i32)
                  n1075 = Compound Arithmetic op=ADD(w1117, w1116, w1118) -> (w1107:i32)
                  n1076 = Bundle(w1124, w1124, w1107, "Mouse theta"=w1105, "Vector scalar"=w1122, "Vector theta"=w1121) -> (w1120:T41)  [unwired: 1 in]
                  n1077 = Build Array (concatenate)(w1125, w1120) -> (w1115:T7)
                  n1078 = Equal?(x=sgl 1.0, y=w1114) -> (x = y?=w1112:bool)
                  n1079 = Equal?(x=sgl 1.0, y=w1110) -> (x = y?=w1106:bool)
                  n1080 = case shown="False" w1112 {
                    tunnel: w1109 -> [w1139 w1177]
                    tunnel: [w1138 w1177] -> w1108
                    tunnel: w1107 -> [w1130 w1173]
                    tunnel: w1106 -> [w1133 _]
                    tunnel: w1105 -> [w1126 _]
                    frame False {
                      n1081 = local read "Player Bullets Reload"() -> (w1129:i32[])
                      n1082 = local read "Player Bullets"() -> (w1128:i32[])
                      n1083 = Index Array(array=w1128, index=w1130) -> (element=w1127:i32)
                      n1084 = Greater Than 0?(x=w1127) -> (x > 0?=w1134:bool)
                      n1085 = Index Array(array=w1129, index=w1130) -> (element=w1131:i32)
                      n1086 = Equal?(x=w1131, y=0) -> (x = y?=w1135:bool)
                      n1087 = And(x=w1133, y=w1134) -> (x .and. y?=w1137:bool)
                      n1088 = And(x=w1135, y=w1137) -> (x .and. y?=w1132:bool)
                      n1089 = case shown="False" w1132 {
                        tunnel: w1139 -> [w1151 w1169]
                        tunnel: [w1151 w1168] -> w1138
                        tunnel: w1131 -> [w1147 _]
                        tunnel: w1130 -> [w1140 w1157]
                        tunnel: w1129 -> [w1146 w1166]
                        tunnel: w1128 -> [w1141 w1163]
                        tunnel: w1127 -> [_ w1162]
                        tunnel: w1126 -> [_ w1159]
                        frame False {
                          n1090 = Greater?(x=w1147, y=0 ("index")) -> (0:w1150:bool)
                          n1091 = Decrement(x=w1147) -> (x-1=w1148:i32)
                          n1092 = Select(t=w1148, s=w1150, f=w1147) -> (s? t:f=w1143:i32)
                          n1093 = Replace Array Subset(array=w1146, new element=w1143, index=w1140) -> (w1145:i32[])
                          n1094 = Equal?(x=w1143, y=5) -> (x = y?=w1142:bool)
                          n1095 = local write "Player Bullets Reload"(w1145) -> ()
                          n1096 = case shown="True" w1142 {
                            tunnel: w1141 -> [_ w1155]
                            tunnel: w1140 -> [_ w1154]
                            frame False {
                            }
                            frame True {
                              n1097 = Replace Array Subset(array=w1155, new element=30 ("new element/subarray"), index=w1154) -> (w1152:i32[])
                              n1098 = local write "Player Bullets"(w1152) -> ()
                            }
                          }
                        }
                        frame True {
                          w1171 = 0.0
                          n1099 = Decrement(x=w1162) -> (x-1=w1161:i32)
                          n1100 = Add(x=100, y=w1157) -> (x+y=w1158:i32)
                          n1101 = Replace Array Subset(array=w1163, new element=w1161, index=w1157) -> (w1160:i32[])
                          n1102 = Bundle(w1171, w1171, w1158, w1171, 15.0, "Mouse theta"=w1159) -> (w1164:T42)  [unwired: 1 in]
                          n1103 = local write "Player Bullets"(w1160) -> ()
                          n1104 = Build Array (concatenate)(w1169, w1164) -> (w1168:T7)
                          n1105 = Replace Array Subset(array=w1166, new element=4 ("new element/subarray"), index=w1157) -> (w1167:i32[])
                          n1106 = local write "Player Bullets Reload"(w1167) -> ()
                        }
                      }
                    }
                    frame True {
                      n1107 = local read "Player Bullets Reload"() -> (w1174:i32[])
                      n1108 = Index Array(array=w1174, index=w1173) -> (element=w1172:i32)
                      n1109 = Less?(x=w1172, y=5) -> (x < y?=w1175:bool)
                      n1110 = case shown="False" w1175 {
                        tunnel: w1174 -> [w1179 w1185]
                        tunnel: w1173 -> [w1181 w1183]
                        tunnel: w1172 -> [w1180 _]
                        frame False {
                          n1111 = Decrement(x=w1180) -> (x-1=w1182:i32)
                          n1112 = Replace Array Subset(array=w1179, new element=w1182, index=w1181) -> (w1178:i32[])
                          n1113 = local write "Player Bullets Reload"(w1178) -> ()
                        }
                        frame True {
                          n1114 = Replace Array Subset(array=w1185, new element=120 ("new element/subarray"), index=w1183) -> (w1184:i32[])
                          n1115 = local write "Player Bullets Reload"(w1184) -> ()
                        }
                      }
                    }
                  }
                }
              }
            }
            "Sent command" <- w954
            n1116 = Lossy Enqueue Element(queue=w971, element=w954) -> ()  [unwired: 1 in, 4 out]
            n1117 = Lossy Enqueue Element(queue=w970, element=w953) -> ()  [unwired: 1 in, 4 out]
          }
          n1118 = call-poly <vilib>:"Close Input Device.vi"("device ID"=w866) -> ()  [unwired: 9 in, 1 out]
          n1119 = call-poly <vilib>:"Close Input Device.vi"("device ID"=w867) -> ()  [unwired: 9 in, 1 out]
          n1120 = local read "初級電腦玩家人數:"() -> (w853:i32)
          n1121 = local read "普通電腦玩家人數:"() -> (w852:i32)
          n1122 = local read "選擇網路介面:"() -> (w863:string)
          n1123 = String To IP(1:w863) -> (0:w862:u32)
          n1124 = Add(x=w853, y=w852) -> (x+y=w851:i32)
          n1125 = UDP Open(7:w862, 11:u16 52023 ("port")) -> (port=w860:refnum<k16>)  [unwired: 3 in, 2 out]
          n1126 = Increment(x=w851) -> (x+1=w850:i32)
          n1127 = while {
            tunnel: w860 -> [w893]
            tunnel: [w899] -> w859
            tunnel: w855 -> [w897]
            tunnel: w854 -> [w890]
            tunnel: w850 -> [w889]
            stop <- w900 stop-if-true
            # "Read input commands from NetPlayer (Get one each time)"
            n1128 = Dequeue Element(queue=w897, timeout in ms (-1)=0) -> (element=w894:T8, timed out?=w895:bool)  [unwired: 1 in, 2 out]
            n1129 = UDP Read(connection ID=w893, timeout ms (25000)=1) -> (data out=w898:string, error out=w891:errorcluster, 3:w899:refnum<k16>)  [unwired: 2 in, 2 out]
            n1130 = case shown="False" w895 {
              tunnel: w894 -> [w923 _]
              tunnel: w893 -> [w925 _]
              tunnel: w890 -> [w919 _]
              frame False {
                # "Send scene data to NetPlayers"
                n1131 = local read "Final Winner"() -> (w920:string)
                n1132 = local read "Player info"() -> (w921:T6)
                n1133 = local read "Alive number"() -> (w922:i32)
                n1134 = To Single Precision Float(number=w923) -> (single precision float=w918:T43)
                n1135 = local read "NetPlayer"() -> (w924:cluster{"Name":string, "IP Address":u32}[])
                n1136 = for {
                  tunnel: w925 -> [w948]
                  tunnel: w924 -> [w946] mode=indexing
                  tunnel: w918 -> [w943]
                  tunnel: w920 -> [w942]
                  tunnel: w921 -> [w941]
                  tunnel: w922 -> [w940]
                  tunnel: w919 -> [w933]
                  i -> [w937]
                  n1137 = local read "初級電腦玩家人數:"() -> (w935:i32)
                  n1138 = local read "普通電腦玩家人數:"() -> (w934:i32)
                  n1139 = local read "Player Bullets Reload"() -> (w939:i32[])
                  n1140 = Unbundle(w946) -> ("IP Address"=w945:u32)  [unwired: 1 out]
                  n1141 = Increment(x=w937) -> (x+1=w936:i32)
                  n1142 = Compound Arithmetic op=ADD(w936, w935, w934) -> (w927:i32)
                  n1143 = Index Array(array=w939, index=w927) -> (element=w938:i32)
                  n1144 = local read "Player Bullets"() -> (w928:i32[])
                  n1145 = Index Array(array=w928, index=w927) -> (element=w926:i32)
                  n1146 = Bundle(w943, "Final Winner"=w942, "Player info"=w941, "Alive number"=w940, w938, w933, w926) -> (w944:T44)  [unwired: 1 in]
                  n1147 = Flatten To String(anything=w944) -> (data string=w932:string, error out=w929:errorcluster)  [unwired: 3 in, 1 out]
                  n1148 = Unbundle(w929) -> ()  [unwired: 3 out]
                  n1149 = String Length(string=w932) -> (length=→"Data length":i32)
                  n1150 = UDP Write(address=w945, port or service name=u16 52023, connection ID=w948, data in=w932) -> (error out=w930:errorcluster)  [unwired: 2 in, 1 out]
                  n1151 = Unbundle(w930) -> ()  [unwired: 3 out]
                }
              }
              frame True {
              }
            }
            n1152 = case shown="No Error" w891 {
              tunnel: w898 -> [w905 _]
              tunnel: w889 -> [w901 _]
              frame No Error {
                n1153 = Unflatten From String(type=T19 {"Vector scalar"=0.0, "Vector theta"=0.0, "Mouse theta"=0.0, "Mouse Shoot"=0.0, "Reload R"=0.0, "Reload R 2"=0.0} ("NetPlayer Commend"), binary string=w905) -> (value=w903:T19, error out=w902:errorcluster)  [unwired: 3 in, 1 out]
                n1154 = case shown="No Error" w902 {
                  tunnel: w903 -> [w917 _]
                  tunnel: w901 -> [w906 _]
                  frame No Error {
                    n1155 = local read "NetPlayer Commend"() -> (w916:T1)
                    n1156 = Unbundle(w917) -> ("Vector scalar"=w910:sgl, "Vector theta"=w911:sgl, "Mouse theta"=w912:sgl, "Mouse Shoot"=w913:sgl, "Reload R"=w914:sgl, "Reload R 2"=w907:sgl)
                    n1157 = Subtract(x=w907, y=w906) -> (x-y=w908:sgl)
                    n1158 = Bundle("Vector scalar"=w910, "Vector theta"=w911, "Mouse theta"=w912, "Mouse Shoot"=w913, "Reload R"=w914) -> (w915:T45)  [unwired: 1 in]
                    n1159 = Replace Array Subset(array=w916, new element=w915, index=w908) -> (w909:T1)
                    n1160 = local write "NetPlayer Commend"(w909) -> ()
                  }
                  frame Error {
                  }
                }
              }
              frame Error {
              }
            }
            n1161 = local read "STOP (會卡住)"() -> (w900:bool)
          }
          n1162 = UDP Close(connection ID=w859) -> ()  [unwired: 1 in, 2 out]
        }
      }
    }
    frame True {
      # "Read scene data from Network"
      # "Input Dectection Model\n(Network version)"
      # "Shading Model"
      # "If current user is a NetPlayer who builds connection to host"
      n1163 = local read "選擇網路介面:"() -> (w2259:string)
      n1164 = local read "Host IP: (Local Network)"() -> (w2257:string)
      n1165 = String To IP(1:w2259) -> (0:w2261:u32)
      n1166 = UDP Open(7:w2261, 11:u16 52023 ("port")) -> (port=w2255:refnum<k16>)  [unwired: 3 in, 2 out]
      n1167 = To Single Precision Float(number=T8 [] ("Map Entity Object Position")) -> (single precision float=w2249:T43)
      n1168 = String To IP(1:w2257) -> (0:w2256:u32)
      n1169 = Obtain Queue(max queue size (-1, unlimited)=3, name (unnamed)="Shading Model", element data type=w2249) -> (queue out=w2251:refnum<queue>)  [unwired: 2 in, 2 out]
      n1170 = call <vilib>:"Intialize Keyboard.vi"() -> ("device ID"=w2264:refnum<k1>)  [unwired: 10 in, 1 out]
      n1171 = call <vilib>:"Initialize Mouse.vi"() -> ("device ID"=w2265:refnum<k1>)  [unwired: 10 in, 1 out]
      n1172 = while {
        tunnel: w2255 -> [w2811]
        tunnel: [w2808] -> w2258
        tunnel: w2256 -> [w2807]
        tunnel: w2265 -> [w2855]
        tunnel: [w2829] -> w2263
        tunnel: w2264 -> [w2832]
        tunnel: [w2828] -> w2262
        stop <- w2827 stop-if-true
        w2846 = 0 ("y")
        # "A/D"
        # "W/S"
        n1173 = control-ref of="Pane"() -> (w2852:refnum<vi>)
        n1174 = call-poly <vilib>:"Acquire Input Data.vi"("device ID"=w2832) -> ("device ID"=w2828:refnum<k1>, "keys pressed"=w2831:T37)  [unwired: 16 in, 1 out]
        n1175 = Wait (ms)(milliseconds to wait=u32 16) -> ()  [unwired: 1 out]
        n1176 = control-ref of="This VI"() -> (w2877:refnum<vi>)
        n1177 = property class="Pane"(reference=w2852) -> ("Origin"=w2878:T36)  [unwired: 1 in, 2 out]
        n1178 = call-poly <vilib>:"Acquire Input Data.vi"("device ID"=w2855, "key mode"=enum16{"RELATIVE", "ABSOLUTE"}."ABSOLUTE") -> ("device ID"=w2829:refnum<k1>, "axis info"=w2854:T38, "button info"=w2830:T39)  [unwired: 14 in, 1 out]
        n1179 = for {
          tunnel: w2831 -> [w2889] mode=indexing
          shift-right: [w2888] -> w2842
          shift-left: 0 ("y") -> [w2887]
          shift-right: [w2886] -> w2840
          shift-left: 0 ("y") -> [w2885]
          shift-right: [w2884] -> w2824
          shift-left: FALSE -> [w2883]
          n1180 = case shown="\"0\", Default" w2889 {
            tunnel: [w2892 w2894 w2898 w2904 w2908 w2911] -> w2888
            tunnel: w2887 -> [w2892 w2895 w2899 w2904 w2908 w2911]
            tunnel: [w2891 w2896 w2900 w2902 w2906 w2910] -> w2886
            tunnel: w2885 -> [w2891 w2896 w2900 w2903 w2907 w2910]
            tunnel: [w2890 w2893 w2897 w2901 w2905 TRUE] -> w2884
            tunnel: w2883 -> [w2890 w2893 w2897 w2901 w2905 _]
            frame "0", Default {
            }
            frame "W" {
              n1181 = Decrement(x=w2895) -> (x-1=w2894:i32)
            }
            frame "S" {
              n1182 = Increment(x=w2899) -> (x+1=w2898:i32)
            }
            frame "A" {
              n1183 = Decrement(x=w2903) -> (x-1=w2902:i32)
            }
            frame "D" {
              n1184 = Increment(x=w2907) -> (x+1=w2906:i32)
            }
            frame "R" {
            }
          }
        }
        n1185 = property class="VI"(reference=w2877) -> ("Front Panel.PanelBounds"=w2876:T40)  [unwired: 1 in, 2 out]
        n1186 = Unbundle By Name(w2854) -> ("Horizontal"=w2869:i32, "Vertical"=w2867:i32)
        n1187 = Unbundle By Name(w2878) -> ("Horizontal"=w2873:i16, "Vertical"=w2872:i16)
        n1188 = Unbundle By Name(w2876) -> ("Left"=w2871:i16, "Top"=w2870:i16)
        n1189 = Subtract(x=w2873, y=w2871) -> (x-y=w2874:i16)
        n1190 = Subtract(x=w2872, y=w2870) -> (x-y=w2875:i16)
        n1191 = To Long Integer(number=w2875) -> (32bit integer=w2866:i32)
        n1192 = To Long Integer(number=w2874) -> (32bit integer=w2868:i32)
        n1193 = Add(x=w2867, y=w2866) -> (x+y=w2858:i32)
        n1194 = Add(x=w2869, y=w2868) -> (x+y=w2859:i32)
        n1195 = Less?(x=w2858, y=0) -> (x < y?=w2863:bool)
        n1196 = Divide(x=w2859, y=w2858) -> (x/y=w2865:dbl)
        n1197 = Not Equal?(x=w2842, y=0) -> (x != y?=w2835:bool)
        n1198 = Not Equal?(x=w2840, y=0) -> (x != y?=w2836:bool)
        n1199 = Unbundle(w2830) -> ("button 1"=w2819:bool)  [unwired: 3 out]
        n1200 = Inverse Tangent(1:w2865) -> (0:w2860:dbl)
        n1201 = Or(x=w2835, y=w2836) -> (x .or. y?=w2837:bool)
        n1202 = Equal?(x=w2842, y=w2846) -> (x = y?=w2848:bool)
        n1203 = Equal?(x=w2840, y=w2846) -> (x = y?=w2849:bool)
        n1204 = Select(t=1.0, s=w2837, f=0.0) -> (s? t:f=w2838:dbl)
        n1205 = Add(x=w2860, y=3.141592653589793) -> (x+y=w2861:dbl)
        n1206 = And(x=w2848, y=w2849) -> (x .and. y?=w2847:bool)
        n1207 = Square Root(x=w2838) -> (sqrt(x)=w2845:dbl)
        n1208 = Select(t=w2861, s=w2863, f=w2860) -> (s? t:f=w2857:dbl)
        n1209 = case shown="False" w2847 {
          tunnel: [w2881 0.0 ("Theta")] -> w2814
          tunnel: w2842 -> [w2880 _]
          tunnel: w2840 -> [w2879 _]
          frame False {
            n1210 = call "XY to Theta (2D picture).vi"("y"=w2880, "x"=w2879) -> ("Theta"=w2881:dbl)
          }
          frame True {
          }
        }
        n1211 = Multiply(x=w2845, y=4.0) -> (x*y=w2815:dbl)
        n1212 = Add(x=w2857, y=1.5707963267948966) -> (x+y=w2816:dbl)
        n1213 = local write "Movement"(w2815) -> ()
        n1214 = local write "Theta"(w2816) -> ()
        n1215 = local read "My NetPlayer number"() -> (w2822:i32)
        n1216 = Select(t=1.0, s=w2819, f=0.0) -> (s? t:f=w2817:dbl)
        n1217 = Select(t=1.0, s=w2824, f=0.0) -> (s? t:f=w2818:dbl)
        n1218 = Bundle(w2815, "Theta"=w2814, w2816, "f"=w2817, "f"=w2818, "My NetPlayer number"=w2822) -> (w2813:T46)  [unwired: 1 in]
        n1219 = To Single Precision Float(number=w2813) -> (single precision float=w2812:T47)
        n1220 = Flatten To String(anything=w2812) -> (data string=w2810:string)  [unwired: 3 in, 2 out]
        n1221 = UDP Write(address=w2807, port or service name=u16 52023, connection ID=w2811, data in=w2810) -> (3:w2808:refnum<k16>)  [unwired: 2 in, 1 out]
        n1222 = local read "STOP (會卡住)"() -> (w2827:bool)
      }
      n1223 = while {
        tunnel: w2255 -> [w2778]
        tunnel: w2251 -> [w2775]
        stop <- w2779 stop-if-true
        n1224 = UDP Read(connection ID=w2778, max size (548)=30000) -> (data out=w2776:string, error out=w2774:errorcluster)  [unwired: 2 in, 3 out]
        n1225 = case shown="No Error" w2774 {
          tunnel: w2776 -> [w2792 _]
          tunnel: w2775 -> [w2786 _]
          frame No Error {
            n1226 = To Single Precision Float(number=T8 [] ("Map Entity Object Position")) -> (single precision float=w2783:T43)
            n1227 = Bundle(w2783, "Final Winner"="", "Player info"=T6 [], "Alive number"=0, "element"=0, "element"=0, "element"=0) -> (w2788:T48)  [unwired: 1 in]
            n1228 = Unflatten From String(type=w2788, binary string=w2792) -> (value=w2787:T48, error out=w2782:errorcluster)  [unwired: 3 in, 1 out]
            n1229 = case shown="No Error" w2782 {
              tunnel: w2787 -> [w2806 _]
              tunnel: w2786 -> [w2799 _]
              frame No Error {
                n1230 = local read "My NetPlayer number"() -> (w2796:i32)
                n1231 = local read "Player Bullets Reload"() -> (w2804:i32[])
                n1232 = Unbundle(w2806) -> (w2798:T43, "Final Winner"=w2800:string, "Player info"=w2801:T6, "Alive number"=w2805:i32, "element"=w2802:i32, "element"=w2797:i32, "element"=w2795:i32)
                n1233 = local read "Player Bullets"() -> (w2793:i32[])
                n1234 = Replace Array Subset(array=w2804, new element=w2802, index=w2796) -> (w2803:i32[])
                n1235 = local write "Alive number"(w2805) -> ()
                n1236 = local write "Object number"(w2797) -> ()
                n1237 = Replace Array Subset(array=w2793, new element=w2795, index=w2796) -> (w2794:i32[])
                n1238 = local write "Player Bullets Reload"(w2803) -> ()
                n1239 = local write "Final Winner"(w2800) -> ()
                n1240 = local write "Player info"(w2801) -> ()
                n1241 = local write "Player Bullets"(w2794) -> ()
                n1242 = Lossy Enqueue Element(queue=w2799, element=w2798) -> ()  [unwired: 1 in, 4 out]
              }
              frame Error {
              }
            }
          }
          frame Error {
          }
        }
        n1243 = local read "STOP (會卡住)"() -> (w2779:bool)
      }
      n1244 = call-poly <vilib>:"Close Input Device.vi"("device ID"=w2262) -> ()  [unwired: 9 in, 1 out]
      n1245 = call-poly <vilib>:"Close Input Device.vi"("device ID"=w2263) -> ()  [unwired: 9 in, 1 out]
      n1246 = UDP Close(connection ID=w2258) -> ()  [unwired: 1 in, 2 out]
      n1247 = local read "地圖:"() -> (w2240:string)
      n1248 = Equal?(x=w2240, y="Map 2") -> (x = y?=w2242:bool)
      n1249 = call <vilib>:"RGB to Color.vi"("B"=u8 17, "G"=u8 149, "R"=u8 227) -> ("Color"=w2244:u32)
      n1250 = local read "MO ID"() -> (w2252:i32)
      n1251 = Select(t=w2244, s=w2242, f=u32 13828024 ("color(black)")) -> (s? t:f=w2241:u32)
      n1252 = while {
        tunnel: w2251 -> [w2328]
        tunnel: w2252 -> [w2283]
        tunnel: w2241 -> [w2266]
        i -> [w2272]
        stop <- w2327 stop-if-true
        # "This part is as same as host part, so I'll not interpret again."
        # "Shade Other Objects"
        # "Shade bullet first!"
        # "Refresh Speed limit"
        n1253 = local read "My NetPlayer number"() -> (w2268:i32)
        n1254 = local read "Object number"() -> (w2269:i32)
        n1255 = local write "Frame Number"(w2272) -> ()
        n1256 = call <vilib>:"Draw Rectangle.vi"("picture"=picture data[5B], "rect"=T11 {"left"=0, "top"=0, "right"=1280, "bottom"=720}, "fill?(F)"=TRUE, "color(black)"=w2266) -> ("new picture"=w2314:picture)  [unwired: 5 in]
        n1257 = Dequeue Element(queue=w2328) -> (element=w2273:T43)  [unwired: 2 in, 3 out]
        n1258 = Array Size(array=w2273) -> (size(s)=w2317:i32)
        n1259 = Index Array(array=w2273, index=w2268) -> (element=w2267:T49)
        n1260 = Wait (ms)(milliseconds to wait=u32 16) -> ()  [unwired: 1 out]
        n1261 = Subtract(x=w2317, y=w2269) -> (x-y=w2312:i32)
        n1262 = Greater Or Equal?(x=w2312, y=1) -> (x >= y?=w2316:bool)
        n1263 = case shown="True" w2316 {
          tunnel: w2314 -> [w2450 w2456]
          tunnel: w2267 -> [_ w2455]
          tunnel: [w2450 w2454] -> w2313
          tunnel: w2312 -> [_ w2453]
          tunnel: w2273 -> [_ w2452]
          tunnel: w2269 -> [_ w2451]
          frame False {
          }
          frame True {
            n1264 = for {
              N: w2453 -> [_]
              shift-right: [w2461] -> w2454
              shift-left: w2456 -> [w2460]
              tunnel: w2455 -> [w2477]
              tunnel: w2452 -> [w2466]
              tunnel: w2451 -> [w2464]
              i -> [w2457]
              n1265 = Add(x=w2464, y=w2457) -> (x+y=w2465:i32)
              n1266 = Index Array(array=w2466, index=w2465) -> (element=w2467:T49)
              n1267 = Unbundle By Name(w2477) -> ("X"=w2470:sgl, "Y"=w2471:sgl)
              n1268 = Unbundle By Name(w2467) -> ("X"=w2463:sgl, "Y"=w2462:sgl)
              n1269 = Subtract(x=w2462, y=w2471) -> (x-y=w2458:sgl)
              n1270 = Subtract(x=w2463, y=w2470) -> (x-y=w2459:sgl)
              n1271 = Absolute Value(x=w2458) -> (abs(x)=w2473:sgl)
              n1272 = Absolute Value(x=w2459) -> (abs(x)=w2472:sgl)
              n1273 = Less?(x=w2472, y=660.0) -> (x < y?=w2468:bool)
              n1274 = Less?(x=w2473, y=380.0) -> (x < y?=w2469:bool)
              n1275 = And(x=w2468, y=w2469) -> (x .and. y?=w2475:bool)
              n1276 = case shown="True" w2475 {
                tunnel: [w2478 w2481] -> w2461
                tunnel: w2460 -> [w2478 w2482]
                tunnel: w2459 -> [_ w2488]
                tunnel: w2458 -> [_ w2487]
                frame False {
                }
                frame True {
                  n1277 = Add(x=w2488, y=640.0) -> (x+y=w2485:dbl)
                  n1278 = Add(x=w2487, y=360.0) -> (x+y=w2486:dbl)
                  n1279 = Bundle(w2485, w2486) -> (w2484:cluster{dbl, dbl})  [unwired: 1 in]
                  n1280 = call <vilib>:"Draw Circle by Radius.vi"("color(black)"=u32 2492672, "fill?(F)"=TRUE, "pixel center"=w2484, "radius"=i16 5, "picture"=w2482) -> ("new picture"=w2481:picture)  [unwired: 6 in]
                }
              }
            }
          }
        }
        n1281 = local write "MainPlayer"(w2267) -> ()
        n1282 = for {
          N: w2269 -> [_]
          tunnel: w2283 -> [w2523]
          tunnel: w2273 -> [w2520]
          tunnel: w2267 -> [w2517]
          shift-right: [w2504] -> w2311
          shift-left: w2313 -> [w2505]
          i -> [w2519]
          n1283 = Index Array(array=w2520, index=w2519) -> (element=w2518:T49)
          n1284 = Greater Or Equal?(x=w2519, y=20) -> (x >= y?=w2526:bool)
          n1285 = Unbundle(w2517) -> ("X"=w2515:sgl, "Y"=w2513:sgl, "HP"=w2491:sgl)  [unwired: 8 out]
          n1286 = Less Or Equal?(x=w2519, y=w2523) -> (x <= y?=w2525:bool)
          n1287 = Unbundle(w2518) -> ("X"=w2516:sgl, "Y"=w2514:sgl, "Object type"=w2503:sgl, "Radius"=w2497:sgl, "Width"=w2493:sgl, "Height"=w2492:sgl, "Theta"=w2498:sgl, "HP"=w2499:sgl, "R"=w2496:sgl, "G"=w2495:sgl, "B"=w2494:sgl)
          n1288 = Or(x=w2525, y=w2526) -> (x .or. y?=w2521:bool)
          n1289 = Subtract(x=w2516, y=w2515) -> (x-y=w2500:sgl)
          n1290 = local write "MP HP"(w2491) -> ()
          n1291 = Subtract(x=w2514, y=w2513) -> (x-y=w2501:sgl)
          n1292 = Absolute Value(x=w2501) -> (abs(x)=w2509:sgl)
          n1293 = Absolute Value(x=w2500) -> (abs(x)=w2512:sgl)
          n1294 = To Long Integer(number=w2503) -> (32bit integer=w2502:i32)
          n1295 = Less?(x=w2509, y=560.0) -> (x < y?=w2507:bool)
          n1296 = Less?(x=w2512, y=840.0) -> (x < y?=w2506:bool)
          n1297 = And(x=w2506, y=w2507) -> (x .and. y?=w2508:bool)
          n1298 = And(x=w2508, y=w2521) -> (x .and. y?=w2522:bool)
          n1299 = case shown="True" w2522 {
            tunnel: [w2527 w2534] -> w2504
            tunnel: w2505 -> [w2527 w2537]
            tunnel: w2502 -> [_ w2540]
            tunnel: w2501 -> [_ w2539]
            tunnel: w2500 -> [_ w2538]
            tunnel: w2499 -> [_ w2536]
            tunnel: w2498 -> [_ w2535]
            tunnel: w2497 -> [_ w2533]
            tunnel: w2496 -> [_ w2532]
            tunnel: w2495 -> [_ w2531]
            tunnel: w2494 -> [_ w2530]
            tunnel: w2493 -> [_ w2529]
            tunnel: w2492 -> [_ w2528]
            frame False {
            }
            frame True {
              n1300 = case shown="0, Default" w2540 {
                tunnel: w2539 -> [w2548 w2721 w2736 w2755 w2771]
                tunnel: w2538 -> [w2547 w2720 w2735 w2754 w2770]
                tunnel: w2537 -> [w2545 w2718 w2733 w2749 w2765]
                tunnel: w2536 -> [w2543 _ _ _ _]
                tunnel: w2535 -> [w2546 _ _ w2746 w2763]
                tunnel: [w2541 w2712 w2724 w2743 w2758] -> w2534
                tunnel: w2533 -> [_ w2711 w2728 _ _]
                tunnel: w2532 -> [_ w2710 w2727 w2753 w2769]
                tunnel: w2531 -> [_ w2709 w2726 w2752 w2768]
                tunnel: w2530 -> [_ w2708 w2725 w2751 w2767]
                tunnel: w2529 -> [_ _ _ w2740 w2760]
                tunnel: w2528 -> [_ _ _ w2739 w2759]
                frame 0, Default {
                  n1301 = Greater?(x=w2543, y=0.0) -> (0:w2544:bool)
                  n1302 = case shown="False" w2544 {
                    tunnel: w2548 -> [w2605 w2705]
                    tunnel: w2547 -> [w2604 w2704]
                    tunnel: w2543 -> [w2602 w2702]
                    tunnel: [w2571 w2671] -> w2541
                    tunnel: w2546 -> [w2559 w2608]
                    tunnel: w2545 -> [w2551 w2648]
                    frame True {
                      w2562 = 10.0 ("height")
                      w2563 = 55.0 ("width")
                      w2573 = i16 9 ("radius")
                      w2583 = i16 9 ("radius")
                      w2592 = i16 30 ("radius")
                      # "Draw two hand on player"
                      # "Draw the weapon on hand"
                      # "The color of player base on the HP points"
                      n1303 = Add(x=w2604, y=640.0) -> (x+y=w2557:dbl)
                      n1304 = Add(x=w2605, y=360.0) -> (x+y=w2554:dbl)
                      n1305 = Divide(x=w2602, y=4.0) -> (x/y=w2596:dbl)
                      n1306 = call "rotation matrix.vi"("angle"=w2559, "y"=0.0, "x"=-55.0) -> ("new y"=w2555:dbl, "new x"=w2558:dbl)
                      n1307 = Add(x=w2555, y=w2554) -> (x+y=w2553:dbl)
                      n1308 = Add(x=w2558, y=w2557) -> (x+y=w2556:dbl)
                      n1309 = Bundle(w2557, w2554) -> (w2591:cluster{dbl, dbl})  [unwired: 1 in]
                      n1310 = Add(x=w2596, y=180.0) -> (x+y=w2600:dbl)
                      n1311 = Add(x=w2596, y=140.0) -> (x+y=w2599:dbl)
                      n1312 = Add(x=w2596, y=85.0) -> (x+y=w2598:dbl)
                      n1313 = call "draw rotated rectangle.vi"("fill"=TRUE, "Color Box"=u32 3684408, "angle"=w2559, "2D Picture"=w2551, "height"=w2562, "width"=w2563, "y"=w2553, "x"=w2556) -> ("new picture"=w2564:picture)  [unwired: 3 in]
                      n1314 = call <vilib>:"RGB to Color.vi"("B"=w2598, "G"=w2599, "R"=w2600) -> ("Color"=w2568:u32)
                      n1315 = call "draw rotated rectangle.vi"("fill"=FALSE, "Color Box"=u32 0, "angle"=w2559, "2D Picture"=w2564, "height"=w2562, "width"=w2563, "y"=w2553, "x"=w2556) -> ("new picture"=w2549:picture)  [unwired: 3 in]
                      n1316 = call <vilib>:"Draw Circle by Radius.vi"("color(black)"=w2568, "fill?(F)"=TRUE, "pixel center"=w2591, "radius"=w2592, "picture"=w2549) -> ("new picture"=w2593:picture)  [unwired: 6 in]
                      n1317 = call <vilib>:"Draw Circle by Radius.vi"("pixel center"=w2591, "radius"=w2592, "picture"=w2593) -> ("new picture"=w2550:picture)  [unwired: 8 in]
                      n1318 = call "rotation matrix.vi"("angle"=w2559, "y"=-8.0, "x"=-35.0) -> ("new y"=w2584:dbl, "new x"=w2585:dbl)
                      n1319 = Add(x=w2554, y=w2584) -> (x+y=w2587:dbl)
                      n1320 = Add(x=w2557, y=w2585) -> (x+y=w2588:dbl)
                      n1321 = Bundle(w2588, w2587) -> (w2581:cluster{dbl, dbl})  [unwired: 1 in]
                      n1322 = call <vilib>:"Draw Circle by Radius.vi"("color(black)"=w2568, "fill?(F)"=TRUE, "pixel center"=w2581, "radius"=w2583, "picture"=w2550) -> ("new picture"=w2582:picture)  [unwired: 6 in]
                      n1323 = call "rotation matrix.vi"("angle"=w2559, "y"=8.0, "x"=-40.0) -> ("new y"=w2569:dbl, "new x"=w2570:dbl)
                      n1324 = call <vilib>:"Draw Circle by Radius.vi"("pixel center"=w2581, "radius"=w2583, "picture"=w2582) -> ("new picture"=w2572:picture)  [unwired: 8 in]
                      n1325 = Add(x=w2557, y=w2570) -> (x+y=w2575:dbl)
                      n1326 = Add(x=w2554, y=w2569) -> (x+y=w2576:dbl)
                      n1327 = Bundle(w2575, w2576) -> (w2574:cluster{dbl, dbl})  [unwired: 1 in]
                      n1328 = call <vilib>:"Draw Circle by Radius.vi"("color(black)"=w2568, "fill?(F)"=TRUE, "pixel center"=w2574, "radius"=w2573, "picture"=w2572) -> ("new picture"=w2580:picture)  [unwired: 6 in]
                      n1329 = call <vilib>:"Draw Circle by Radius.vi"("pixel center"=w2574, "radius"=w2573, "picture"=w2580) -> ("new picture"=w2571:picture)  [unwired: 8 in]
                    }
                    frame False {
                      w2662 = 10.0 ("height")
                      w2663 = 55.0 ("width")
                      w2673 = i16 9 ("radius")
                      w2683 = i16 9 ("radius")
                      w2692 = i16 30 ("radius")
                      # "Draw two hand on player"
                      # "Draw the weapon on hand"
                      # "The color of player base on the HP points"
                      n1330 = Add(x=w2704, y=640.0) -> (x+y=w2611:dbl)
                      n1331 = Add(x=w2705, y=360.0) -> (x+y=w2612:dbl)
                      n1332 = call "rotation matrix.vi"("angle"=w2608, "y"=-5.0, "x"=-22.0 ("y")) -> ("new y"=w2639:dbl, "new x"=w2640:dbl)
                      n1333 = Add(x=w2611, y=w2640) -> (x+y=w2646:dbl)
                      n1334 = Add(x=w2612, y=w2639) -> (x+y=w2645:dbl)
                      n1335 = Divide(x=w2702, y=4.0) -> (x/y=w2696:dbl)
                      n1336 = Bundle(w2646, w2645) -> (w2638:cluster{dbl, dbl})  [unwired: 1 in]
                      n1337 = call <vilib>:"Draw Circle by Radius.vi"("color(black)"=u32 16711680, "fill?(F)"=TRUE, "pixel center"=w2638, "radius"=i16 24, "picture"=w2648) -> ("new picture"=w2631:picture)  [unwired: 6 in]
                      n1338 = Bundle(w2611, w2612) -> (w2691:cluster{dbl, dbl})  [unwired: 1 in]
                      n1339 = Add(x=w2608, y=0.5) -> (x+y=w2628:dbl)
                      n1340 = Add(x=w2696, y=180.0) -> (x+y=w2700:dbl)
                      n1341 = call "rotation matrix.vi"("angle"=w2628, "y"=5.0, "x"=-24.0) -> ("new y"=w2625:dbl, "new x"=w2626:dbl)
                      n1342 = Add(x=w2696, y=140.0) -> (x+y=w2699:dbl)
                      n1343 = Add(x=w2696, y=85.0) -> (x+y=w2698:dbl)
                      n1344 = Add(x=w2611, y=w2626) -> (x+y=w2636:dbl)
                      n1345 = Add(x=w2612, y=w2625) -> (x+y=w2635:dbl)
                      n1346 = Add(x=w2608, y=-0.1) -> (x+y=w2651:dbl)
                      n1347 = call <vilib>:"RGB to Color.vi"("B"=w2698, "G"=w2699, "R"=w2700) -> ("Color"=w2668:u32)
                      n1348 = Add(x=w2608, y=-1.75) -> (x+y=w2609:dbl)
                      n1349 = Bundle(w2636, w2635) -> (w2632:cluster{dbl, dbl})  [unwired: 1 in]
                      n1350 = call <vilib>:"Draw Circle by Radius.vi"("color(black)"=u32 16711680, "fill?(F)"=TRUE, "pixel center"=w2632, "radius"=i16 20, "picture"=w2631) -> ("new picture"=w2618:picture)  [unwired: 6 in]
                      n1351 = call "rotation matrix.vi"("angle"=w2609, "y"=5.0, "x"=-27.0) -> ("new y"=w2613:dbl, "new x"=w2614:dbl)
                      n1352 = call "rotation matrix.vi"("angle"=w2651, "y"=-8.0, "x"=-40.0) -> ("new y"=w2684:dbl, "new x"=w2685:dbl)
                      n1353 = Add(x=w2611, y=w2614) -> (x+y=w2623:dbl)
                      n1354 = Add(x=w2612, y=w2613) -> (x+y=w2622:dbl)
                      n1355 = Bundle(w2623, w2622) -> (w2619:cluster{dbl, dbl})  [unwired: 1 in]
                      n1356 = call <vilib>:"Draw Circle by Radius.vi"("color(black)"=u32 16711680, "fill?(F)"=TRUE, "pixel center"=w2619, "radius"=i16 7, "picture"=w2618) -> ("new picture"=w2617:picture)  [unwired: 6 in]
                      n1357 = Add(x=w2612, y=w2684) -> (x+y=w2687:dbl)
                      n1358 = Add(x=w2611, y=w2685) -> (x+y=w2688:dbl)
                      n1359 = Bundle(w2688, w2687) -> (w2681:cluster{dbl, dbl})  [unwired: 1 in]
                      n1360 = Add(x=w2608, y=0.5) -> (x+y=w2652:dbl)
                      n1361 = call "rotation matrix.vi"("angle"=w2608, "y"=10.0, "x"=-50.0) -> ("new y"=w2669:dbl, "new x"=w2670:dbl)
                      n1362 = call "rotation matrix.vi"("angle"=w2608, "y"=0.0, "x"=-55.0) -> ("new y"=w2657:dbl, "new x"=w2659:dbl)
                      n1363 = Add(x=w2657, y=w2612) -> (x+y=w2656:dbl)
                      n1364 = Add(x=w2659, y=w2611) -> (x+y=w2658:dbl)
                      n1365 = Add(x=w2611, y=w2670) -> (x+y=w2675:dbl)
                      n1366 = Add(x=w2612, y=w2669) -> (x+y=w2676:dbl)
                      n1367 = call "draw rotated rectangle.vi"("fill"=TRUE, "Color Box"=u32 3684408, "angle"=w2652, "2D Picture"=w2617, "height"=w2662, "width"=w2663, "y"=w2656, "x"=w2658) -> ("new picture"=w2664:picture)  [unwired: 3 in]
                      n1368 = Bundle(w2675, w2676) -> (w2674:cluster{dbl, dbl})  [unwired: 1 in]
                      n1369 = call "draw rotated rectangle.vi"("fill"=FALSE, "Color Box"=u32 0, "angle"=w2652, "2D Picture"=w2664, "height"=w2662, "width"=w2663, "y"=w2656, "x"=w2658) -> ("new picture"=w2653:picture)  [unwired: 3 in]
                      n1370 = call <vilib>:"Draw Circle by Radius.vi"("color(black)"=w2668, "fill?(F)"=TRUE, "pixel center"=w2691, "radius"=w2692, "picture"=w2653) -> ("new picture"=w2693:picture)  [unwired: 6 in]
                      n1371 = call <vilib>:"Draw Circle by Radius.vi"("pixel center"=w2691, "radius"=w2692, "picture"=w2693) -> ("new picture"=w2654:picture)  [unwired: 8 in]
                      n1372 = call <vilib>:"Draw Circle by Radius.vi"("color(black)"=w2668, "fill?(F)"=TRUE, "pixel center"=w2681, "radius"=w2683, "picture"=w2654) -> ("new picture"=w2682:picture)  [unwired: 6 in]
                      n1373 = call <vilib>:"Draw Circle by Radius.vi"("pixel center"=w2681, "radius"=w2683, "picture"=w2682) -> ("new picture"=w2672:picture)  [unwired: 8 in]
                      n1374 = call <vilib>:"Draw Circle by Radius.vi"("color(black)"=w2668, "fill?(F)"=TRUE, "pixel center"=w2674, "radius"=w2673, "picture"=w2672) -> ("new picture"=w2680:picture)  [unwired: 6 in]
                      n1375 = call <vilib>:"Draw Circle by Radius.vi"("pixel center"=w2674, "radius"=w2673, "picture"=w2680) -> ("new picture"=w2671:picture)  [unwired: 8 in]
                    }
                  }
                }
                frame 1 {
                  n1376 = Add(x=w2720, y=640.0) -> (x+y=w2714:dbl)
                  n1377 = Add(x=w2721, y=360.0) -> (x+y=w2713:dbl)
                  n1378 = Bundle(w2714, w2713) -> (w2716:cluster{dbl, dbl})  [unwired: 1 in]
                  n1379 = call <vilib>:"RGB to Color.vi"("B"=w2708, "G"=w2709, "R"=w2710) -> ("Color"=w2715:u32)
                  n1380 = call <vilib>:"Draw Circle by Radius.vi"("color(black)"=w2715, "fill?(F)"=TRUE, "pixel center"=w2716, "radius"=w2711, "picture"=w2718) -> ("new picture"=w2717:picture)  [unwired: 6 in]
                  n1381 = call <vilib>:"Draw Circle by Radius.vi"("pixel center"=w2716, "radius"=w2711, "picture"=w2717) -> ("new picture"=w2712:picture)  [unwired: 8 in]
                }
                frame 3 {
                  n1382 = Add(x=w2735, y=640.0) -> (x+y=w2730:dbl)
                  n1383 = Add(x=w2736, y=360.0) -> (x+y=w2729:dbl)
                  n1384 = Bundle(w2730, w2729) -> (w2732:cluster{dbl, dbl})  [unwired: 1 in]
                  n1385 = call <vilib>:"RGB to Color.vi"("B"=w2725, "G"=w2726, "R"=w2727) -> ("Color"=w2731:u32)
                  n1386 = call <vilib>:"Draw Circle by Radius.vi"("color(black)"=w2731, "fill?(F)"=TRUE, "pixel center"=w2732, "radius"=w2728, "picture"=w2733) -> ("new picture"=w2724:picture)  [unwired: 6 in]
                }
                frame 2 {
                  n1387 = Add(x=w2754, y=640.0) -> (x+y=w2742:dbl)
                  n1388 = Add(x=w2755, y=360.0) -> (x+y=w2741:dbl)
                  n1389 = call <vilib>:"RGB to Color.vi"("B"=w2751, "G"=w2752, "R"=w2753) -> ("Color"=w2748:u32)
                  n1390 = call "draw rotated rectangle.vi"("fill"=TRUE, "Color Box"=w2748, "angle"=w2746, "2D Picture"=w2749, "height"=w2739, "width"=w2740, "y"=w2741, "x"=w2742) -> ("new picture"=w2744:picture)  [unwired: 3 in]
                  n1391 = call "draw rotated rectangle.vi"("fill"=FALSE, "Color Box"=u32 0, "angle"=w2746, "2D Picture"=w2744, "height"=w2739, "width"=w2740, "y"=w2741, "x"=w2742) -> ("new picture"=w2743:picture)  [unwired: 3 in]
                }
                frame 4 {
                  n1392 = Add(x=w2770, y=640.0) -> (x+y=w2762:dbl)
                  n1393 = Add(x=w2771, y=360.0) -> (x+y=w2761:dbl)
                  n1394 = call <vilib>:"RGB to Color.vi"("B"=w2767, "G"=w2768, "R"=w2769) -> ("Color"=w2764:u32)
                  n1395 = call "draw rotated rectangle.vi"("fill"=TRUE, "Color Box"=w2764, "angle"=w2763, "2D Picture"=w2765, "height"=w2759, "width"=w2760, "y"=w2761, "x"=w2762) -> ("new picture"=w2758:picture)  [unwired: 3 in]
                }
              }
            }
          }
        }
        n1396 = local read "Player Bullets"() -> (w2305:i32[])
        n1397 = local read "My NetPlayer number"() -> (w2271:i32)
        n1398 = local read "Player Bullets Reload"() -> (w2302:i32[])
        n1399 = Index Array(array=w2305, index=w2271) -> (element=w2304:i32)
        n1400 = call <vilib>:"High Resolution Relative Seconds.vi"() -> ("relative seconds"=w2324:dbl)
        n1401 = Number To Decimal String(number=w2304) -> (decimal integer string=w2303:string)  [unwired: 1 in]
        n1402 = feedback #5(u32 0 ("millisecond timer value")) -> (w2325:dbl)
        n1403 = feedback-in #5(w2324) -> ()
        n1404 = Index Array(array=w2302, index=w2271) -> (element=w2298:i32)
        n1405 = Subtract(x=w2324, y=w2325) -> (x-y=w2326:dbl)
        n1406 = call <vilib>:"Draw Text at Point.vi"("[user-specified font]"=T14 {"Font Name:"="Arial", "Size"=36, "Strikeout?"=FALSE, "Italic?"=FALSE, "Underline?"=FALSE, "Outline?"=FALSE, "Shadow?"=TRUE, "Bold?"=TRUE}, "text color(black)"=u32 0, "desired font(Application)"=T13."User-specified Font", "text"=w2303, "alignment(left, top)"=T15 {"horizontal"=enum."left", "vertical"=enum."top"}, "origin"=cluster{"x":i16, "y":i16} {"x"=860, "y"=635}, "picture"=w2311) -> ("new picture"=w2299:picture)  [unwired: 3 in, 1 out]
        n1407 = Divide(x=1.0, y=w2326) -> (x/y=w2321:dbl)
        n1408 = local write "FPS"(w2321) -> ()
        n1409 = Greater?(x=w2298, y=4) -> (0:w2300:bool)
        n1410 = case shown="True" w2300 {
          tunnel: [w2427 w2444] -> w2296
          tunnel: w2299 -> [w2427 w2449]
          tunnel: w2298 -> [_ w2442]
          frame False {
          }
          frame True {
            w2439 = cluster{"x":i16, "y":i16} {"x"=640, "y"=580} ("origin")
            n1411 = Divide(x=w2442, y=120) -> (x/y=w2429:dbl)
            n1412 = Multiply(x=w2429, y=360.0) -> (x*y=w2436:dbl)
            n1413 = call <vilib>:"Draw Circle by Radius.vi"("arc size(360)"=w2436, "color(black)"=u32 13816530, "fill?(F)"=TRUE, "pixel center"=w2439, "radius"=i16 50, "picture"=w2449) -> ("new picture"=w2443:picture)  [unwired: 5 in]
            n1414 = Multiply(x=w2429, y=2.0) -> (x*y=w2430:dbl)
            n1415 = Number To Fractional String(number=w2430, precision (6)=i16 1) -> (F-format string=w2432:string)  [unwired: 2 in]
            n1416 = Concatenate Strings("Reloading...\n      ", w2432) -> (w2434:string)
            n1417 = call <vilib>:"Draw Text at Point.vi"("[user-specified font]"=T14 {"Font Name:"="Arial", "Size"=24, "Strikeout?"=FALSE, "Italic?"=FALSE, "Underline?"=FALSE, "Outline?"=FALSE, "Shadow?"=TRUE, "Bold?"=TRUE}, "text color(black)"=u32 0, "desired font(Application)"=T13."User-specified Font", "text"=w2434, "alignment(left, top)"=T15 {"horizontal"=enum."center", "vertical"=enum."center"}, "origin"=w2439, "picture"=w2443) -> ("new picture"=w2444:picture)  [unwired: 3 in, 1 out]
          }
        }
        n1418 = local read "STOP (會卡住)"() -> (w2327:bool)
        n1419 = local read "Player info"() -> (w2297:T6)
        n1420 = Sort 1D Array(array=w2297) -> (sorted array=w2295:T6)
        n1421 = Reverse 1D Array(array=w2295) -> (reversed array=w2294:T6)
        n1422 = for {
          tunnel: w2294 -> [w2419] mode=indexing
          shift-right: [w2414] -> w2289
          shift-left: w2296 -> [w2420]
          i -> [w2405]
          stop <- w2426 stop-if-true
          n1423 = Unbundle(w2419) -> ("Kills"=w2411:dbl, "Name"=w2412:string)  [unwired: 3 out]
          n1424 = Multiply(x=32, y=w2405) -> (x*y=w2403:i32)
          n1425 = Add(x=24, y=w2403) -> (x+y=w2401:i32)
          n1426 = Bundle(24, w2401) -> (w2409:cluster{i32, i32})  [unwired: 1 in]
          n1427 = call <vilib>:"Draw Text at Point.vi"("[user-specified font]"=T14 {"Font Name:"="Arial", "Size"=24, "Strikeout?"=FALSE, "Italic?"=FALSE, "Underline?"=FALSE, "Outline?"=FALSE, "Shadow?"=TRUE, "Bold?"=TRUE}, "text color(black)"=u32 0, "desired font(Application)"=T13."User-specified Font", "text"=w2412, "alignment(left, top)"=T15 {"horizontal"=enum."left", "vertical"=enum."center"}, "origin"=w2409, "picture"=w2420) -> ("new picture"=w2413:picture)  [unwired: 3 in, 1 out]
          n1428 = Number To Decimal String(number=w2411) -> (decimal integer string=w2410:string)  [unwired: 1 in]
          n1429 = Bundle(210, w2401) -> (w2408:cluster{i32, i32})  [unwired: 1 in]
          n1430 = Greater?(x=w2405, y=3) -> (0:w2426:bool)
          n1431 = call <vilib>:"Draw Text at Point.vi"("[user-specified font]"=T14 {"Font Name:"="Arial", "Size"=24, "Strikeout?"=FALSE, "Italic?"=FALSE, "Underline?"=FALSE, "Outline?"=FALSE, "Shadow?"=TRUE, "Bold?"=TRUE}, "text color(black)"=u32 0, "desired font(Application)"=T13."User-specified Font", "text"=w2410, "alignment(left, top)"=T15 {"horizontal"=enum."left", "vertical"=enum."center"}, "origin"=w2408, "picture"=w2413) -> ("new picture"=w2414:picture)  [unwired: 3 in, 1 out]
        }
        n1432 = local read "Alive number"() -> (w2288:i32)
        n1433 = Number To Decimal String(number=w2288) -> (decimal integer string=w2286:string)  [unwired: 1 in]
        n1434 = Concatenate Strings("Alive: " ("string"), w2286) -> (w2287:string)
        n1435 = call <vilib>:"Draw Text at Point.vi"("[user-specified font]"=T14 {"Font Name:"="Arial", "Size"=42, "Strikeout?"=FALSE, "Italic?"=FALSE, "Underline?"=FALSE, "Outline?"=FALSE, "Shadow?"=TRUE, "Bold?"=TRUE}, "text color(black)"=u32 0, "desired font(Application)"=T13."User-specified Font", "text"=w2287, "alignment(left, top)"=T15 {"horizontal"=enum."left", "vertical"=enum."center"}, "origin"=cluster{"x":i16, "y":i16} {"x"=1080, "y"=40}, "picture"=w2289) -> ("new picture"=w2282:picture)  [unwired: 3 in, 1 out]
        n1436 = local read "MP HP"() -> (w2280:dbl)
        n1437 = Less Or Equal?(x=w2280, y=0.0) -> (x <= y?=w2281:bool)
        n1438 = case shown="True" w2281 {
          tunnel: w2282 -> [w2344 w2371]
          tunnel: [w2344 w2351] -> w2275
          frame False {
          }
          frame True {
            n1439 = local read "My NetPlayer number"() -> (w2345:i32)
            n1440 = local read "Player info"() -> (w2368:T6)
            n1441 = Index Array(array=w2368, index=w2345) -> (element=w2370:T26)
            n1442 = Unbundle(w2370) -> ("Kills"=w2347:dbl, "Rank"=w2353:dbl, "Who Kill Me"=w2369:dbl, "After Kill"=w2348:dbl)  [unwired: 1 out]
            n1443 = call <vilib>:"Draw Text at Point.vi"("[user-specified font]"=T14 {"Font Name:"="Arial", "Size"=56, "Strikeout?"=FALSE, "Italic?"=FALSE, "Underline?"=TRUE, "Outline?"=FALSE, "Shadow?"=TRUE, "Bold?"=TRUE}, "text color(black)"=u32 16711699, "desired font(Application)"=T13."User-specified Font", "text"="你已陣亡!", "alignment(left, top)"=T15 {"horizontal"=enum."center", "vertical"=enum."center"}, "origin"=cluster{"x":i16, "y":i16} {"x"=640, "y"=150}, "picture"=w2371) -> ("new picture"=w2357:picture)  [unwired: 3 in, 1 out]
            n1444 = Index Array(array=w2368, index=w2369) -> (element=w2367:T26)
            n1445 = local write "Background music"(2.0 ("Background music")) -> ()
            n1446 = Unbundle(w2367) -> ("Name"=w2365:string)  [unwired: 4 out]
            n1447 = Concatenate Strings(w2365, " 選擇對你痛下殺手" ("string")) -> (w2358:string)
            n1448 = call <vilib>:"Draw Text at Point.vi"("[user-specified font]"=T14 {"Font Name:"="Arial", "Size"=42, "Strikeout?"=FALSE, "Italic?"=FALSE, "Underline?"=FALSE, "Outline?"=FALSE, "Shadow?"=TRUE, "Bold?"=TRUE}, "text color(black)"=u32 5064, "desired font(Application)"=T13."User-specified Font", "text"=w2358, "alignment(left, top)"=T15 {"horizontal"=enum."center", "vertical"=enum."center"}, "origin"=cluster{"x":i16, "y":i16} {"x"=640, "y"=210}, "picture"=w2357) -> ("new picture"=w2354:picture)  [unwired: 3 in, 1 out]
            n1449 = Less?(x=w2348, y=400.0) -> (x < y?=w2355:bool)
            n1450 = case shown="True" w2355 {
              tunnel: w2354 -> [w2389 w2392]
              tunnel: [w2389 w2391] -> w2352
              tunnel: w2353 -> [_ w2390]
              frame False {
              }
              frame True {
                n1451 = Number To Decimal String(number=w2390) -> (decimal integer string=w2393:string)  [unwired: 1 in]
                n1452 = Concatenate Strings("Rank: " ("text"), w2393) -> (w2394:string)
                n1453 = call <vilib>:"Draw Text at Point.vi"("[user-specified font]"=T14 {"Font Name:"="Arial", "Size"=42, "Strikeout?"=FALSE, "Italic?"=FALSE, "Underline?"=FALSE, "Outline?"=FALSE, "Shadow?"=TRUE, "Bold?"=TRUE}, "text color(black)"=u32 16764482, "desired font(Application)"=T13."User-specified Font", "text"=w2394, "alignment(left, top)"=T15 {"horizontal"=enum."center", "vertical"=enum."center"}, "origin"=cluster{"x":i16, "y":i16} {"x"=450, "y"=270}, "picture"=w2392) -> ("new picture"=w2391:picture)  [unwired: 3 in, 1 out]
              }
            }
            n1454 = Less?(x=w2348, y=200.0) -> (x < y?=w2349:bool)
            n1455 = case shown="True" w2349 {
              tunnel: w2352 -> [w2377 w2380]
              tunnel: [w2377 w2379] -> w2351
              tunnel: w2347 -> [_ w2378]
              frame False {
              }
              frame True {
                n1456 = Number To Decimal String(number=w2378) -> (decimal integer string=w2381:string)  [unwired: 1 in]
                n1457 = Concatenate Strings("Kills: " ("text"), w2381) -> (w2382:string)
                n1458 = call <vilib>:"Draw Text at Point.vi"("[user-specified font]"=T14 {"Font Name:"="Arial", "Size"=42, "Strikeout?"=FALSE, "Italic?"=FALSE, "Underline?"=FALSE, "Outline?"=FALSE, "Shadow?"=TRUE, "Bold?"=TRUE}, "text color(black)"=u32 16735530, "desired font(Application)"=T13."User-specified Font", "text"=w2382, "alignment(left, top)"=T15 {"horizontal"=enum."center", "vertical"=enum."center"}, "origin"=cluster{"x":i16, "y":i16} {"x"=810, "y"=270}, "picture"=w2380) -> ("new picture"=w2379:picture)  [unwired: 3 in, 1 out]
              }
            }
          }
        }
        n1459 = local read "Alive number"() -> (w2278:i32)
        n1460 = Equal?(x=w2278, y=1) -> (x = y?=w2276:bool)
        n1461 = case shown="True" w2276 {
          tunnel: [w2329 w2335] -> w2270
          tunnel: w2275 -> [w2329 w2333]
          frame False {
          }
          frame True {
            n1462 = call <vilib>:"Draw Rectangle.vi"("picture"=w2333, "rect"=T11 {"left"=280, "top"=20, "right"=1000, "bottom"=100}, "fill?(F)"=TRUE, "color(black)"=u32 15395562) -> ("new picture"=w2334:picture)  [unwired: 5 in]
            n1463 = local read "Final Winner"() -> (w2337:string)
            n1464 = Concatenate Strings(w2337, " 取得最終勝利!" ("string")) -> (w2338:string)
            n1465 = call <vilib>:"Draw Text at Point.vi"("[user-specified font]"=T14 {"Font Name:"="Arial", "Size"=56, "Strikeout?"=FALSE, "Italic?"=FALSE, "Underline?"=FALSE, "Outline?"=FALSE, "Shadow?"=TRUE, "Bold?"=TRUE}, "text color(black)"=u32 15715328, "desired font(Application)"=T13."User-specified Font", "text"=w2338, "alignment(left, top)"=T15 {"horizontal"=enum."center", "vertical"=enum."center"}, "origin"=cluster{"x":i16, "y":i16} {"x"=640, "y"=60}, "picture"=w2334) -> ("new picture"=w2335:picture)  [unwired: 3 in, 1 out]
          }
        }
        n1466 = local write "PlayingScene"(w2270) -> ()
      }
    }
  }
